vi "FT10_FPGA_7854R Set Relay Config.vi"(10 "Update Config Enum":T1(ring), 11 "Refnum in":refnum<k20>) -> (3 "Refnum out":refnum<k20>)   [LabVIEW 2024]
uses:
  <vilib>/Utility/error.llb/Error Cluster From Error Code.vi
  <vilib>/rvi/errors/niLvFpgaAdjustHostInterfaceError.vi
  <vilib>/rvi/interface/nirviReadWriteControl/nirviReadWriteControl.xnode
  NiFpgaLv.dll
  <vilib>/rvi/interface/Simulation/niFpgaSimulationCallBeginRW.vi
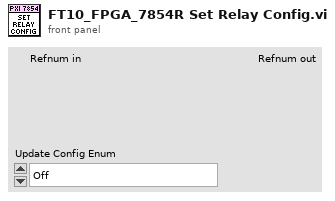
[diagram p1: front panel]
types:
  T1 = enum16{"Off", "Mono1 Relay Config", "Mono2 Relay Config", "Bipolar Relay Config", "Ligasure Relay Config", "Handswitch - Mono1 Cut", "Handswitch - Mono1 Coag", "Handswitch - Mono2 Cut", "Handswitch - Mono2 Coag", "Switch to Triverse Mode", "Switch to Mono2 - 2 button Mode", "Triverse Power 1", "Triverse Power 2", "Triverse Power 3", "Triverse Power 4", "Triverse Power 5", "Handswitch - Triverse Seal", "Handswitch - Triverse Cut", "Handswitch - Triverse Coag"}
  T2 = cluster{"Conn2/DIO_0_7 In":cluster{"Conn2/DIO_0_7 - 75kHz":bool, "Conn2/DIO_0_7 - uSec On":u16, "Conn2/DIO_0_7 In":bool[], "Conn2/DIO_0_7 - uSec Off":u16}, "Conn2/DIO_8_15 In":cluster{"Conn2/DIO_8_15 - 75kHz":bool, "Conn2/DIO_8_15 - uSec On":u16, "Conn2/DIO_8_15 In":bool[], "Conn2/DIO_8_15 - uSec Off":u16}, "Conn2/DIO_16_23 In":cluster{"Conn2/DIO_16_23 - 75kHz":bool, "Conn2/DIO_16_23 - uSec On":u16, "Conn2/DIO_16_23 In":bool[], "Conn2/DIO_16_23 - uSec Off":u16}, "Conn2/DIO_24_31 In":cluster{"Conn2/DIO_24_31 - 75kHz":bool, "Conn2/DIO_24_31 - uSec On":u16, "Conn2/DIO_24_31 In":bool[], "Conn2/DIO_24_31 - uSec Off":u16}, "Conn2/DIO_32_39 In":cluster{"Conn2/DIO_32_39 - 75kHz":bool, "Conn2/DIO_32_39 - uSec On":u16, "Conn2/DIO_32_39 In":bool[], "Conn2/DIO_32_39 - uSec Off":u16}}
  T3 = cluster{"Conn1/DIO_0_7 In":cluster{"Conn1/DIO_0_7 - 75kHz":bool, "Conn1/DIO_0_7 - uSec On":u16, "Conn1/DIO_0_7 In":bool[], "Conn1/DIO_0_7 - uSec Off":u16}, "Conn1/DIO_8_15 In":cluster{"Conn1/DIO_8_15 - 75kHz":bool, "Conn1/DIO_8_15 - uSec On":u16, "Conn1/DIO_8_15 In":bool[], "Conn1/DIO_8_15 - uSec Off":u16}, "Conn1/DIO_16_23 In":cluster{"Conn1/DIO_16_23 - 75kHz":bool, "Conn1/DIO_16_23 - uSec On":u16, "Conn1/DIO_16_23 In":bool[], "Conn1/DIO_16_23 - uSec Off":u16}, "Conn1/DIO_24_31 In":cluster{"Conn1/DIO_24_31 - 75kHz":bool, "Conn1/DIO_24_31 - uSec On":u16, "Conn1/DIO_24_31 In":bool[], "Conn1/DIO_24_31 - uSec Off":u16}, "Conn1/DIO_32_39 In":cluster{"Conn1/DIO_32_39 - 75kHz":bool, "Conn1/DIO_32_39 - uSec On":u16, "Conn1/DIO_32_39 In":bool[], "Conn1/DIO_32_39 - uSec Off":u16}}
  T4 = cluster{"Conn0/DIO_0_7 In":cluster{"Conn0/DIO_0_7 - 75kHz":bool, "Conn0/DIO_0_7 - uSec On":u16, "Conn0/DIO_0_7 In":bool[], "Conn0/DIO_0_7 - uSec Off":u16}, "Conn0/DIO_8_15 In":cluster{"Conn0/DIO_8_15 - 75kHz":bool, "Conn0/DIO_8_15 - uSec On":u16, "Conn0/DIO_8_15 In":bool[], "Conn0/DIO_8_15 - uSec Off":u16}}
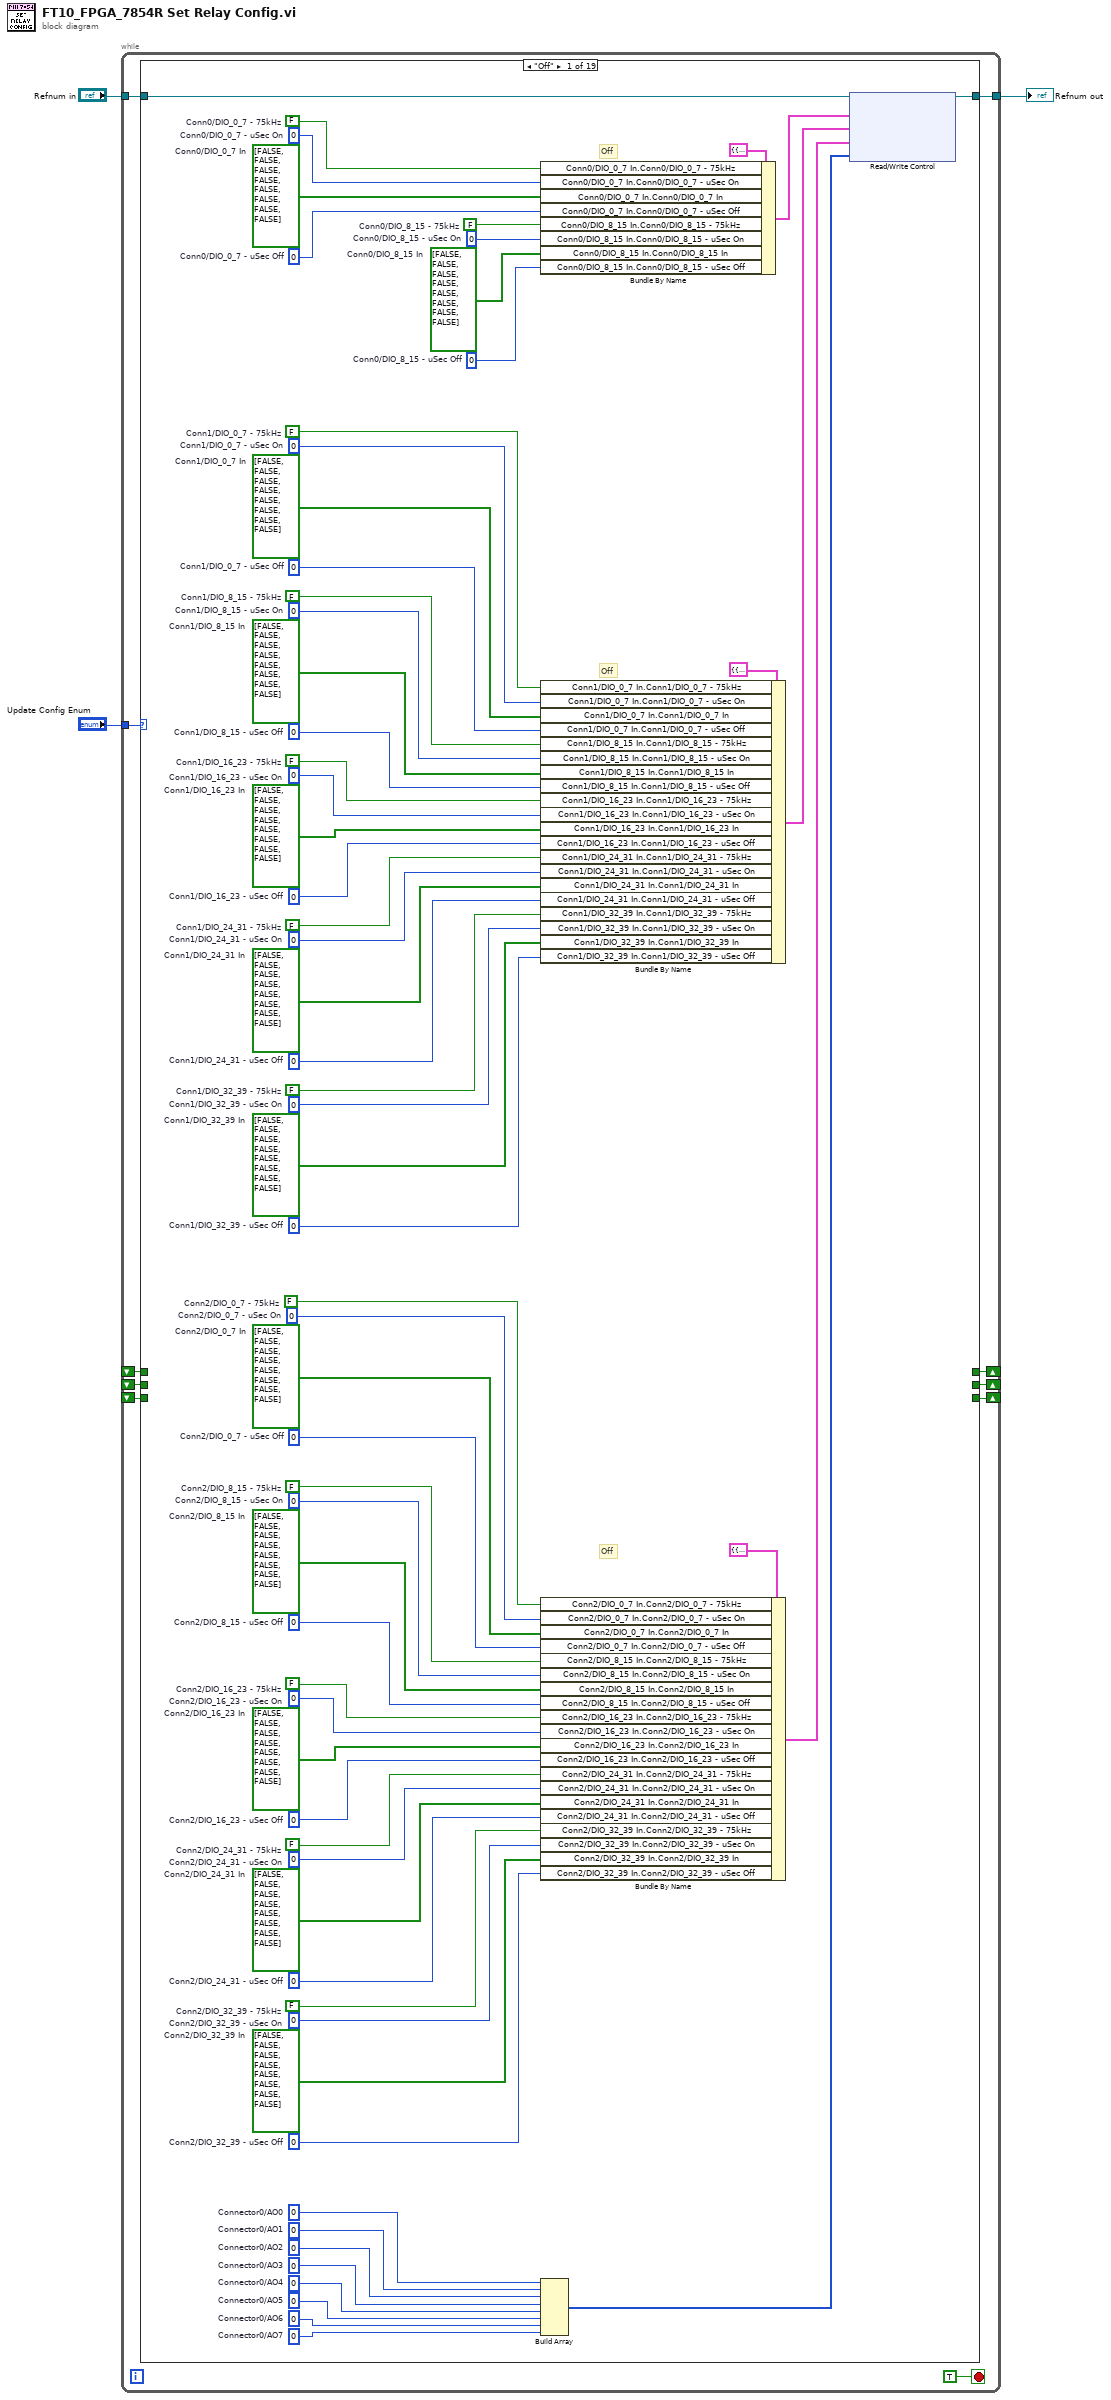
[diagram p0: block diagram]
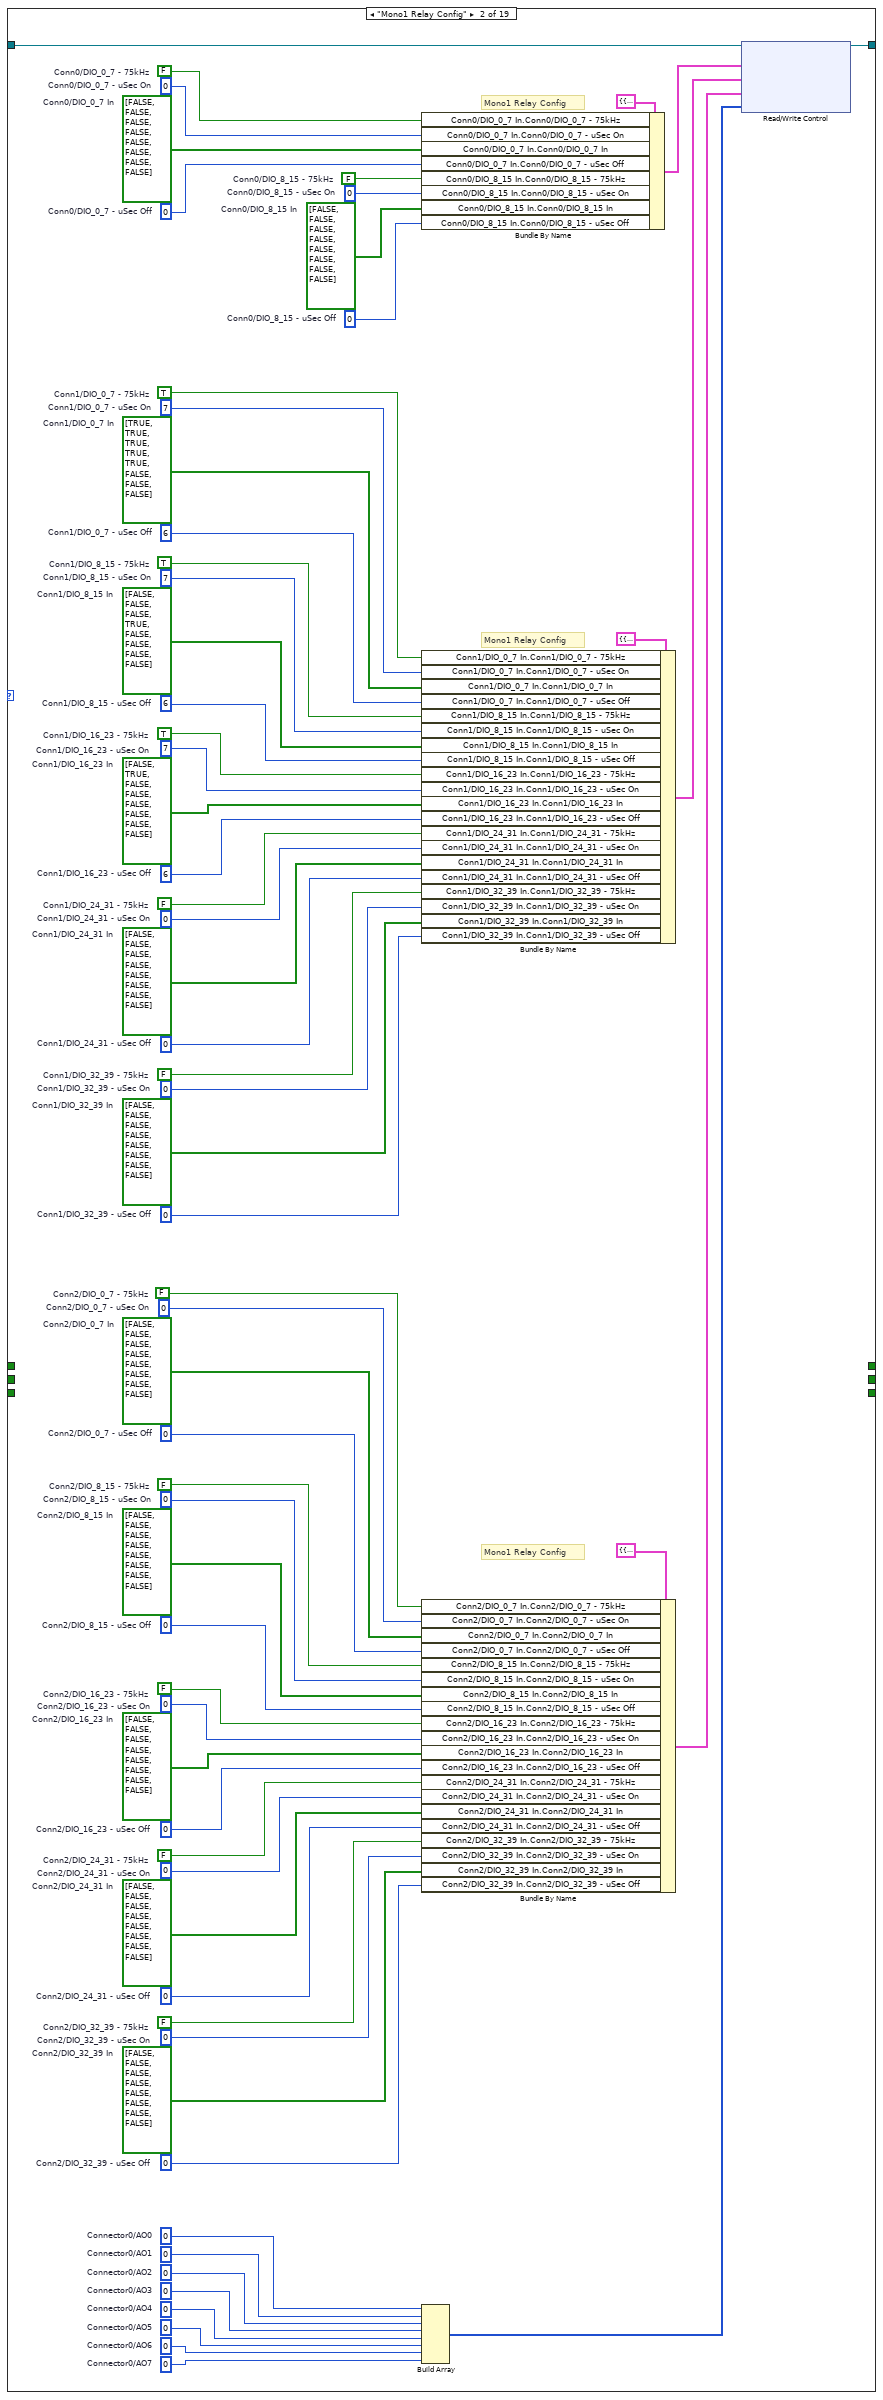
[diagram p2: hidden frame]
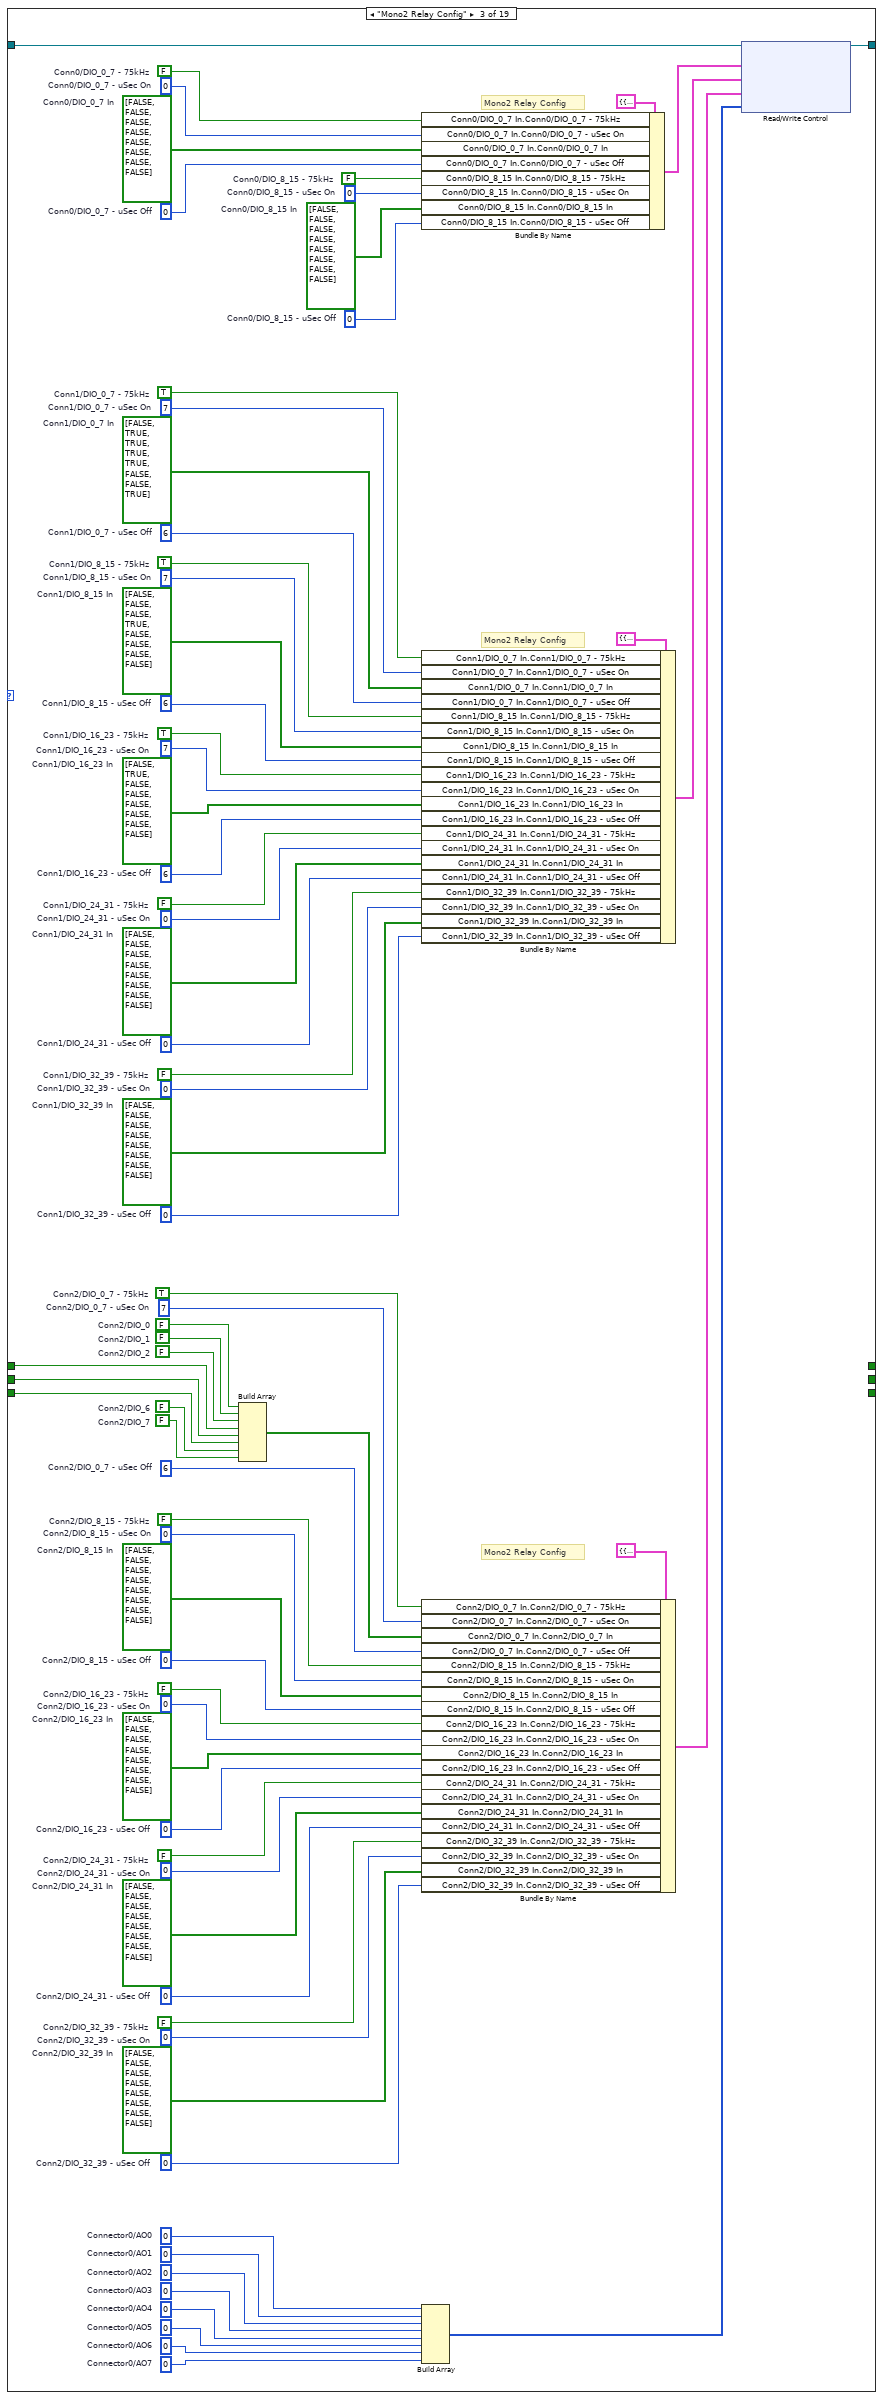
[diagram p3: hidden frame]
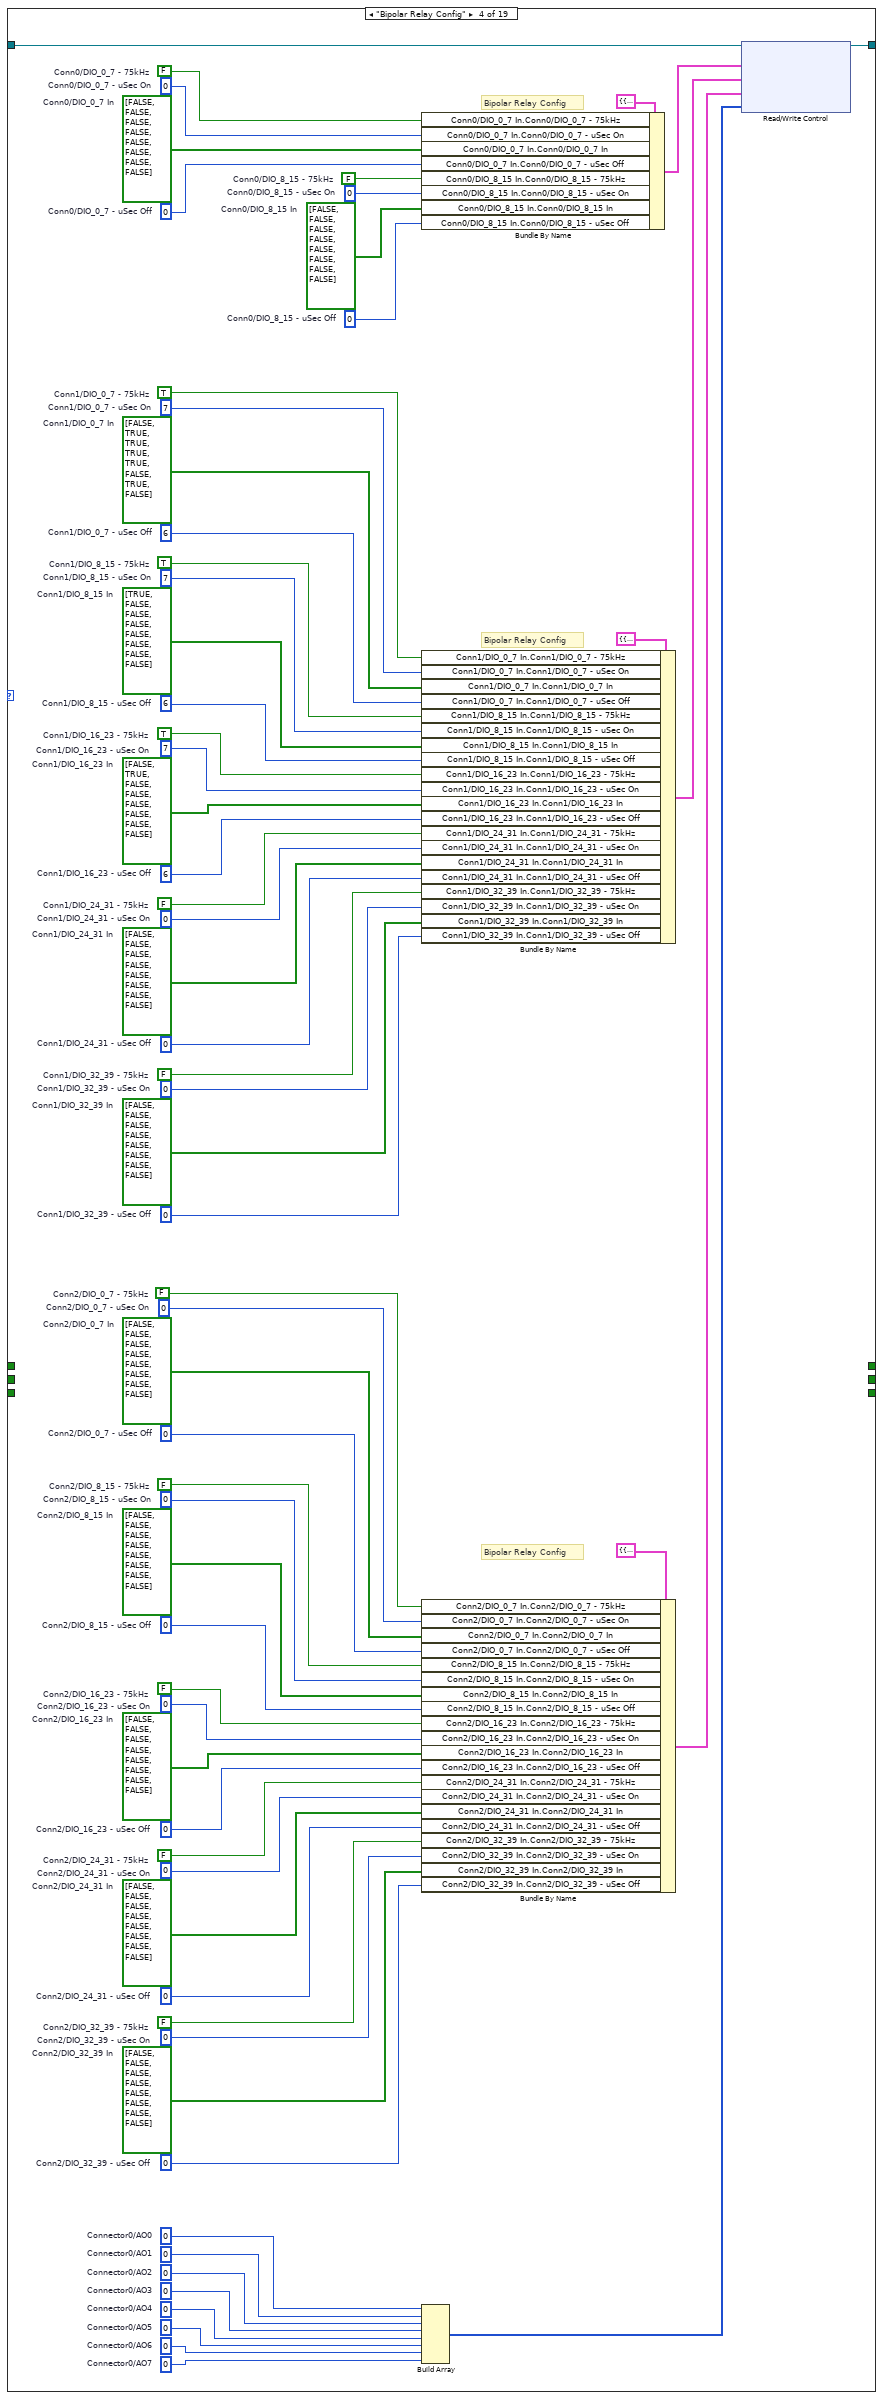
[diagram p4: hidden frame]
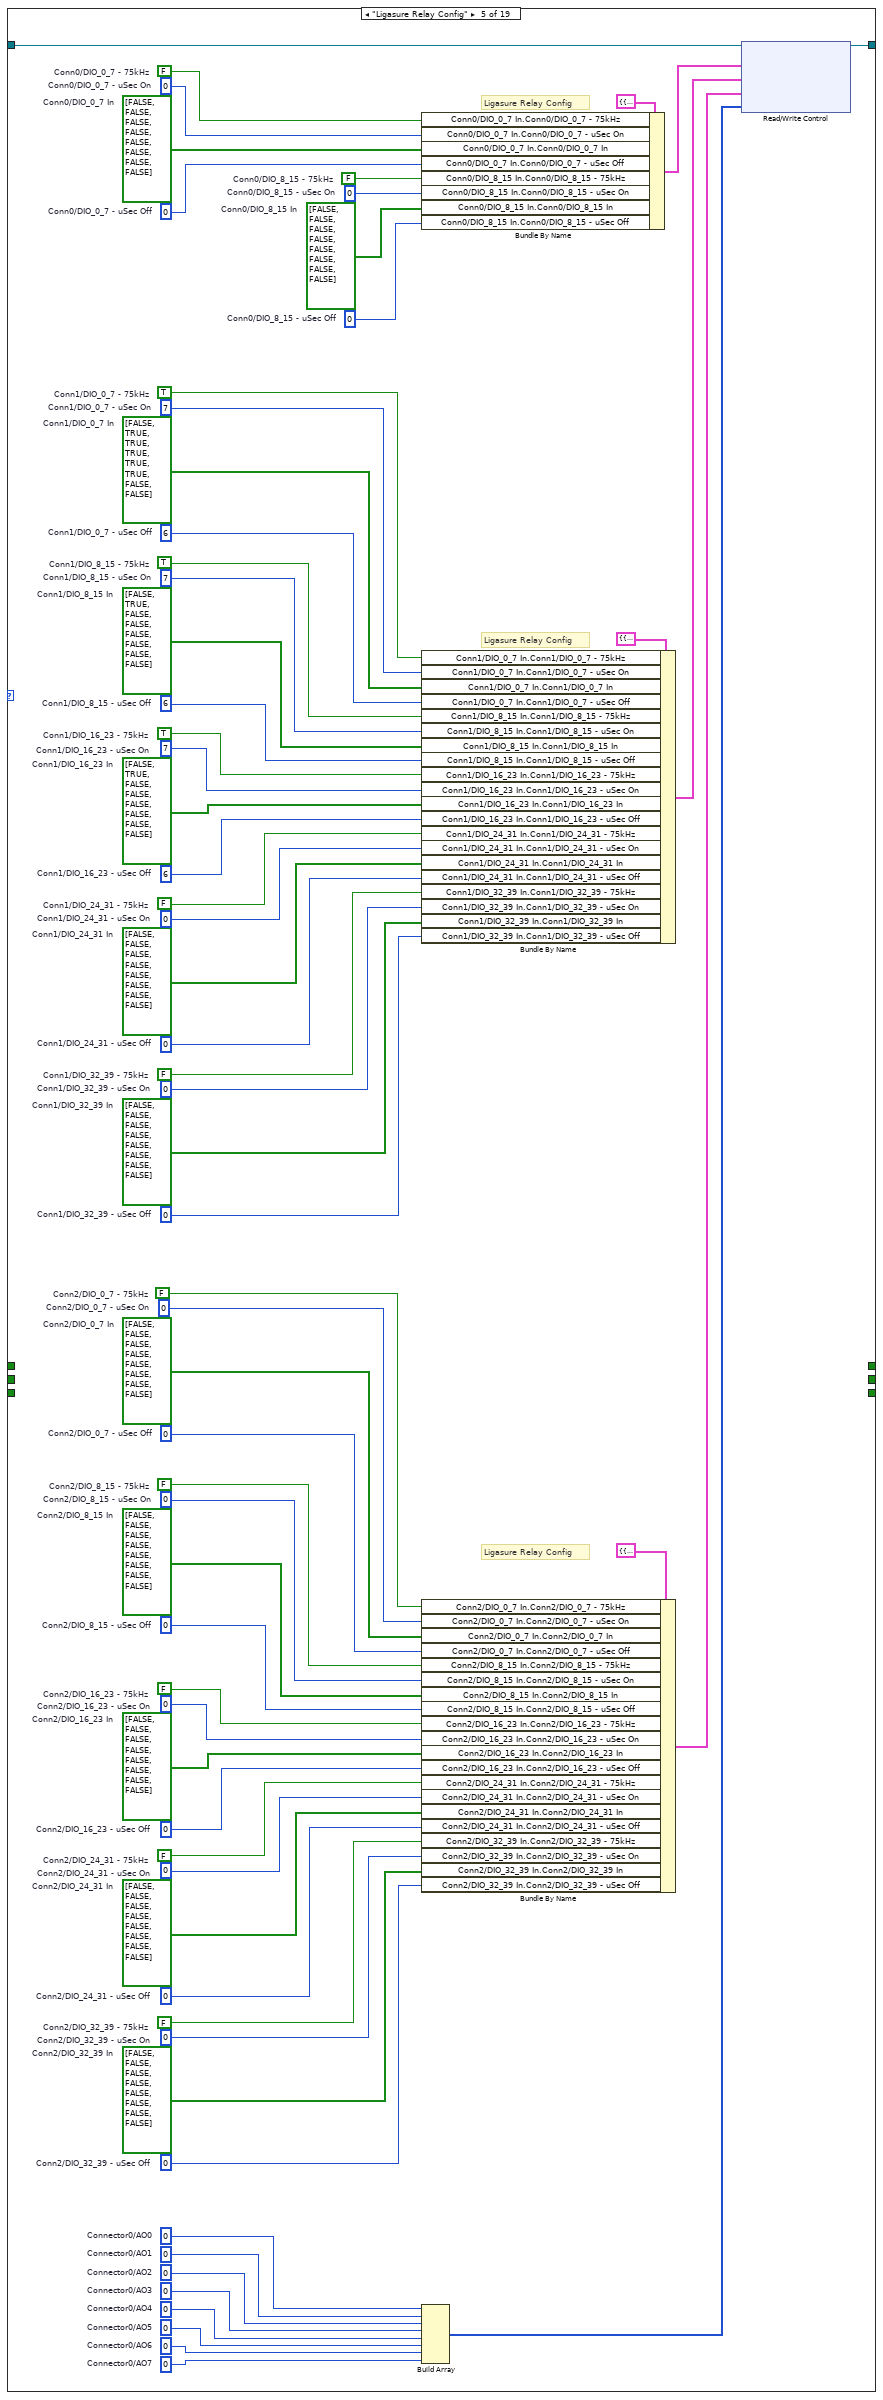
[diagram p5: hidden frame]
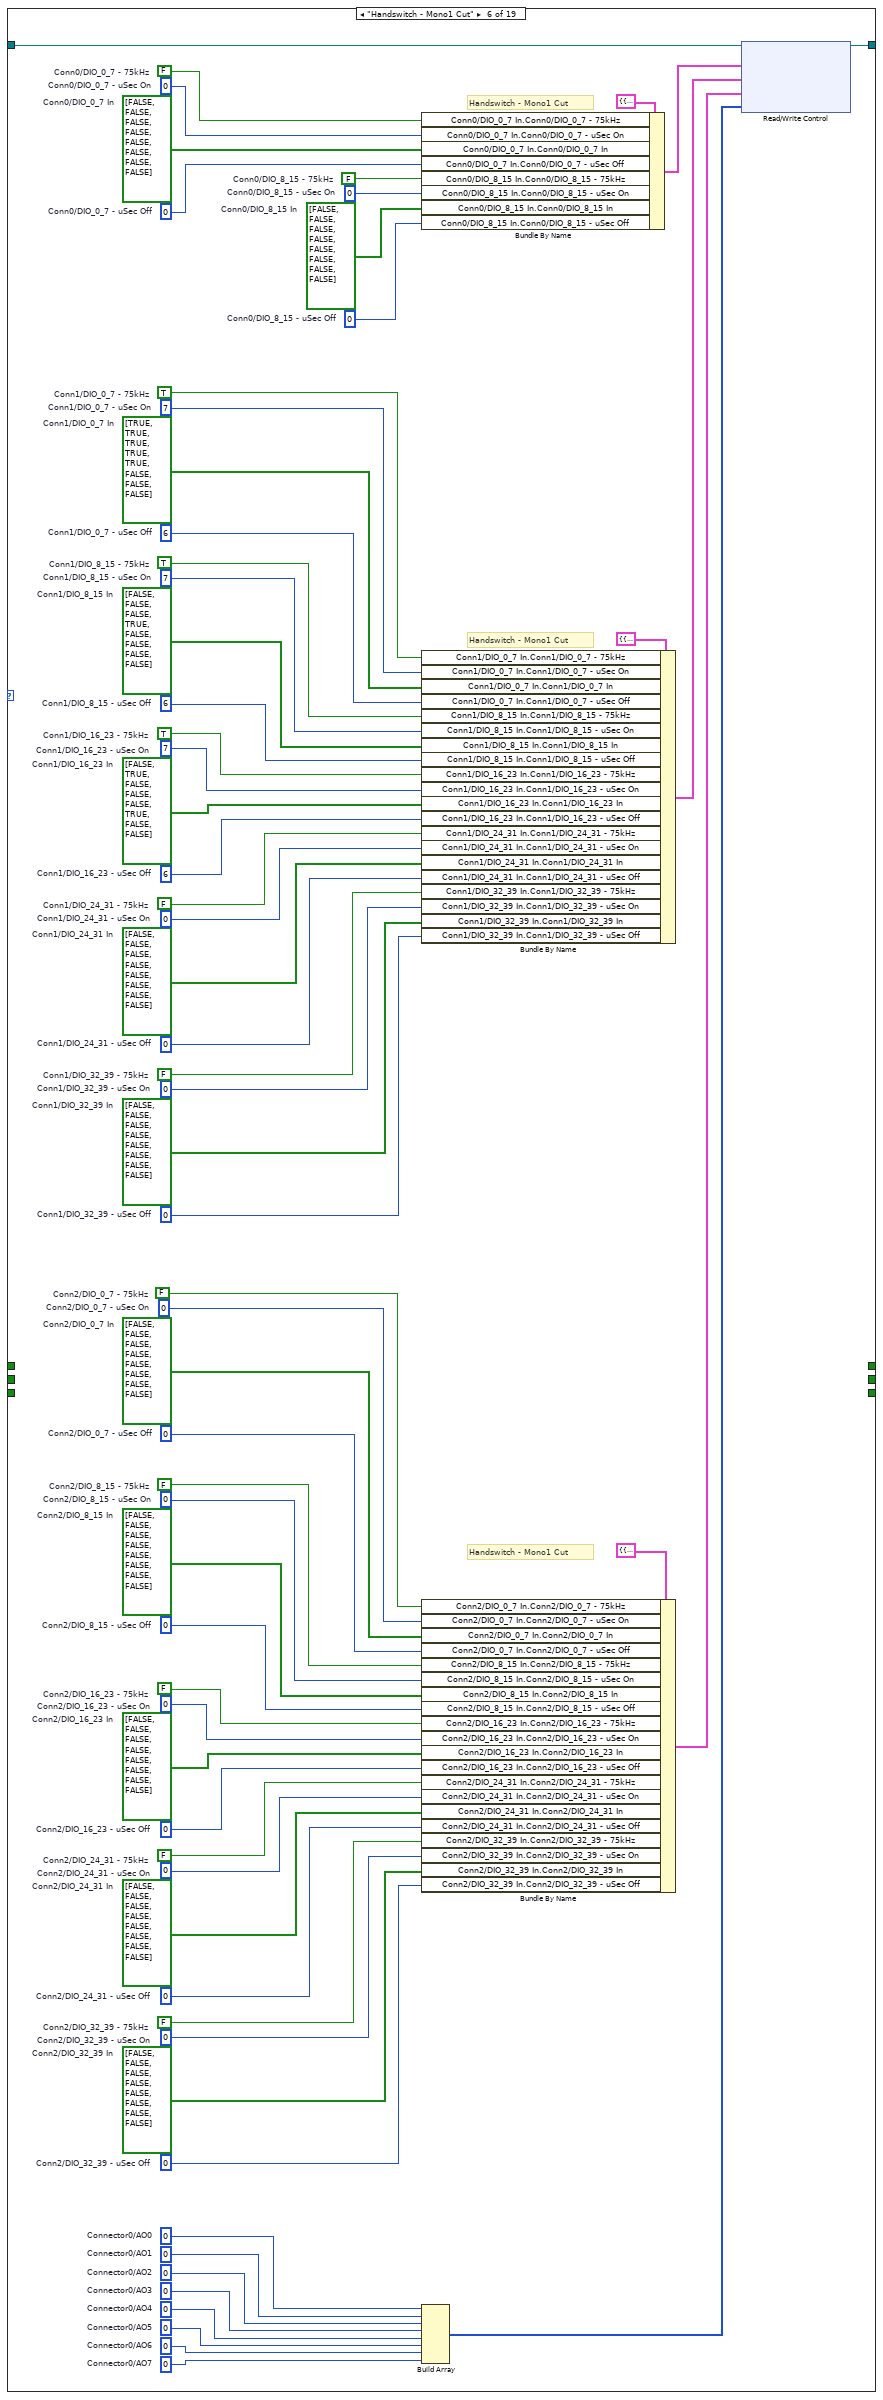
[diagram p6: hidden frame]
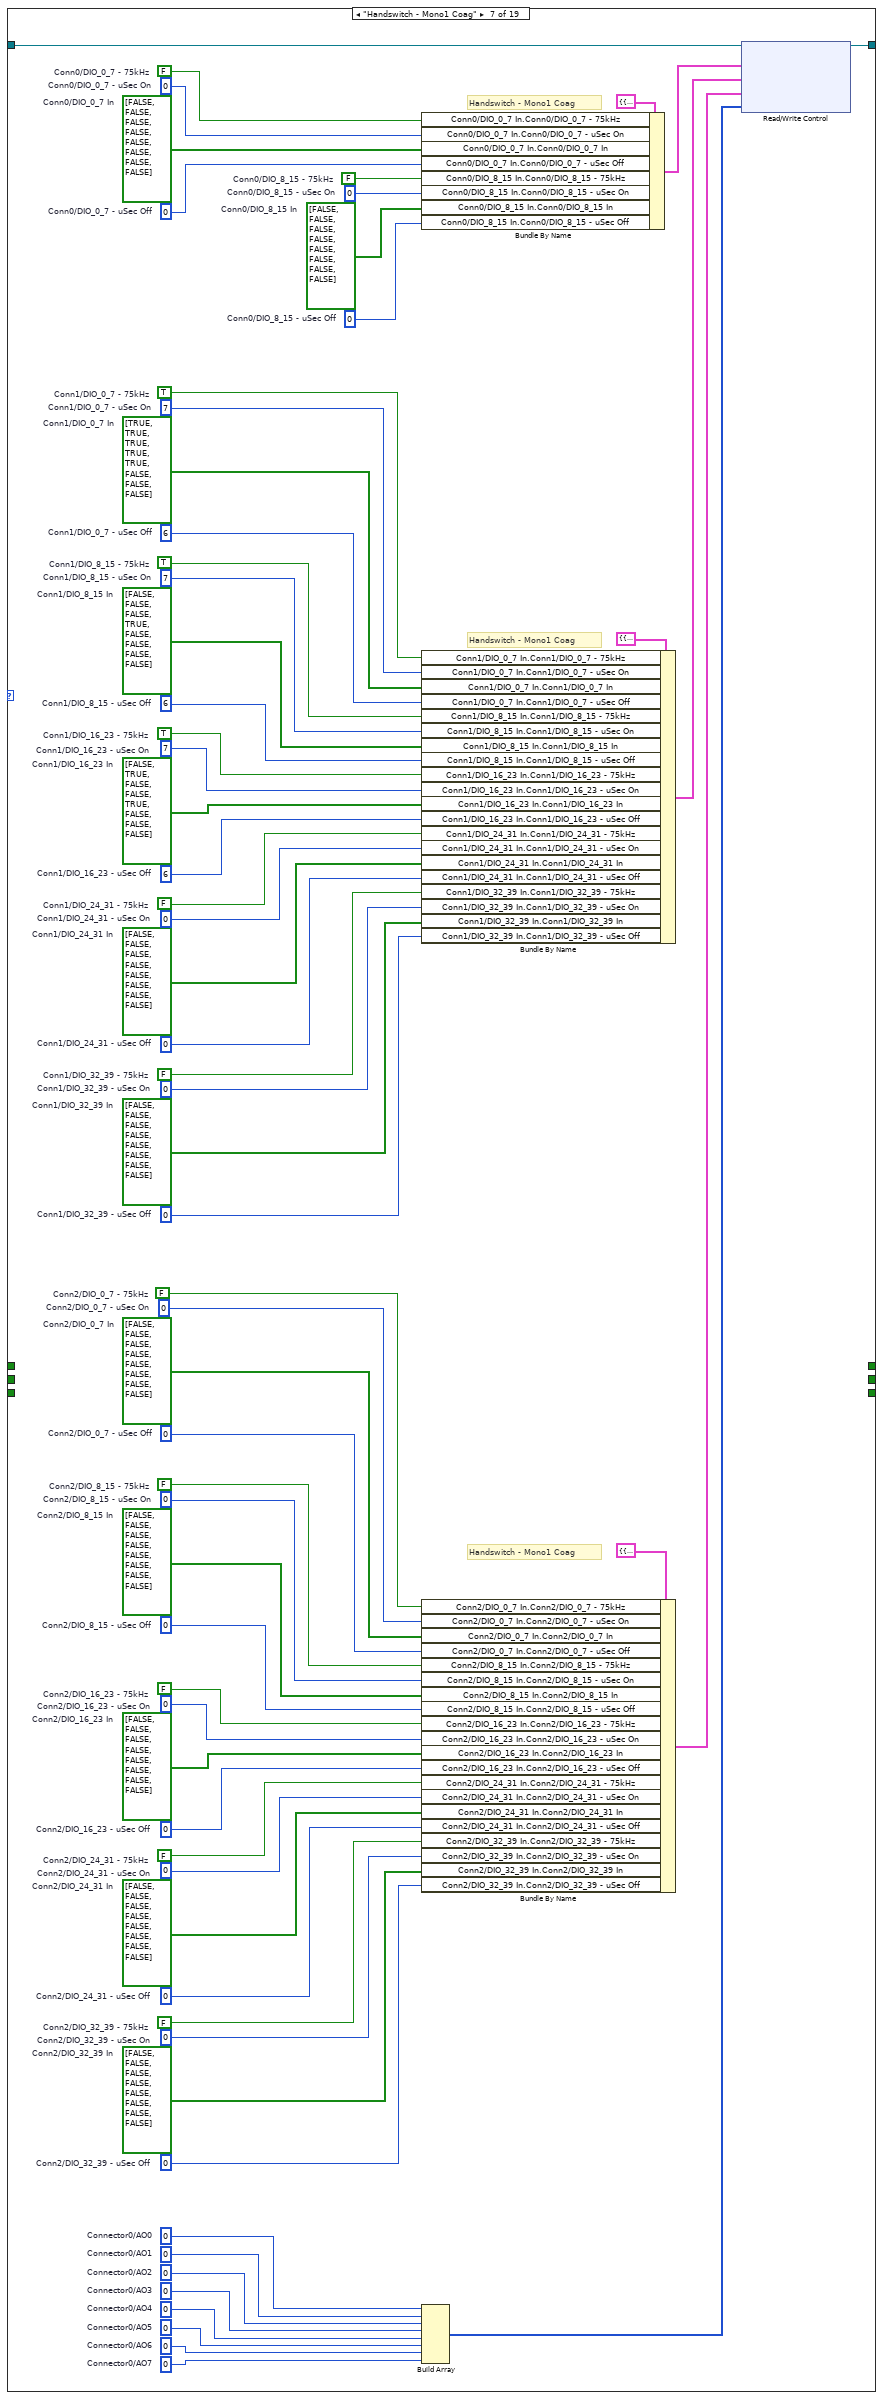
[diagram p7: hidden frame]
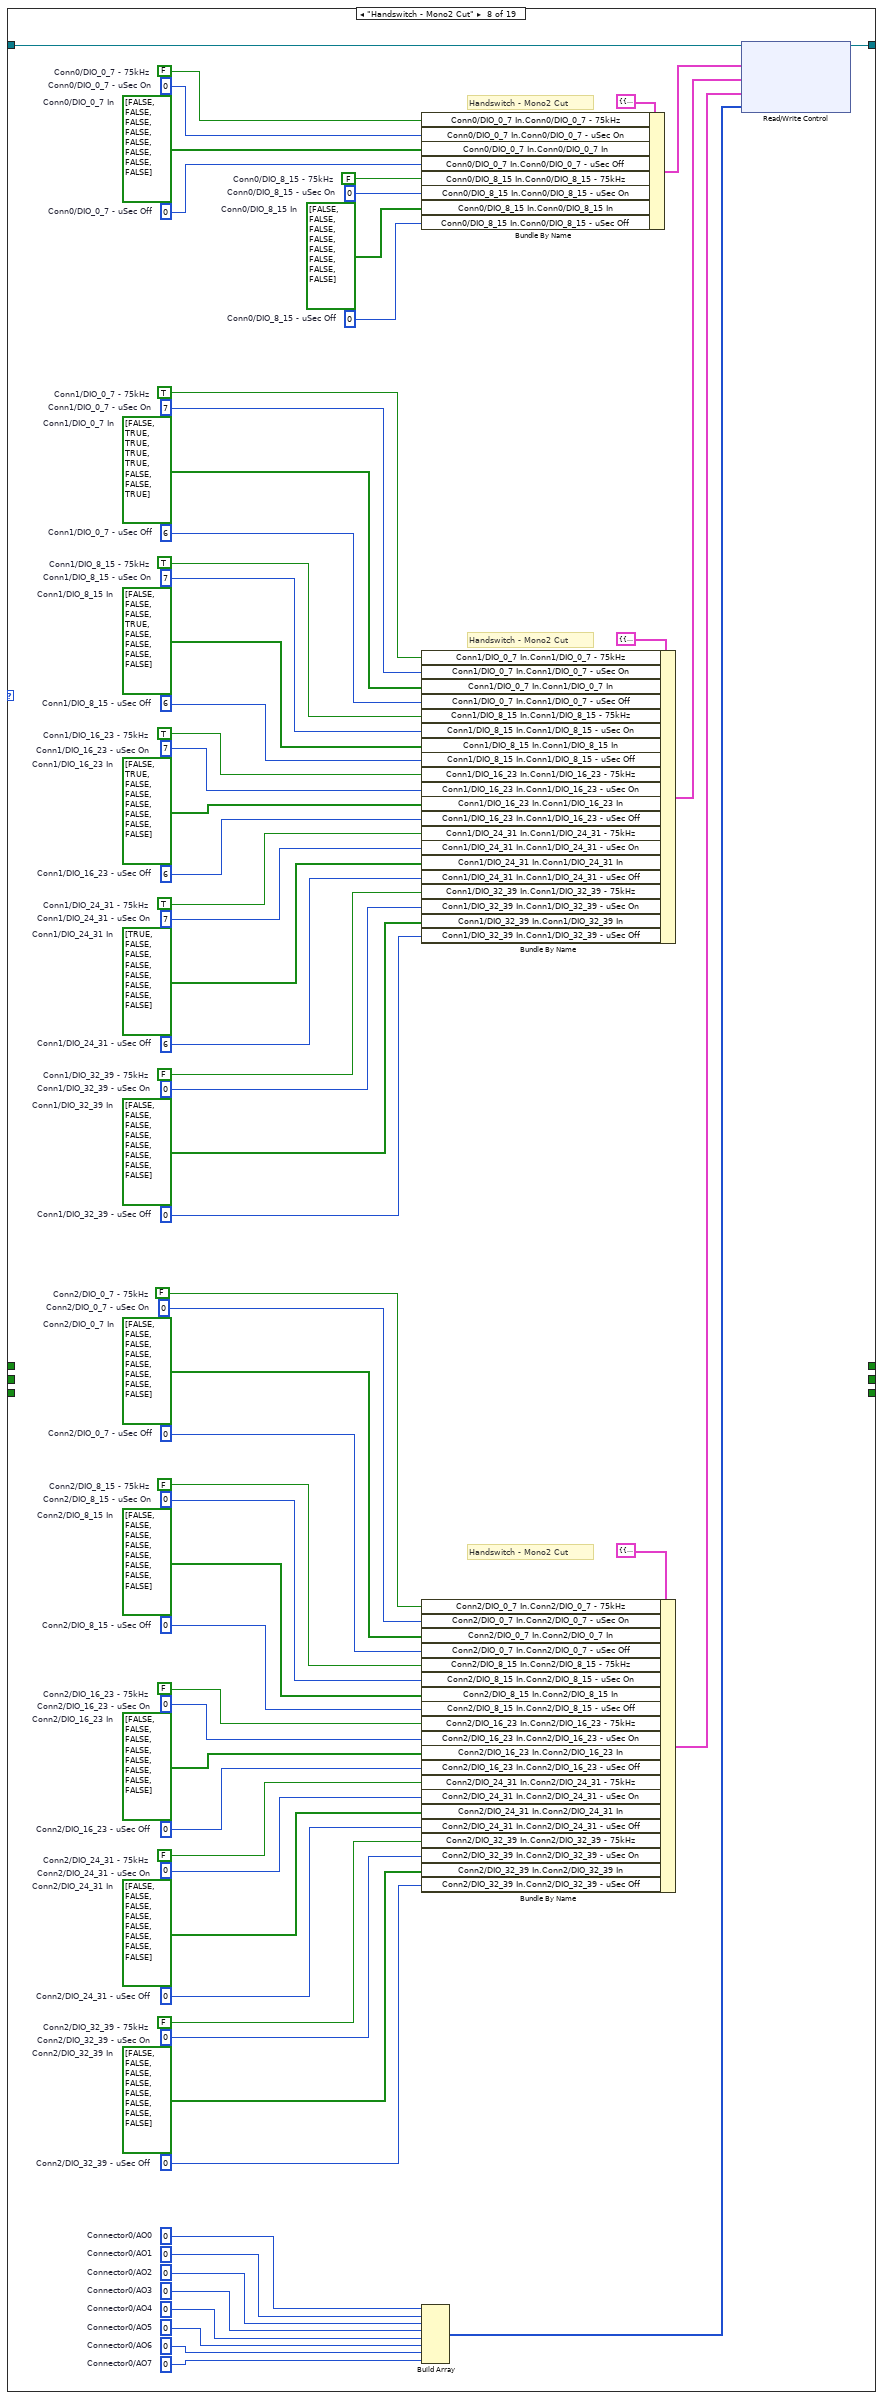
[diagram p8: hidden frame]
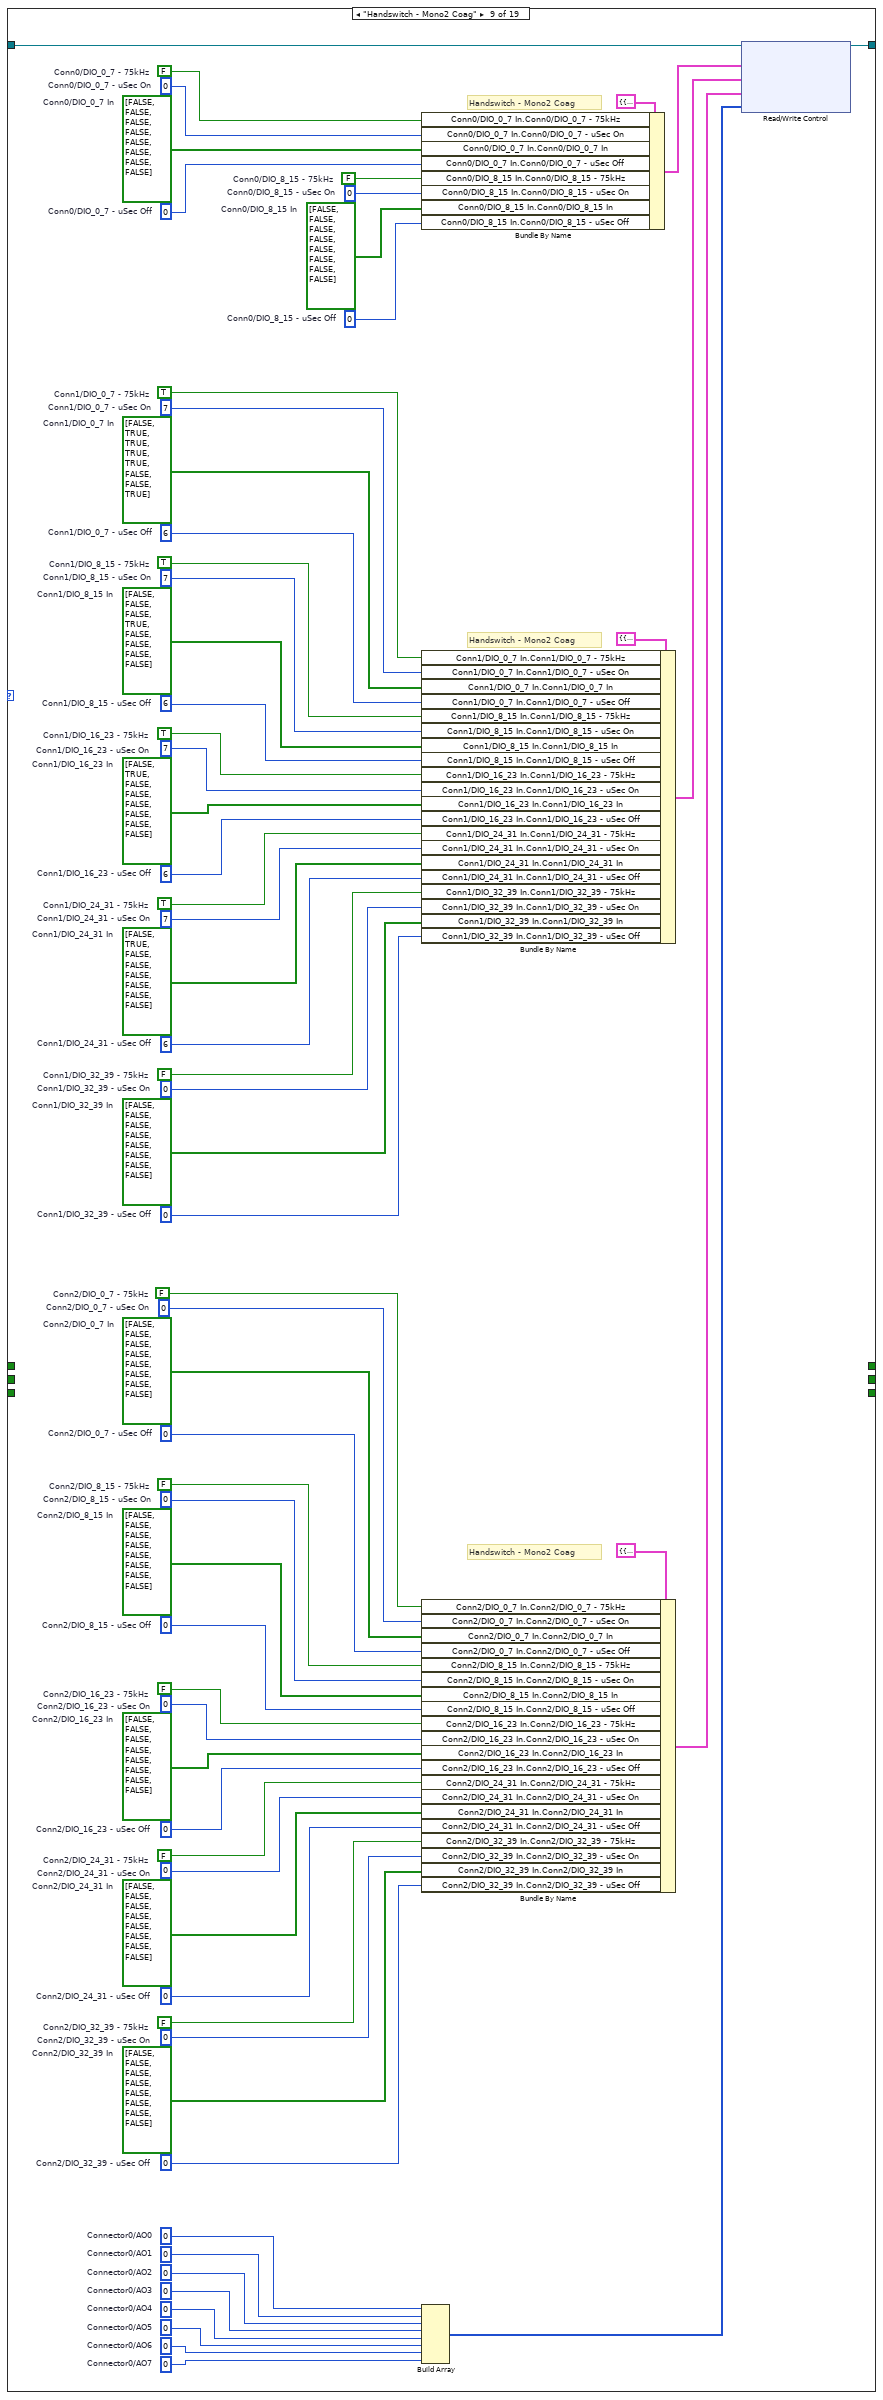
[diagram p9: hidden frame]
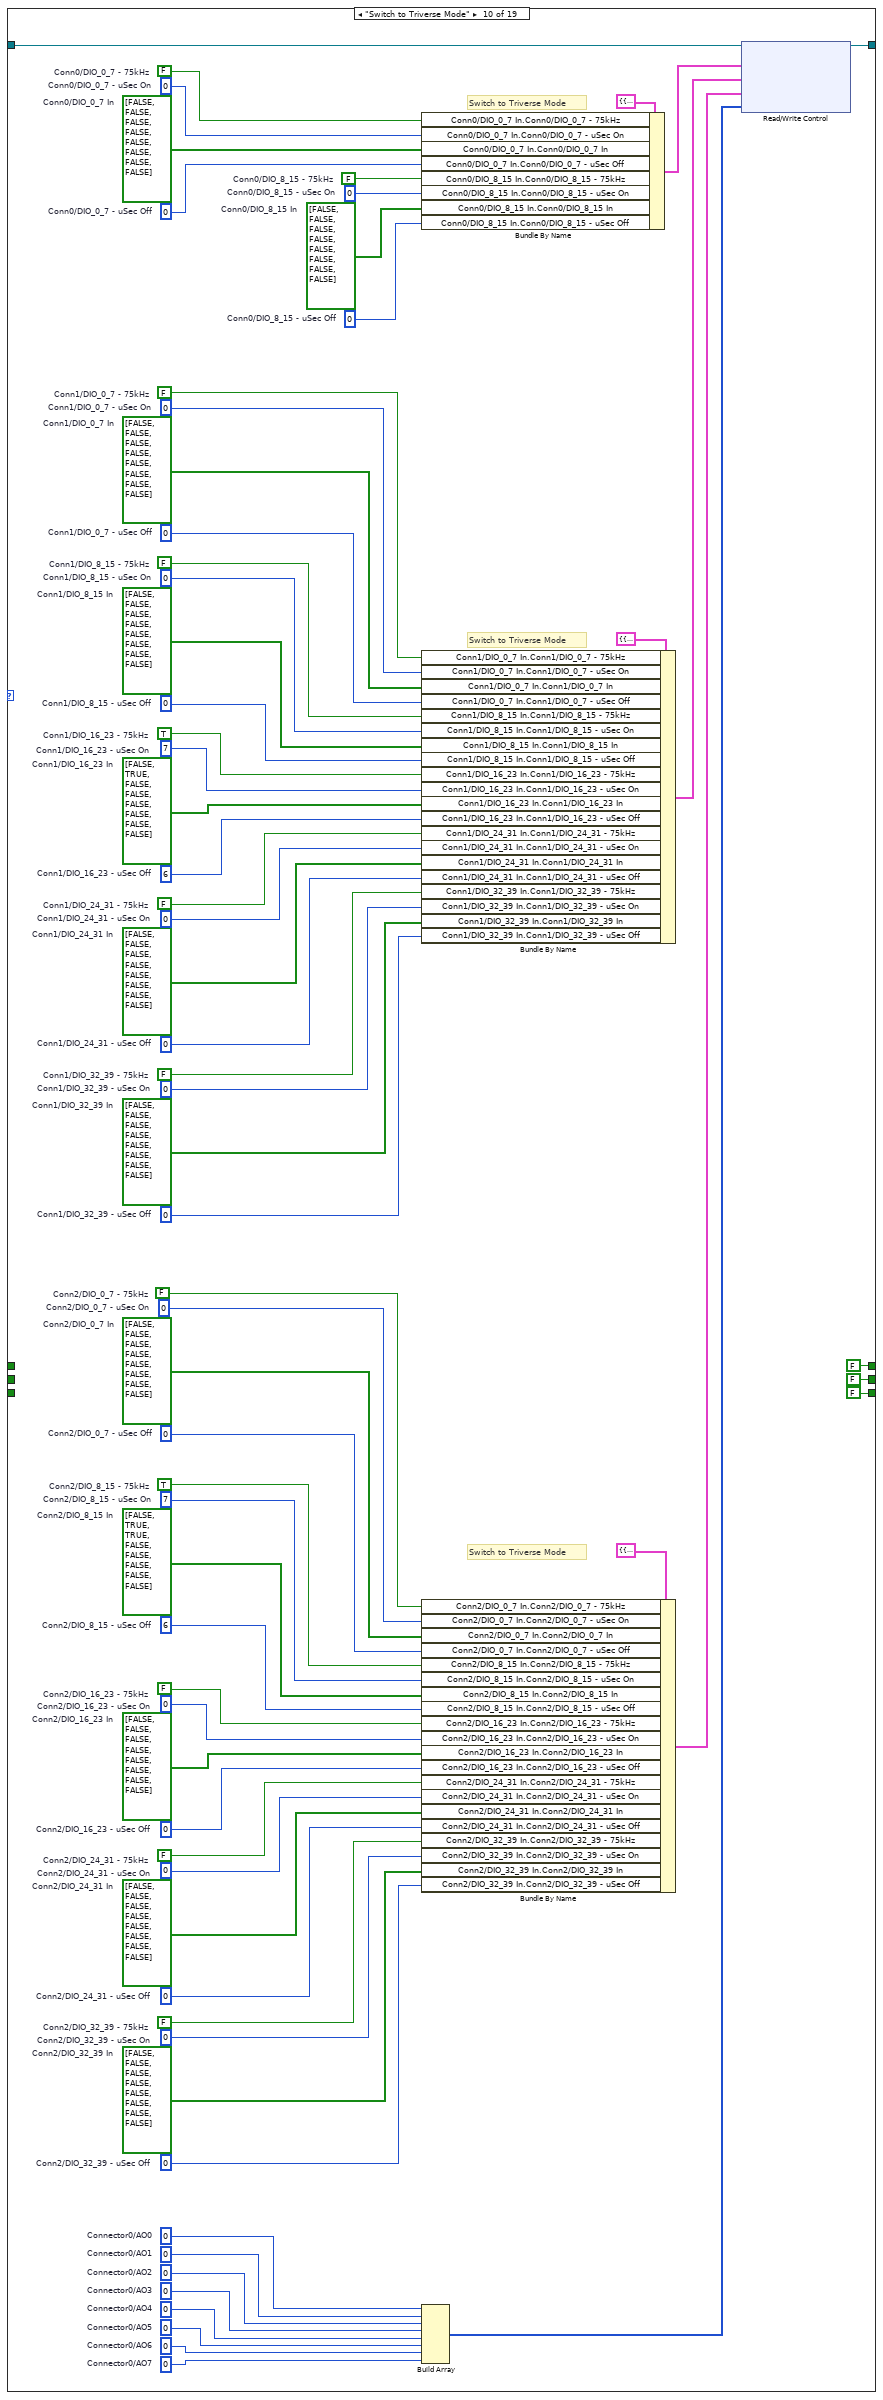
[diagram p10: hidden frame]
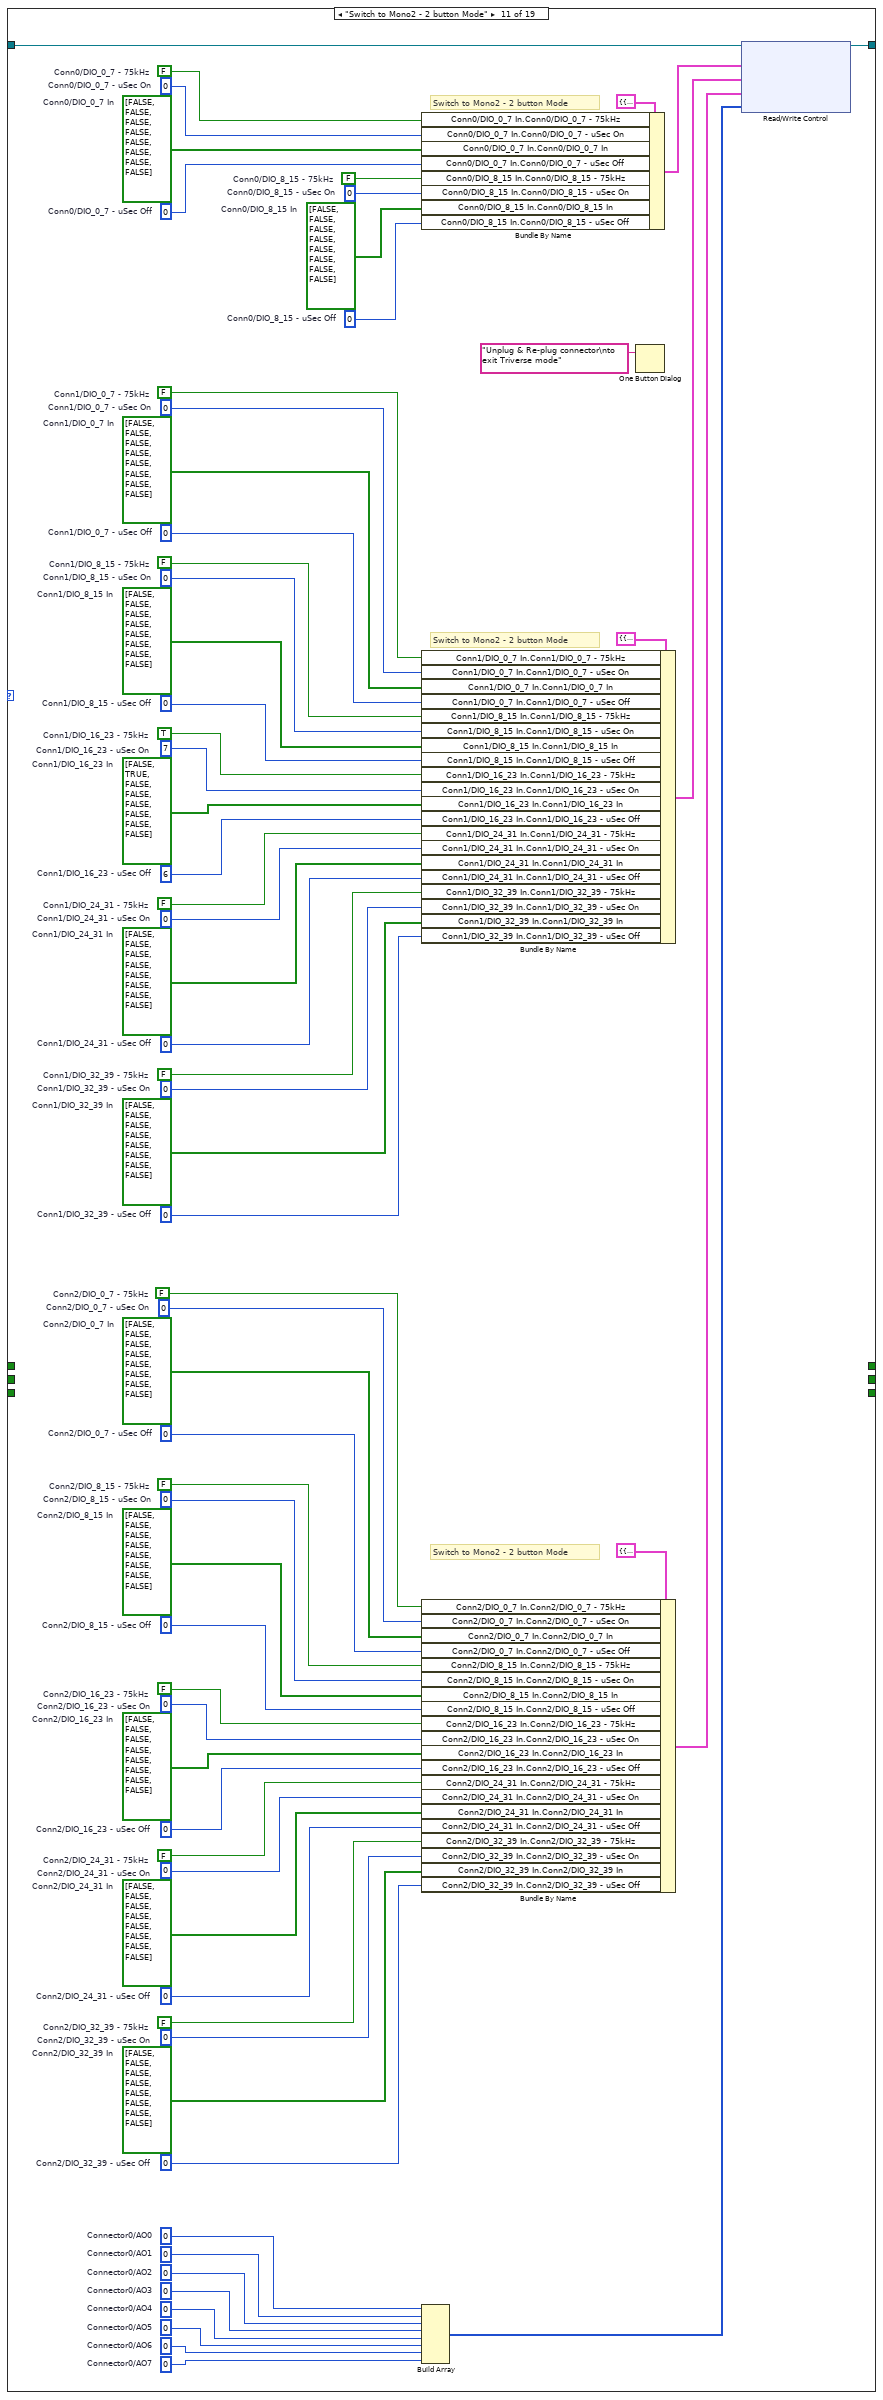
[diagram p11: hidden frame]
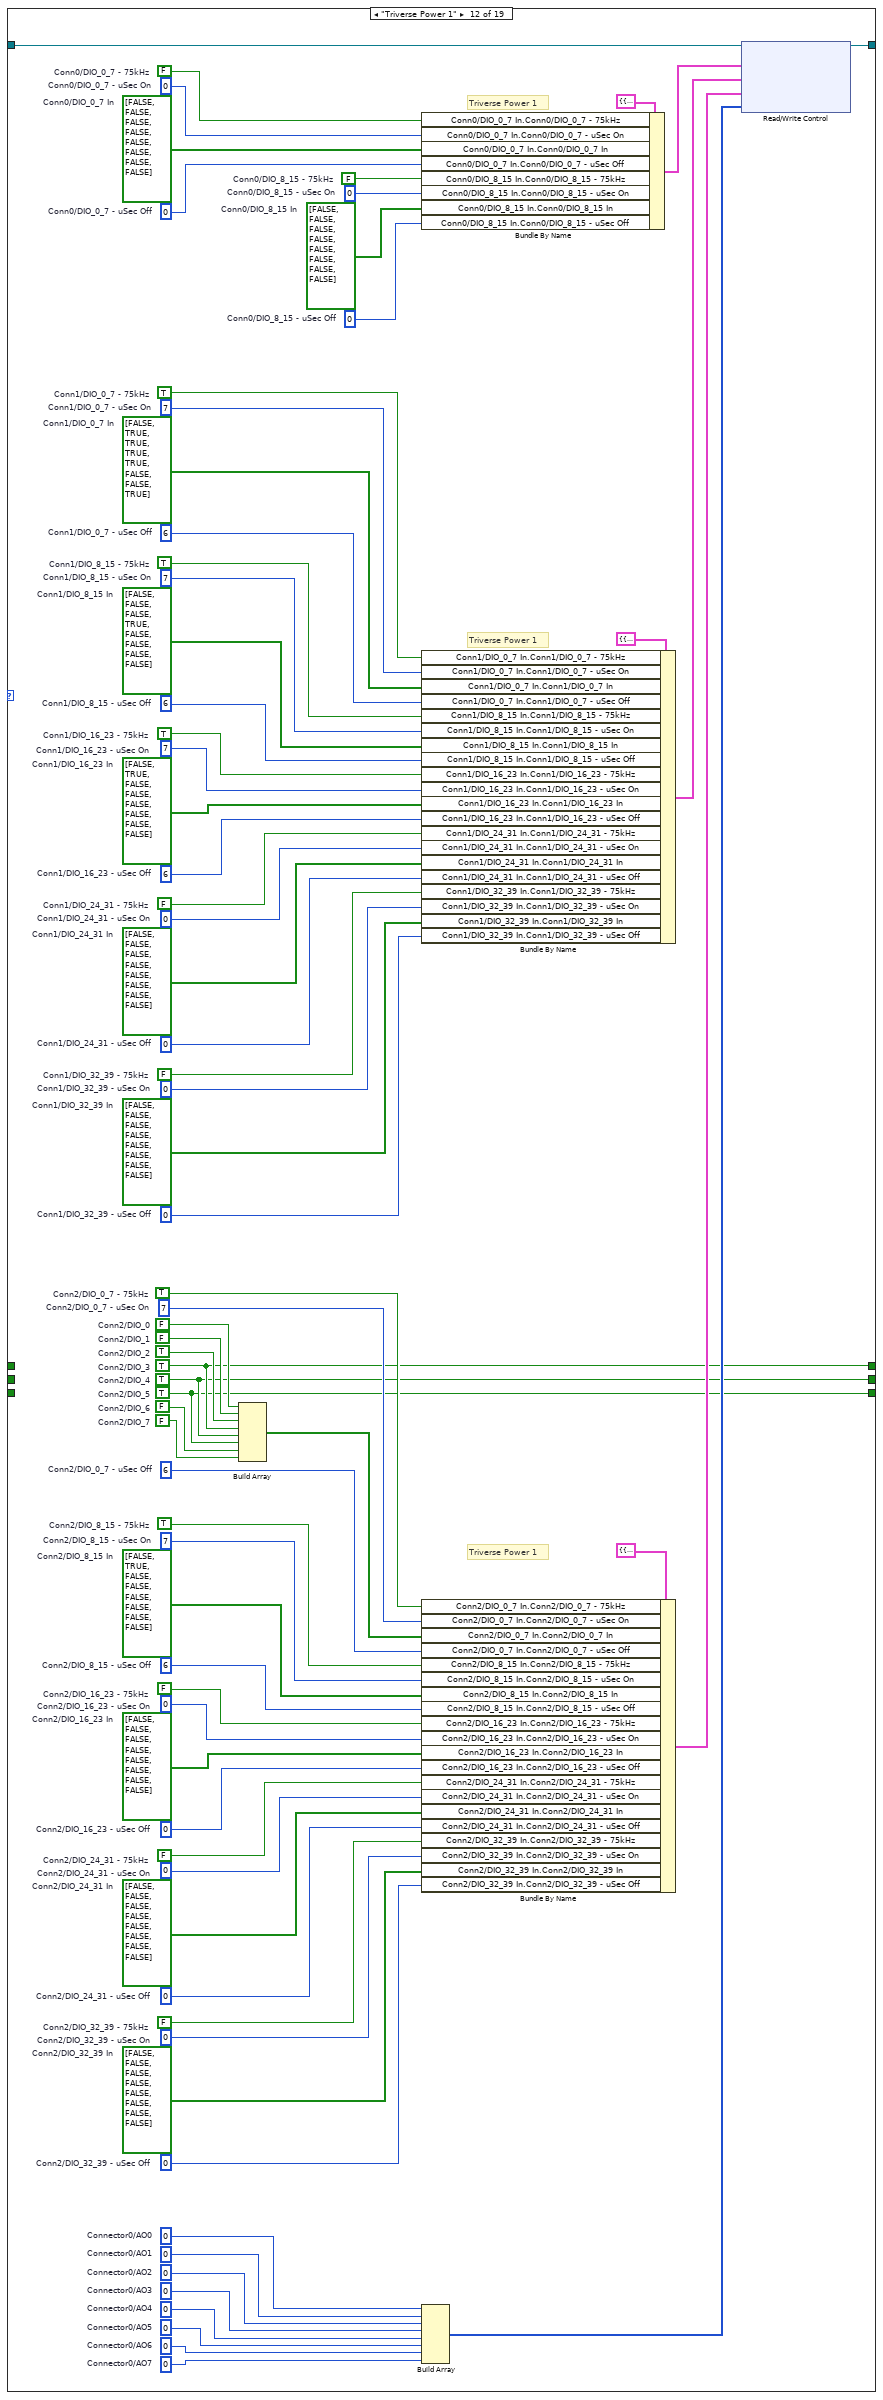
[diagram p12: hidden frame]
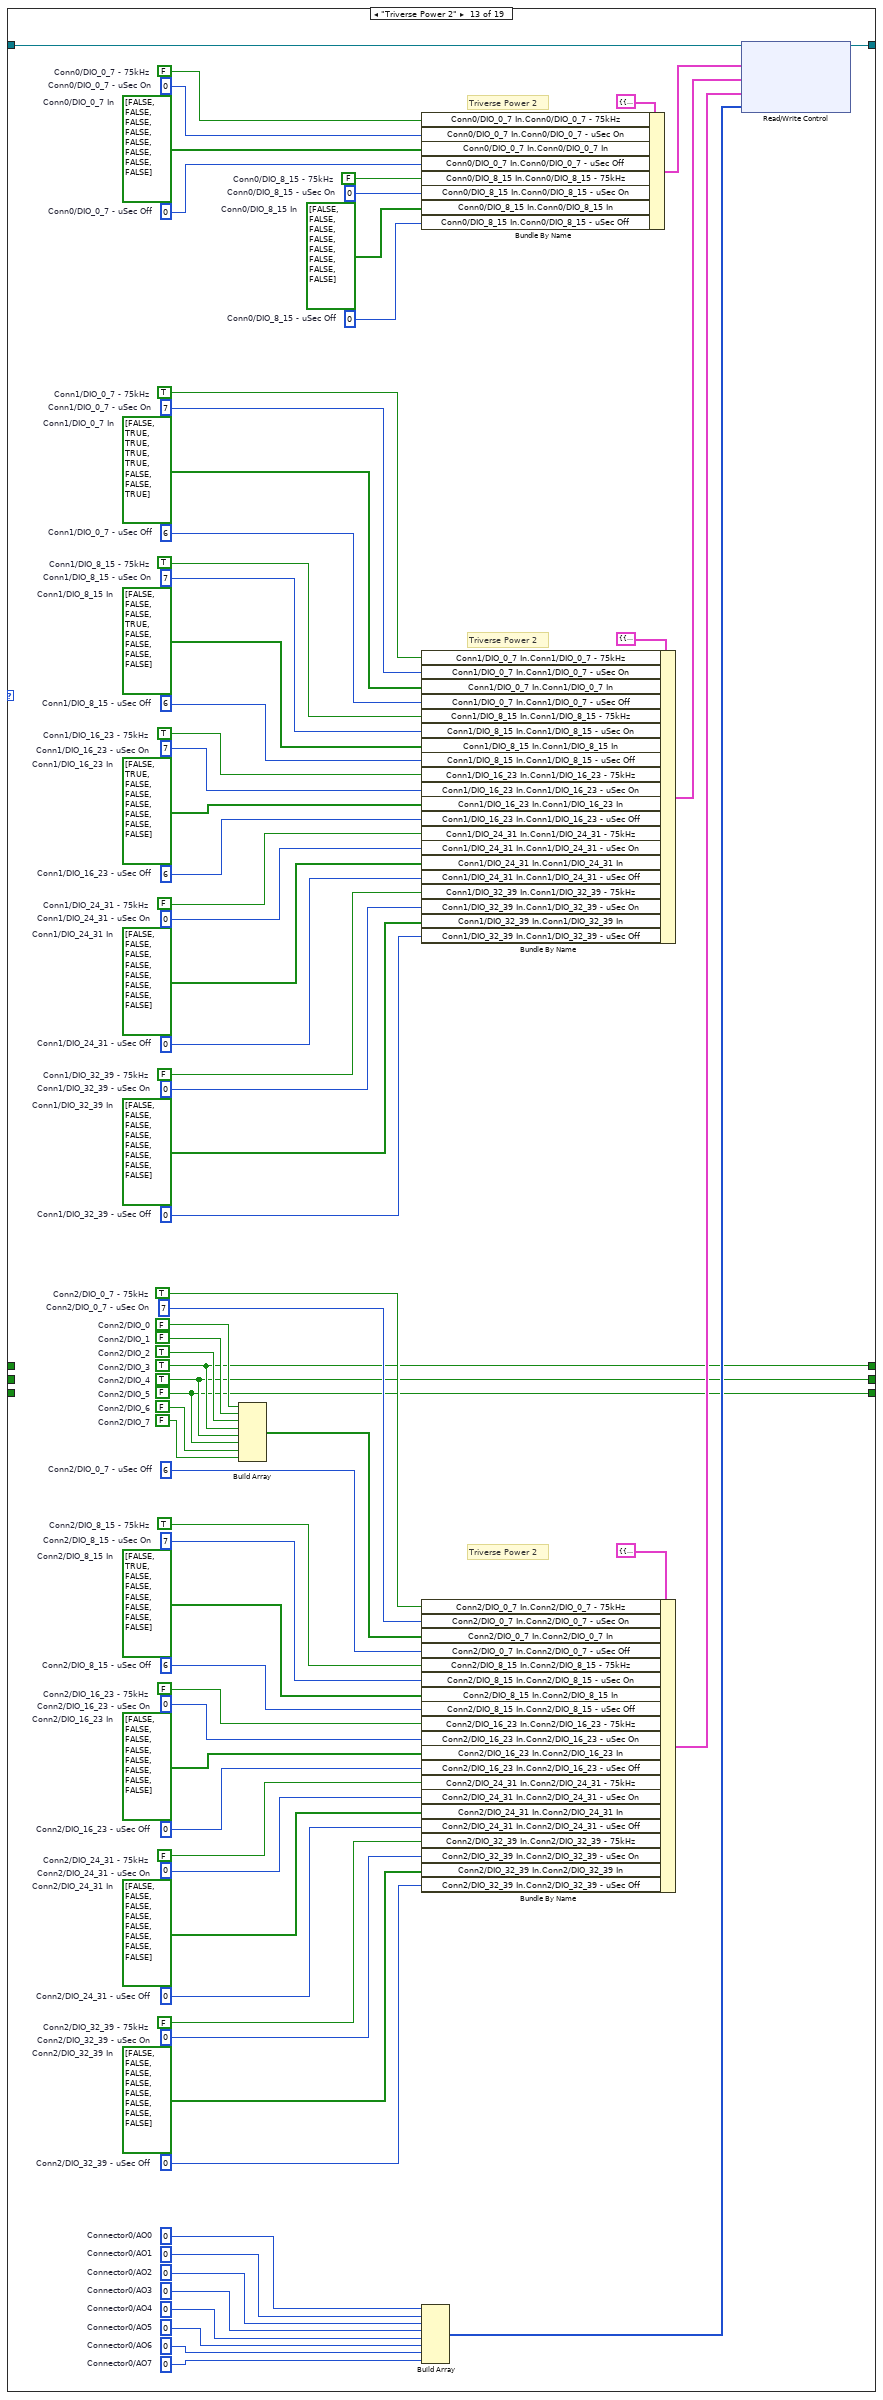
[diagram p13: hidden frame]
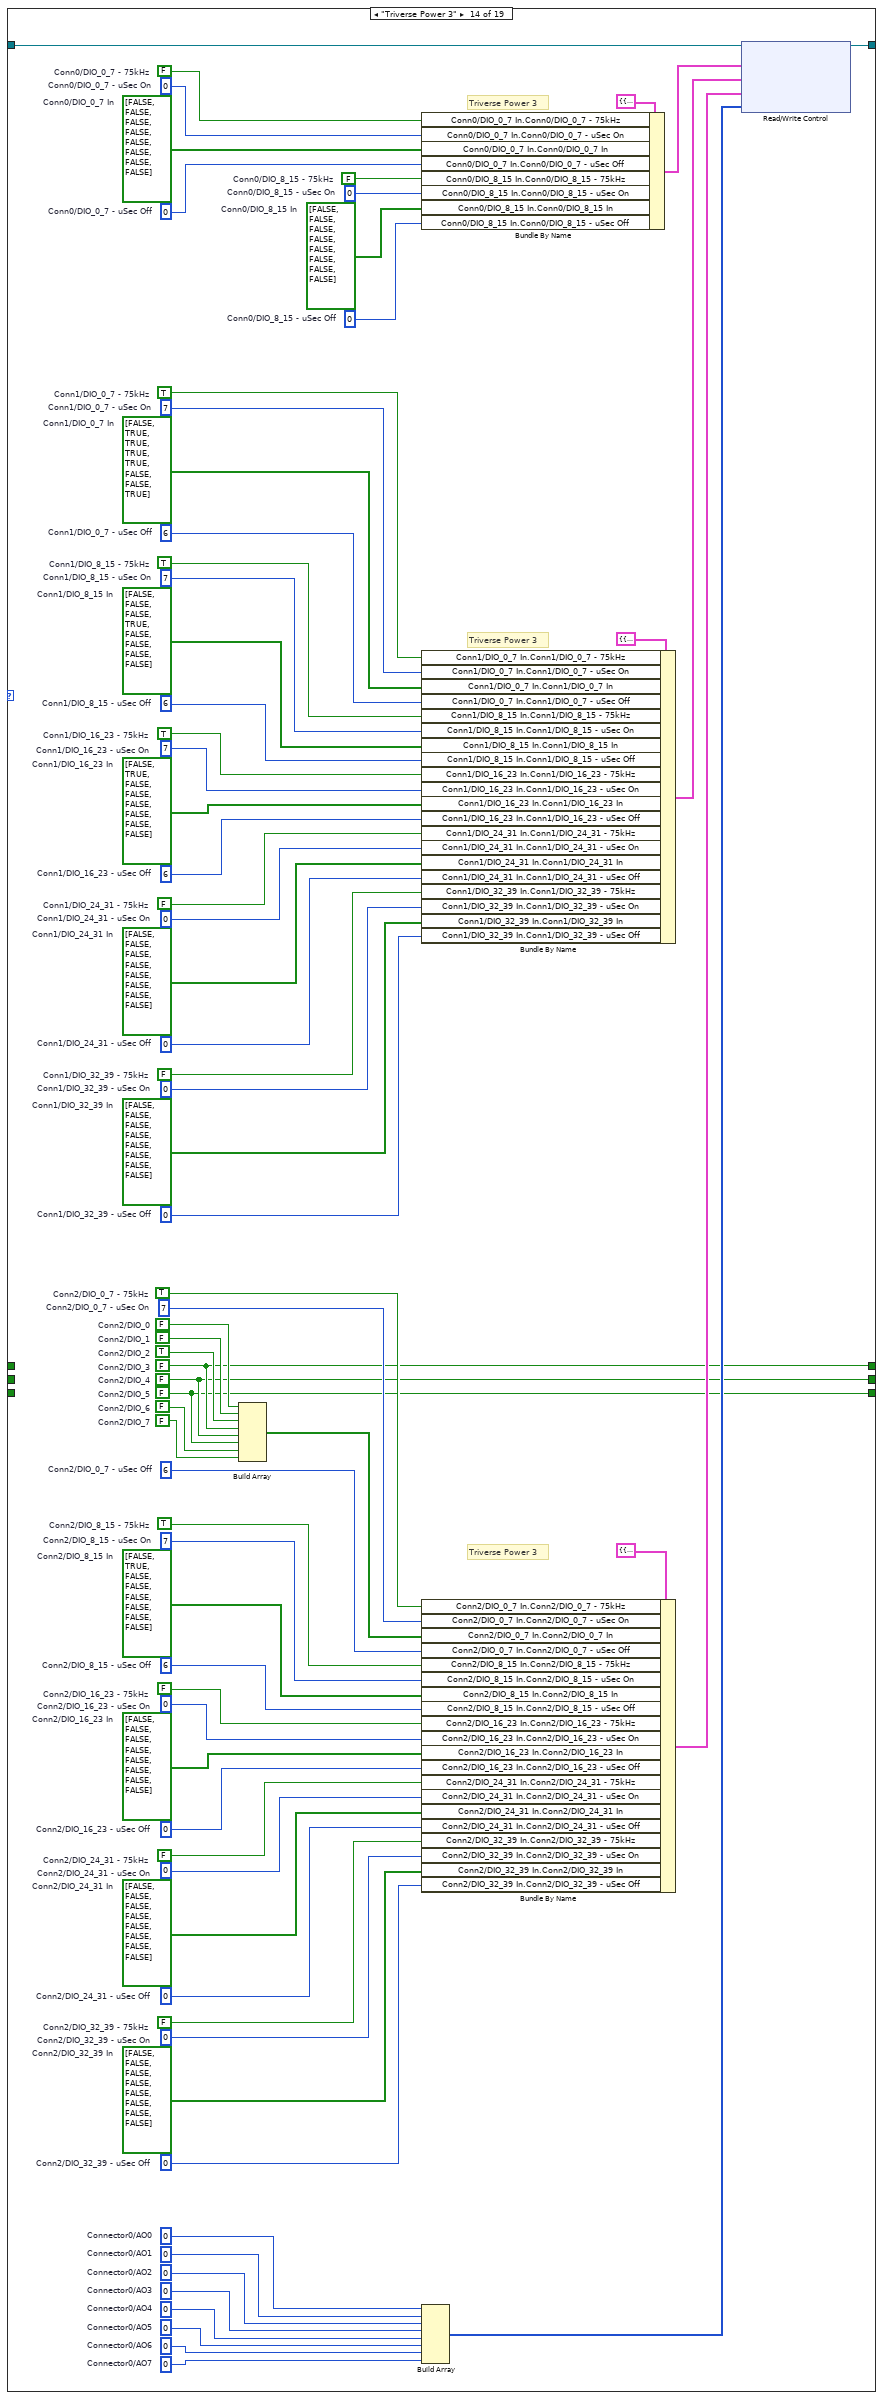
[diagram p14: hidden frame]
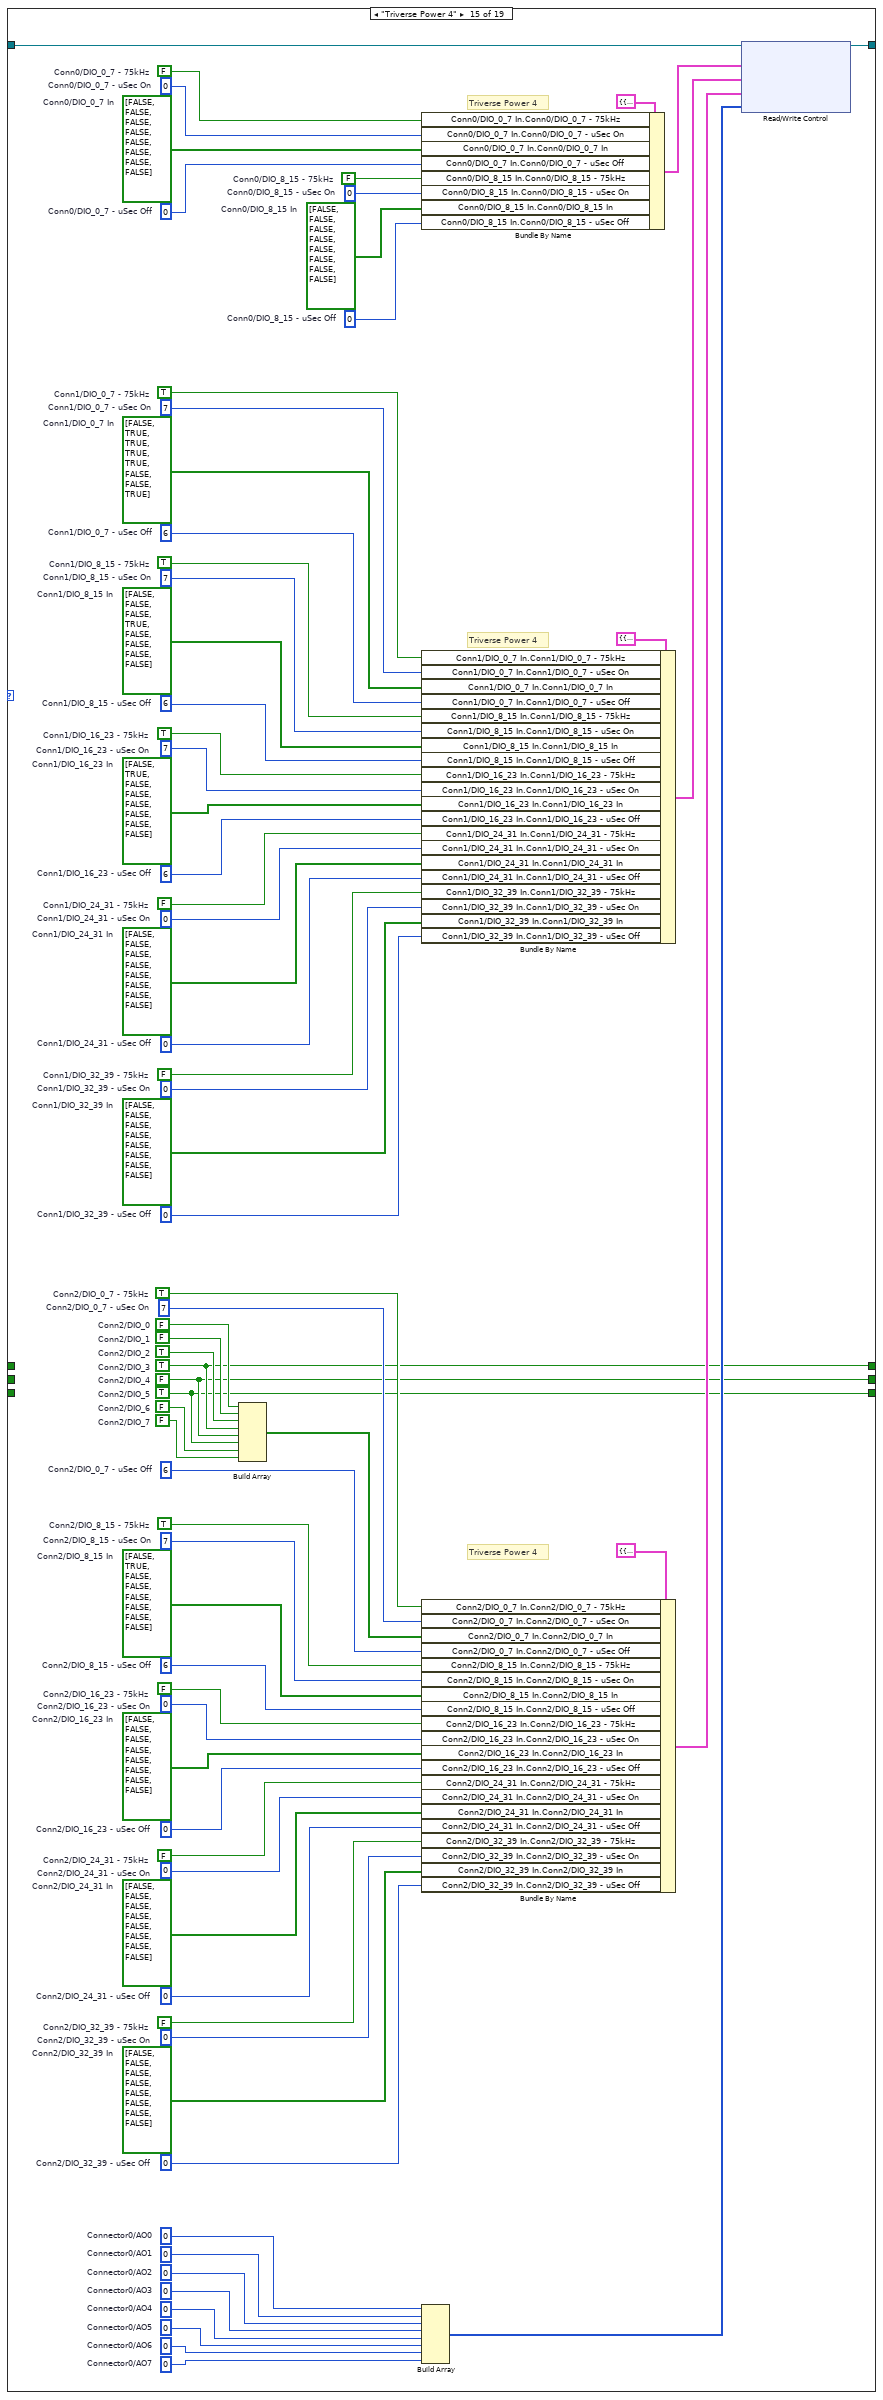
[diagram p15: hidden frame]
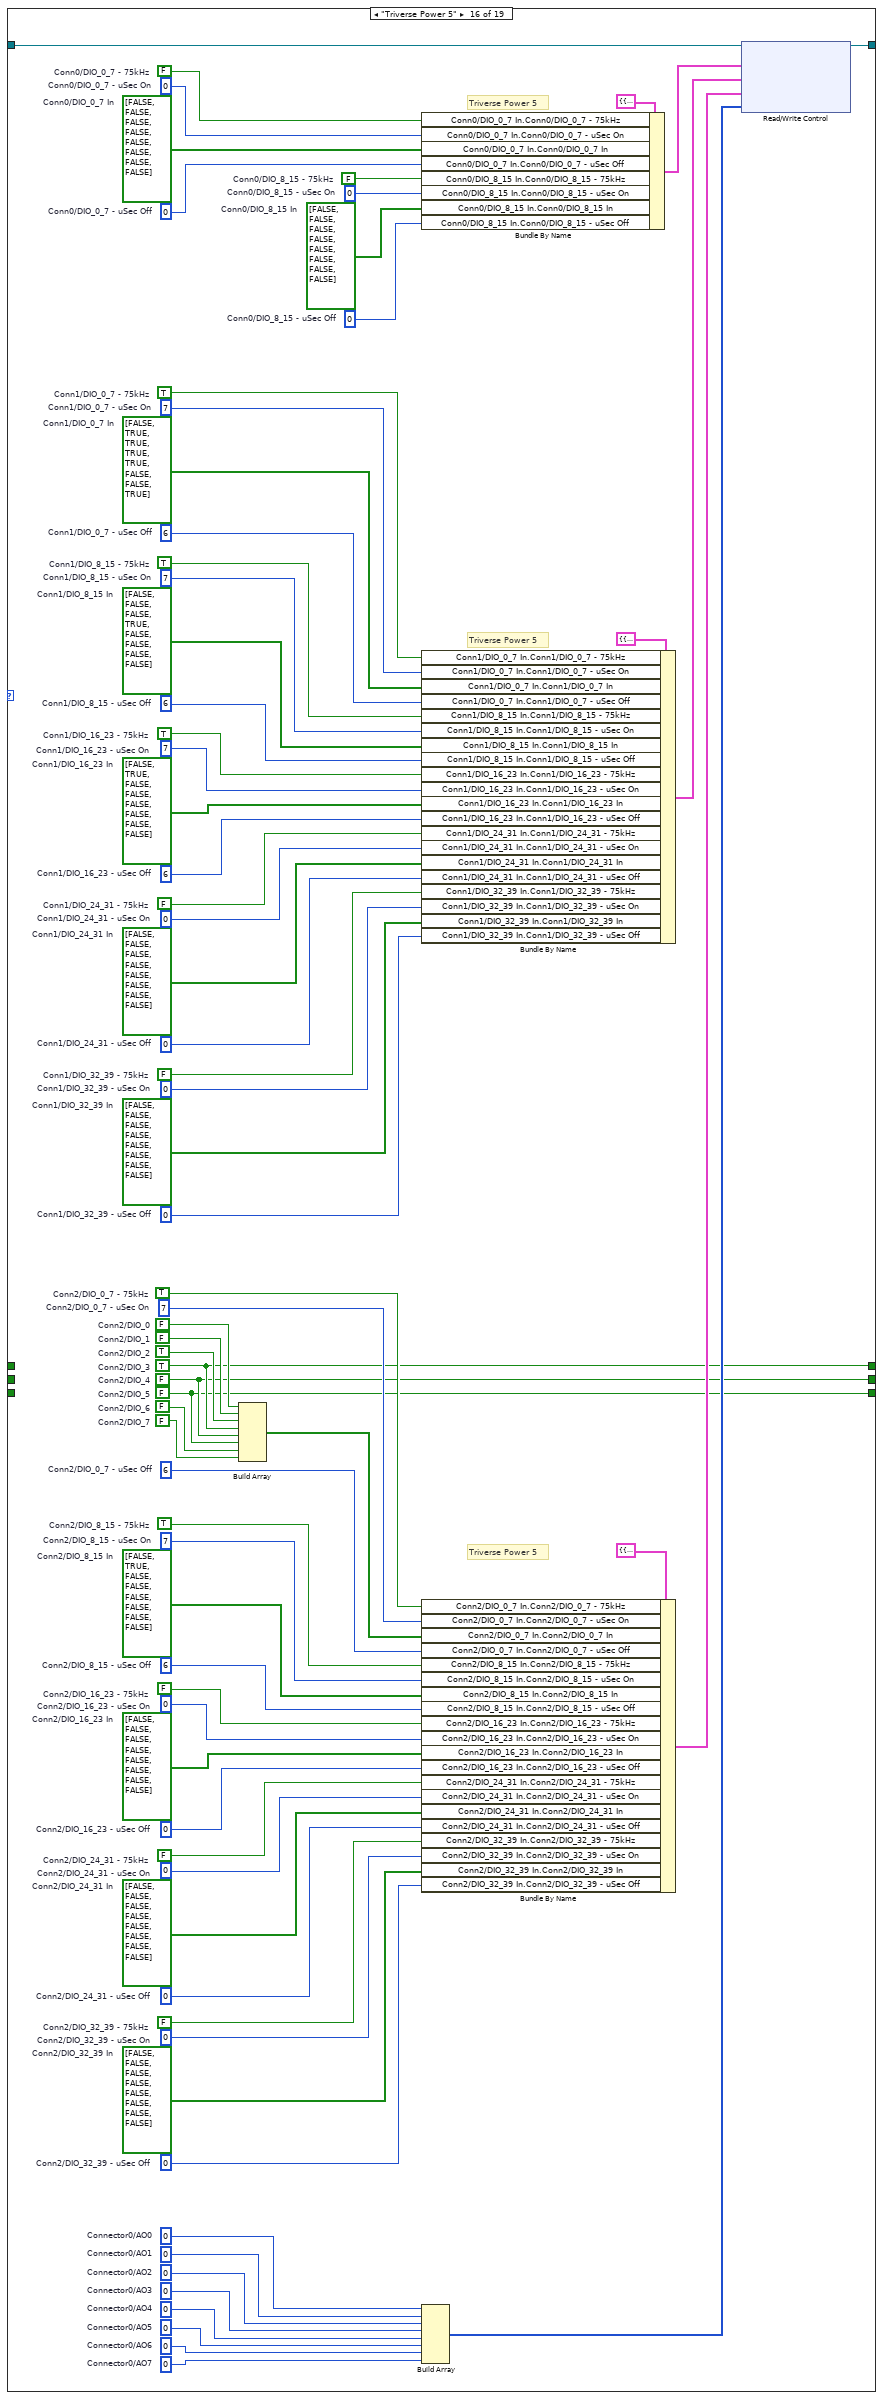
[diagram p16: hidden frame]
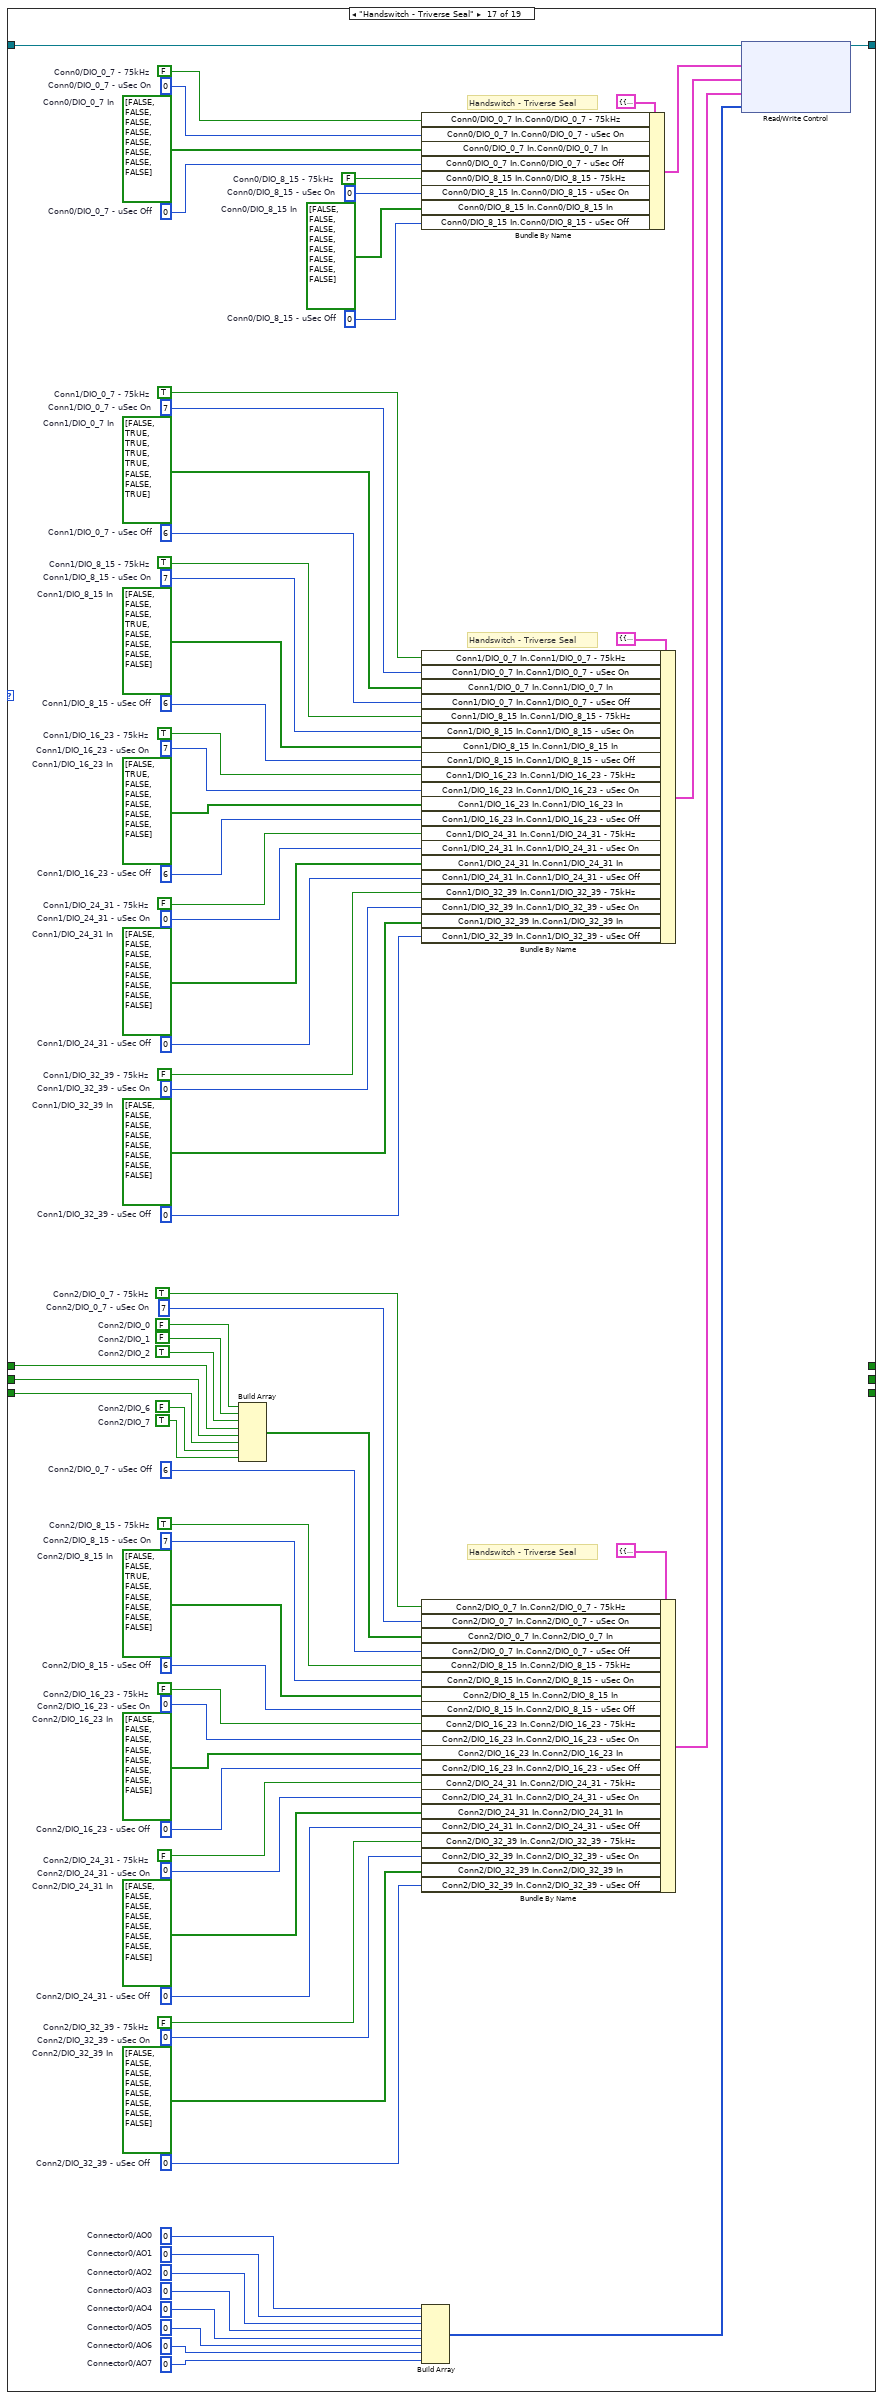
[diagram p17: hidden frame]
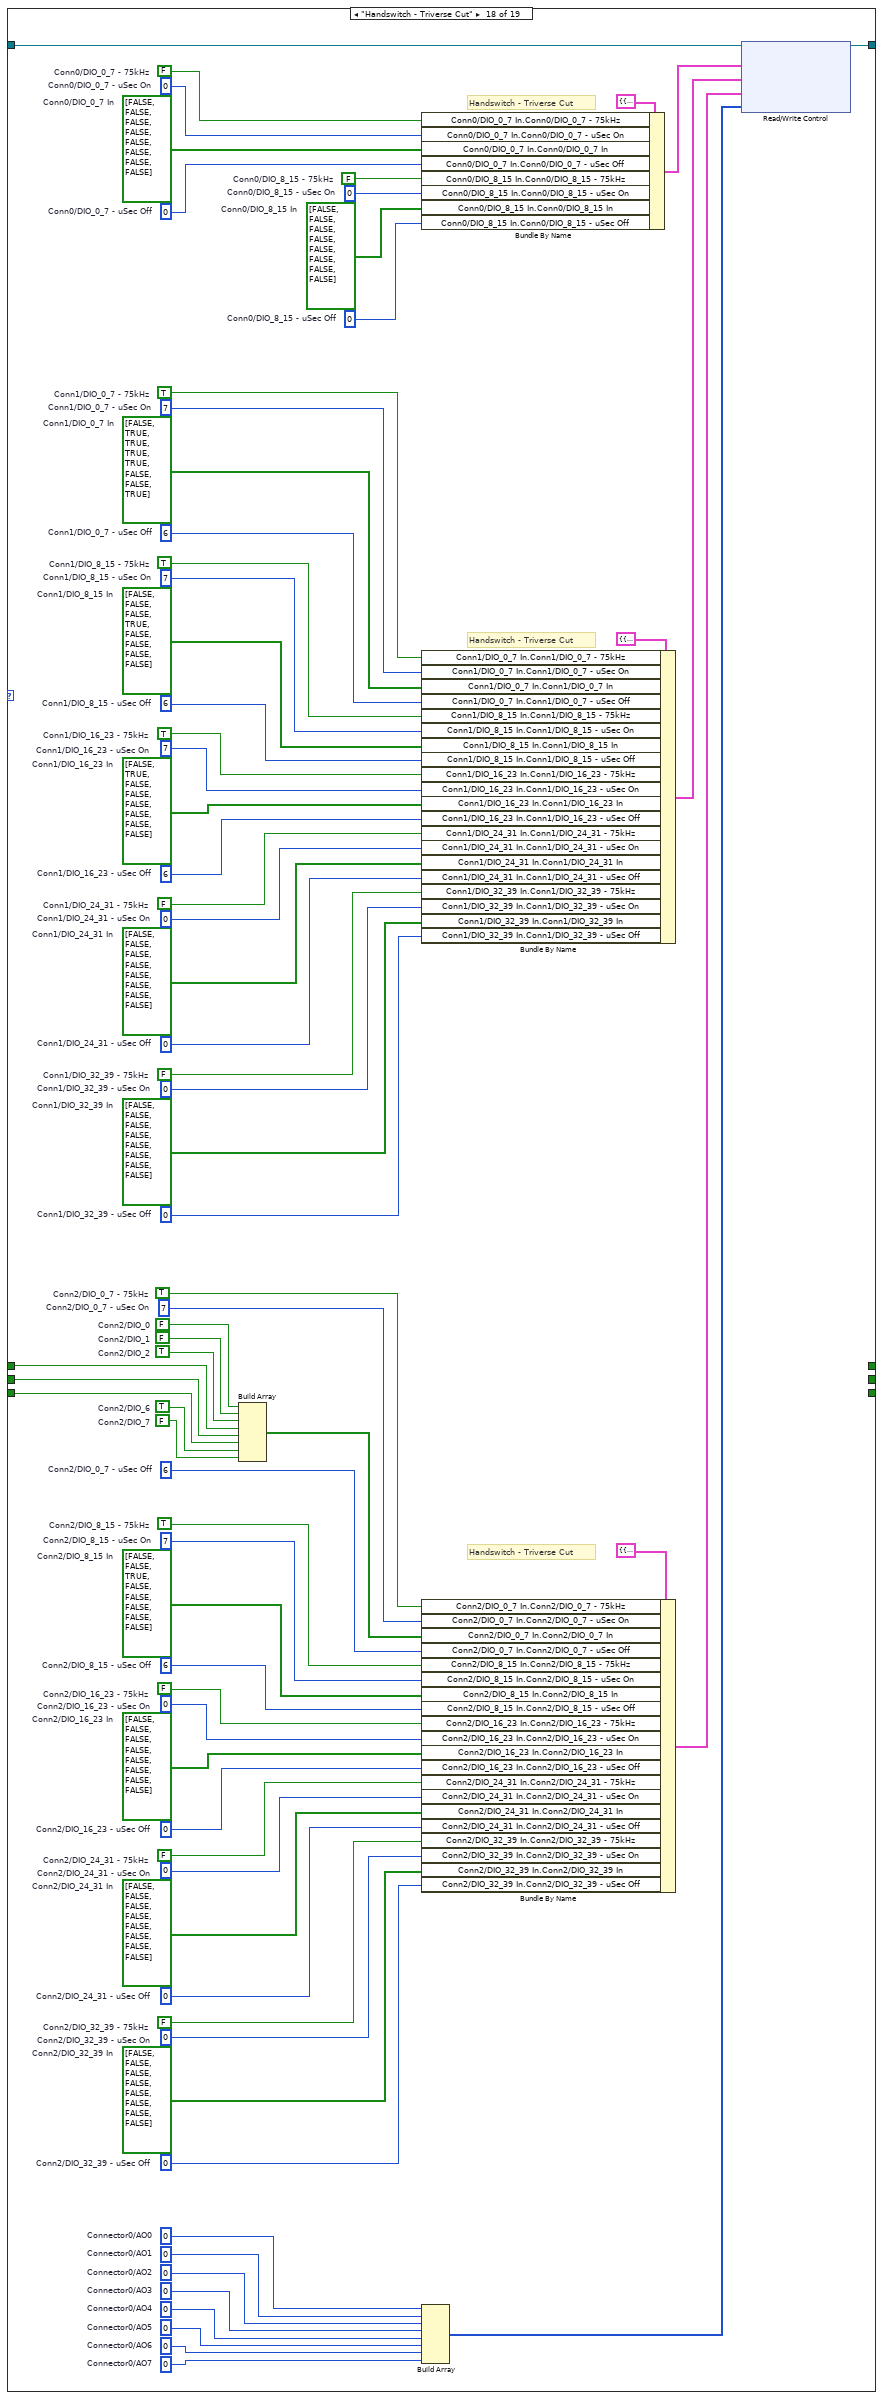
[diagram p18: hidden frame]
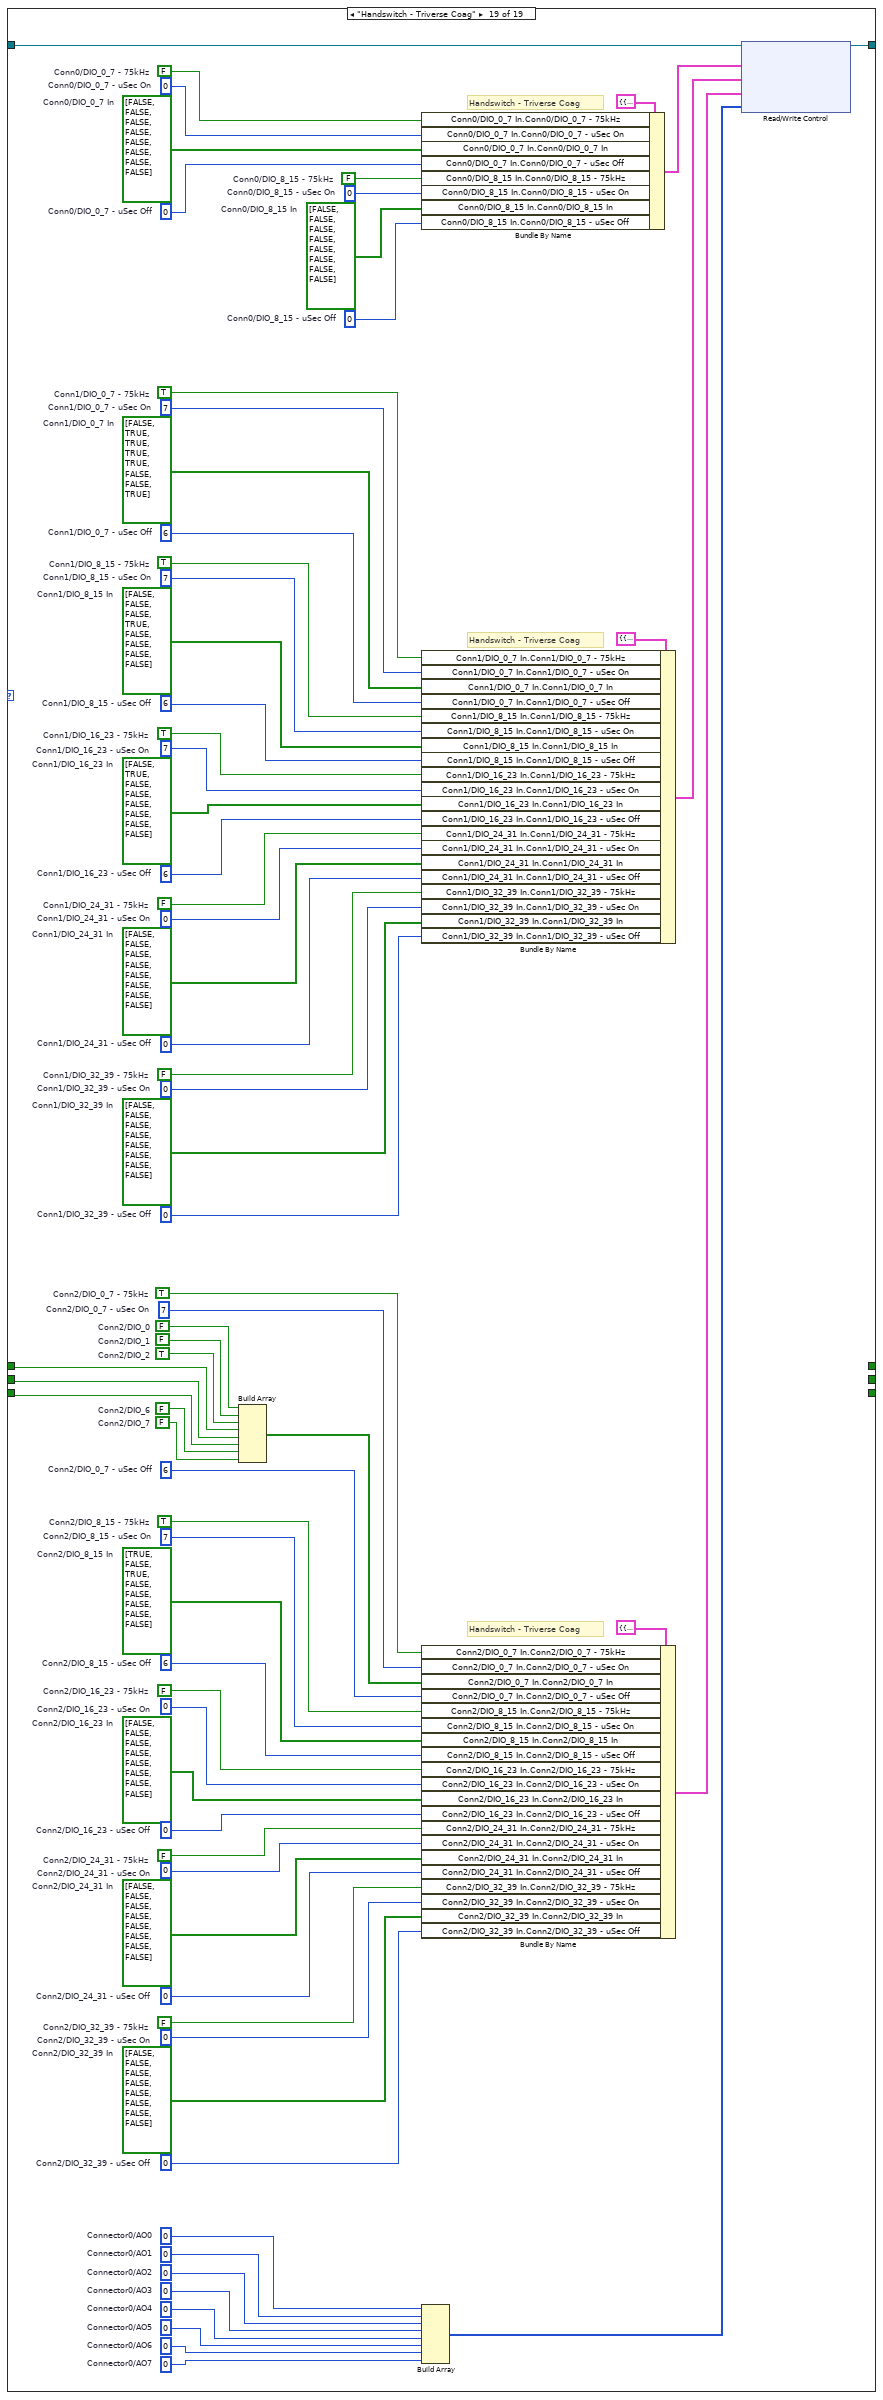
[diagram p19: hidden frame]
diagram:
  n1 = while {
    tunnel: "Update Config Enum" -> [w11]
    tunnel: "Refnum in" -> [w12]
    tunnel: [w13] -> w3
    shift-right: [w9] -> _
    shift-left: _ -> [w6]
    shift-right: [w8] -> _
    shift-left: _ -> [w5]
    shift-right: [w7] -> _
    shift-left: _ -> [w4]
    stop <- TRUE stop-if-true
    n2 = case shown="\"Off\"" w11 {
      tunnel: [w60 w126 w199 w263 w328 w393 w458 w523 w588 w656 w722 w796 w869 w942 w1015 w1088 w1161 w1234 w1307] -> w13
      tunnel: w12 -> [w59 w125 w198 w262 w327 w392 w457 w522 w587 w655 w721 w795 w868 w941 w1014 w1087 w1160 w1233 w1306]
      tunnel: [_ _ _ _ _ _ _ _ _ FALSE ("Conn2/DIO_3") _ w743 w816 w889 w962 w1035 _ _ _] -> w9
      tunnel: [_ _ _ _ _ _ _ _ _ FALSE ("Conn2/DIO_4") _ w742 w815 w888 w961 w1034 _ _ _] -> w8
      tunnel: [_ _ _ _ _ _ _ _ _ FALSE ("Conn2/DIO_5") _ w741 w814 w887 w960 w1033 _ _ _] -> w7
      tunnel: w6 -> [_ _ w146 _ _ _ _ _ _ _ _ _ _ _ _ _ w1108 w1181 w1254]
      tunnel: w5 -> [_ _ w145 _ _ _ _ _ _ _ _ _ _ _ _ _ w1107 w1180 w1253]
      tunnel: w4 -> [_ _ w144 _ _ _ _ _ _ _ _ _ _ _ _ _ w1106 w1179 w1252]
      frame "Off" {
        w15 = u16 0  # Conn2/DIO_32_39 - uSec Off
        w16 = bool[] [FALSE, FALSE, FALSE, FALSE, FALSE, FALSE, FALSE, FALSE]  # Conn2/DIO_32_39 In
        w17 = u16 0  # Conn2/DIO_32_39 - uSec On
        w18 = FALSE  # Conn2/DIO_32_39 - 75kHz
        w19 = u16 0  # Conn2/DIO_24_31 - uSec Off
        w20 = bool[] [FALSE, FALSE, FALSE, FALSE, FALSE, FALSE, FALSE, FALSE]  # Conn2/DIO_24_31 In
        w21 = u16 0  # Conn2/DIO_24_31 - uSec On
        w22 = FALSE  # Conn2/DIO_24_31 - 75kHz
        w23 = u16 0  # Conn2/DIO_16_23 - uSec Off
        w24 = bool[] [FALSE, FALSE, FALSE, FALSE, FALSE, FALSE, FALSE, FALSE]  # Conn2/DIO_16_23 In
        w25 = u16 0  # Conn2/DIO_16_23 - uSec On
        w26 = FALSE  # Conn2/DIO_16_23 - 75kHz
        w27 = u16 0  # Conn2/DIO_8_15 - uSec Off
        w28 = bool[] [FALSE, FALSE, FALSE, FALSE, FALSE, FALSE, FALSE, FALSE]  # Conn2/DIO_8_15 In
        w29 = u16 0  # Conn2/DIO_8_15 - uSec On
        w30 = FALSE  # Conn2/DIO_8_15 - 75kHz
        w31 = i16 0  # Connector0/AO7
        w32 = i16 0  # Connector0/AO6
        w33 = i16 0  # Connector0/AO5
        w34 = i16 0  # Connector0/AO4
        w35 = i16 0  # Connector0/AO3
        w36 = i16 0  # Connector0/AO2
        w37 = i16 0  # Connector0/AO1
        w38 = i16 0  # Connector0/AO0
        w39 = u16 0  # Conn1/DIO_32_39 - uSec Off
        w40 = bool[] [FALSE, FALSE, FALSE, FALSE, FALSE, FALSE, FALSE, FALSE]  # Conn1/DIO_32_39 In
        w41 = u16 0  # Conn1/DIO_32_39 - uSec On
        w42 = FALSE  # Conn1/DIO_32_39 - 75kHz
        w43 = u16 0  # Conn1/DIO_24_31 - uSec Off
        w44 = bool[] [FALSE, FALSE, FALSE, FALSE, FALSE, FALSE, FALSE, FALSE]  # Conn1/DIO_24_31 In
        w45 = u16 0  # Conn1/DIO_24_31 - uSec On
        w46 = FALSE  # Conn1/DIO_24_31 - 75kHz
        w47 = u16 0  # Conn1/DIO_16_23 - uSec Off
        w48 = bool[] [FALSE, FALSE, FALSE, FALSE, FALSE, FALSE, FALSE, FALSE]  # Conn1/DIO_16_23 In
        w49 = u16 0  # Conn1/DIO_16_23 - uSec On
        w50 = FALSE  # Conn1/DIO_16_23 - 75kHz
        w51 = u16 0  # Conn1/DIO_8_15 - uSec Off
        w52 = bool[] [FALSE, FALSE, FALSE, FALSE, FALSE, FALSE, FALSE, FALSE]  # Conn1/DIO_8_15 In
        w53 = u16 0  # Conn1/DIO_8_15 - uSec On
        w54 = FALSE  # Conn1/DIO_8_15 - 75kHz
        w55 = u16 0  # Conn0/DIO_8_15 - uSec Off
        w56 = bool[] [FALSE, FALSE, FALSE, FALSE, FALSE, FALSE, FALSE, FALSE]  # Conn0/DIO_8_15 In
        w57 = u16 0  # Conn0/DIO_8_15 - uSec On
        w58 = FALSE  # Conn0/DIO_8_15 - 75kHz
        w75 = u16 0  # Conn0/DIO_0_7 - uSec Off
        w74 = bool[] [FALSE, FALSE, FALSE, FALSE, FALSE, FALSE, FALSE, FALSE]  # Conn0/DIO_0_7 In
        w73 = u16 0  # Conn0/DIO_0_7 - uSec On
        w72 = FALSE  # Conn0/DIO_0_7 - 75kHz
        w71 = u16 0  # Conn1/DIO_0_7 - uSec Off
        w70 = bool[] [FALSE, FALSE, FALSE, FALSE, FALSE, FALSE, FALSE, FALSE]  # Conn1/DIO_0_7 In
        w69 = u16 0  # Conn1/DIO_0_7 - uSec On
        w68 = FALSE  # Conn1/DIO_0_7 - 75kHz
        w67 = u16 0  # Conn2/DIO_0_7 - uSec Off
        w66 = bool[] [FALSE, FALSE, FALSE, FALSE, FALSE, FALSE, FALSE, FALSE]  # Conn2/DIO_0_7 In
        w65 = u16 0  # Conn2/DIO_0_7 - uSec On
        w64 = FALSE  # Conn2/DIO_0_7 - 75kHz
        # "Off"
        # "Off"
        # "Off"
        n3 = Bundle By Name(cluster=T4 {"Conn0/DIO_0_7 In"={"Conn0/DIO_0_7 - 75kHz"=FALSE, "Conn0/DIO_0_7 - uSec On"=0, "Conn0/DIO_0_7 In"=[FALSE, FALSE, FALSE, FALSE, FALSE, FALSE, FALSE, FALSE], "Conn0/DIO_0_7 - uSec Off"=0}, "Conn0/DIO_8_15 In"={"Conn0/DIO_8_15 - 75kHz"=FALSE, "Conn0/DIO_8_15 - uSec On"=0, "Conn0/DIO_8_15 In"=[FALSE, FALSE, FALSE, FALSE, FALSE, FALSE, FALSE, FALSE], "Conn0/DIO_8_15 - uSec Off"=0}} ("Conn0 DIOs In"), "Conn0/DIO_0_7 In.Conn0/DIO_0_7 - 75kHz"=w72, "Conn0/DIO_0_7 In.Conn0/DIO_0_7 - uSec On"=w73, "Conn0/DIO_0_7 In.Conn0/DIO_0_7 In"=w74, "Conn0/DIO_0_7 In.Conn0/DIO_0_7 - uSec Off"=w75, "Conn0/DIO_8_15 In.Conn0/DIO_8_15 - 75kHz"=w58, "Conn0/DIO_8_15 In.Conn0/DIO_8_15 - uSec On"=w57, "Conn0/DIO_8_15 In.Conn0/DIO_8_15 In"=w56, "Conn0/DIO_8_15 In.Conn0/DIO_8_15 - uSec Off"=w55) -> (w62:T4)
        n4 = Bundle By Name(cluster=T3 {"Conn1/DIO_0_7 In"={"Conn1/DIO_0_7 - 75kHz"=FALSE, "Conn1/DIO_0_7 - uSec On"=0, "Conn1/DIO_0_7 In"=[FALSE, FALSE, FALSE, FALSE, FALSE, FALSE, FALSE, FALSE], "Conn1/DIO_0_7 - uSec Off"=0}, "Conn1/DIO_8_15 In"={"Conn1/DIO_8_15 - 75kHz"=FALSE, "Conn1/DIO_8_15 - uSec On"=0, "Conn1/DIO_8_15 In"=[FALSE, FALSE, FALSE, FALSE, FALSE, FALSE, FALSE, FALSE], "Conn1/DIO_8_15 - uSec Off"=0}, "Conn1/DIO_16_23 In"={"Conn1/DIO_16_23 - 75kHz"=FALSE, "Conn1/DIO_16_23 - uSec On"=0, "Conn1/DIO_16_23 In"=[FALSE, FALSE, FALSE, FALSE, FALSE, FALSE, FALSE, FALSE], "Conn1/DIO_16_23 - uSec Off"=0}, "Conn1/DIO_24_31 In"={"Conn1/DIO_24_31 - 75kHz"=FALSE, "Conn1/DIO_24_31 - uSec On"=0, "Conn1/DIO_24_31 In"=[FALSE, FALSE, FALSE, FALSE, FALSE, FALSE, FALSE, FALSE], "Conn1/DIO_24_31 - uSec Off"=0}, "Conn1/DIO_32_39 In"={"Conn1/DIO_32_39 - 75kHz"=FALSE, "Conn1/DIO_32_39 - uSec On"=0, "Conn1/DIO_32_39 In"=[FALSE, FALSE, FALSE, FALSE, FALSE, FALSE, FALSE, FALSE], "Conn1/DIO_32_39 - uSec Off"=0}} ("Conn1 DIOs In"), "Conn1/DIO_0_7 In.Conn1/DIO_0_7 - 75kHz"=w68, "Conn1/DIO_0_7 In.Conn1/DIO_0_7 - uSec On"=w69, "Conn1/DIO_0_7 In.Conn1/DIO_0_7 In"=w70, "Conn1/DIO_0_7 In.Conn1/DIO_0_7 - uSec Off"=w71, "Conn1/DIO_8_15 In.Conn1/DIO_8_15 - 75kHz"=w54, "Conn1/DIO_8_15 In.Conn1/DIO_8_15 - uSec On"=w53, "Conn1/DIO_8_15 In.Conn1/DIO_8_15 In"=w52, "Conn1/DIO_8_15 In.Conn1/DIO_8_15 - uSec Off"=w51, "Conn1/DIO_16_23 In.Conn1/DIO_16_23 - 75kHz"=w50, "Conn1/DIO_16_23 In.Conn1/DIO_16_23 - uSec On"=w49, "Conn1/DIO_16_23 In.Conn1/DIO_16_23 In"=w48, "Conn1/DIO_16_23 In.Conn1/DIO_16_23 - uSec Off"=w47, "Conn1/DIO_24_31 In.Conn1/DIO_24_31 - 75kHz"=w46, "Conn1/DIO_24_31 In.Conn1/DIO_24_31 - uSec On"=w45, "Conn1/DIO_24_31 In.Conn1/DIO_24_31 In"=w44, "Conn1/DIO_24_31 In.Conn1/DIO_24_31 - uSec Off"=w43, "Conn1/DIO_32_39 In.Conn1/DIO_32_39 - 75kHz"=w42, "Conn1/DIO_32_39 In.Conn1/DIO_32_39 - uSec On"=w41, "Conn1/DIO_32_39 In.Conn1/DIO_32_39 In"=w40, "Conn1/DIO_32_39 In.Conn1/DIO_32_39 - uSec Off"=w39) -> (w76:T3)
        n5 = Bundle By Name(cluster=T2 {"Conn2/DIO_0_7 In"={"Conn2/DIO_0_7 - 75kHz"=FALSE, "Conn2/DIO_0_7 - uSec On"=0, "Conn2/DIO_0_7 In"=[FALSE, FALSE, FALSE, FALSE, FALSE, FALSE, FALSE, FALSE], "Conn2/DIO_0_7 - uSec Off"=0}, "Conn2/DIO_8_15 In"={"Conn2/DIO_8_15 - 75kHz"=FALSE, "Conn2/DIO_8_15 - uSec On"=0, "Conn2/DIO_8_15 In"=[FALSE, FALSE, FALSE, FALSE, FALSE, FALSE, FALSE, FALSE], "Conn2/DIO_8_15 - uSec Off"=0}, "Conn2/DIO_16_23 In"={"Conn2/DIO_16_23 - 75kHz"=FALSE, "Conn2/DIO_16_23 - uSec On"=0, "Conn2/DIO_16_23 In"=[FALSE, FALSE, FALSE, FALSE, FALSE, FALSE, FALSE, FALSE], "Conn2/DIO_16_23 - uSec Off"=0}, "Conn2/DIO_24_31 In"={"Conn2/DIO_24_31 - 75kHz"=FALSE, "Conn2/DIO_24_31 - uSec On"=0, "Conn2/DIO_24_31 In"=[FALSE, FALSE, FALSE, FALSE, FALSE, FALSE, FALSE, FALSE], "Conn2/DIO_24_31 - uSec Off"=0}, "Conn2/DIO_32_39 In"={"Conn2/DIO_32_39 - 75kHz"=FALSE, "Conn2/DIO_32_39 - uSec On"=0, "Conn2/DIO_32_39 In"=[FALSE, FALSE, FALSE, FALSE, FALSE, FALSE, FALSE, FALSE], "Conn2/DIO_32_39 - uSec Off"=0}} ("Conn2 DIOs In"), "Conn2/DIO_0_7 In.Conn2/DIO_0_7 - 75kHz"=w64, "Conn2/DIO_0_7 In.Conn2/DIO_0_7 - uSec On"=w65, "Conn2/DIO_0_7 In.Conn2/DIO_0_7 In"=w66, "Conn2/DIO_0_7 In.Conn2/DIO_0_7 - uSec Off"=w67, "Conn2/DIO_8_15 In.Conn2/DIO_8_15 - 75kHz"=w30, "Conn2/DIO_8_15 In.Conn2/DIO_8_15 - uSec On"=w29, "Conn2/DIO_8_15 In.Conn2/DIO_8_15 In"=w28, "Conn2/DIO_8_15 In.Conn2/DIO_8_15 - uSec Off"=w27, "Conn2/DIO_16_23 In.Conn2/DIO_16_23 - 75kHz"=w26, "Conn2/DIO_16_23 In.Conn2/DIO_16_23 - uSec On"=w25, "Conn2/DIO_16_23 In.Conn2/DIO_16_23 In"=w24, "Conn2/DIO_16_23 In.Conn2/DIO_16_23 - uSec Off"=w23, "Conn2/DIO_24_31 In.Conn2/DIO_24_31 - 75kHz"=w22, "Conn2/DIO_24_31 In.Conn2/DIO_24_31 - uSec On"=w21, "Conn2/DIO_24_31 In.Conn2/DIO_24_31 In"=w20, "Conn2/DIO_24_31 In.Conn2/DIO_24_31 - uSec Off"=w19, "Conn2/DIO_32_39 In.Conn2/DIO_32_39 - 75kHz"=w18, "Conn2/DIO_32_39 In.Conn2/DIO_32_39 - uSec On"=w17, "Conn2/DIO_32_39 In.Conn2/DIO_32_39 In"=w16, "Conn2/DIO_32_39 In.Conn2/DIO_32_39 - uSec Off"=w15) -> (w77:T2)
        n6 = Build Array(w38, w37, w36, w35, w34, w33, w32, w31) -> (w78:i16[])
        n7 = xnode "Read/Write Control"("FPGA VI Reference In"=w59, "Conn0 DIOs In"=w62, "Conn1 DIOs In"=w76, "Conn2 DIOs In"=w77, "Connector0/AO0_7"=w78) -> ("FPGA VI Reference Out"=w60:refnum<k20>)  [unwired: 1 in, 1 out]
      }
      frame "Mono1 Relay Config" {
        w81 = u16 0  # Conn2/DIO_32_39 - uSec Off
        w82 = bool[] [FALSE, FALSE, FALSE, FALSE, FALSE, FALSE, FALSE, FALSE]  # Conn2/DIO_32_39 In
        w83 = u16 0  # Conn2/DIO_32_39 - uSec On
        w84 = FALSE  # Conn2/DIO_32_39 - 75kHz
        w85 = u16 0  # Conn2/DIO_24_31 - uSec Off
        w86 = bool[] [FALSE, FALSE, FALSE, FALSE, FALSE, FALSE, FALSE, FALSE]  # Conn2/DIO_24_31 In
        w87 = u16 0  # Conn2/DIO_24_31 - uSec On
        w88 = FALSE  # Conn2/DIO_24_31 - 75kHz
        w89 = u16 0  # Conn2/DIO_16_23 - uSec Off
        w90 = bool[] [FALSE, FALSE, FALSE, FALSE, FALSE, FALSE, FALSE, FALSE]  # Conn2/DIO_16_23 In
        w91 = u16 0  # Conn2/DIO_16_23 - uSec On
        w92 = FALSE  # Conn2/DIO_16_23 - 75kHz
        w93 = u16 0  # Conn2/DIO_8_15 - uSec Off
        w94 = bool[] [FALSE, FALSE, FALSE, FALSE, FALSE, FALSE, FALSE, FALSE]  # Conn2/DIO_8_15 In
        w95 = u16 0  # Conn2/DIO_8_15 - uSec On
        w96 = FALSE  # Conn2/DIO_8_15 - 75kHz
        w97 = i16 0  # Connector0/AO7
        w98 = i16 0  # Connector0/AO6
        w99 = i16 0  # Connector0/AO5
        w100 = i16 0  # Connector0/AO4
        w101 = i16 0  # Connector0/AO3
        w102 = i16 0  # Connector0/AO2
        w103 = i16 0  # Connector0/AO1
        w104 = i16 0  # Connector0/AO0
        w105 = u16 0  # Conn1/DIO_32_39 - uSec Off
        w106 = bool[] [FALSE, FALSE, FALSE, FALSE, FALSE, FALSE, FALSE, FALSE]  # Conn1/DIO_32_39 In
        w107 = u16 0  # Conn1/DIO_32_39 - uSec On
        w108 = FALSE  # Conn1/DIO_32_39 - 75kHz
        w109 = u16 0  # Conn1/DIO_24_31 - uSec Off
        w110 = bool[] [FALSE, FALSE, FALSE, FALSE, FALSE, FALSE, FALSE, FALSE]  # Conn1/DIO_24_31 In
        w111 = u16 0  # Conn1/DIO_24_31 - uSec On
        w112 = FALSE  # Conn1/DIO_24_31 - 75kHz
        w113 = u16 6  # Conn1/DIO_16_23 - uSec Off
        w114 = bool[] [FALSE, TRUE, FALSE, FALSE, FALSE, FALSE, FALSE, FALSE]  # Conn1/DIO_16_23 In
        w115 = u16 7  # Conn1/DIO_16_23 - uSec On
        w116 = TRUE  # Conn1/DIO_16_23 - 75kHz
        w117 = u16 6  # Conn1/DIO_8_15 - uSec Off
        w118 = bool[] [FALSE, FALSE, FALSE, TRUE, FALSE, FALSE, FALSE, FALSE]  # Conn1/DIO_8_15 In
        w119 = u16 7  # Conn1/DIO_8_15 - uSec On
        w120 = TRUE  # Conn1/DIO_8_15 - 75kHz
        w121 = u16 0  # Conn0/DIO_8_15 - uSec Off
        w122 = bool[] [FALSE, FALSE, FALSE, FALSE, FALSE, FALSE, FALSE, FALSE]  # Conn0/DIO_8_15 In
        w123 = u16 0  # Conn0/DIO_8_15 - uSec On
        w124 = FALSE  # Conn0/DIO_8_15 - 75kHz
        w141 = u16 0  # Conn0/DIO_0_7 - uSec Off
        w140 = bool[] [FALSE, FALSE, FALSE, FALSE, FALSE, FALSE, FALSE, FALSE]  # Conn0/DIO_0_7 In
        w139 = u16 0  # Conn0/DIO_0_7 - uSec On
        w138 = FALSE  # Conn0/DIO_0_7 - 75kHz
        w137 = u16 6  # Conn1/DIO_0_7 - uSec Off
        w136 = bool[] [TRUE, TRUE, TRUE, TRUE, TRUE, FALSE, FALSE, FALSE]  # Conn1/DIO_0_7 In
        w135 = u16 7  # Conn1/DIO_0_7 - uSec On
        w134 = TRUE  # Conn1/DIO_0_7 - 75kHz
        w133 = u16 0  # Conn2/DIO_0_7 - uSec Off
        w132 = bool[] [FALSE, FALSE, FALSE, FALSE, FALSE, FALSE, FALSE, FALSE]  # Conn2/DIO_0_7 In
        w131 = u16 0  # Conn2/DIO_0_7 - uSec On
        w130 = FALSE  # Conn2/DIO_0_7 - 75kHz
        # "Mono1 Relay Config"
        # "Mono1 Relay Config"
        # "Mono1 Relay Config"
        n8 = Bundle By Name(cluster=T4 {"Conn0/DIO_0_7 In"={"Conn0/DIO_0_7 - 75kHz"=FALSE, "Conn0/DIO_0_7 - uSec On"=0, "Conn0/DIO_0_7 In"=[FALSE, FALSE, FALSE, FALSE, FALSE, FALSE, FALSE, FALSE], "Conn0/DIO_0_7 - uSec Off"=0}, "Conn0/DIO_8_15 In"={"Conn0/DIO_8_15 - 75kHz"=FALSE, "Conn0/DIO_8_15 - uSec On"=0, "Conn0/DIO_8_15 In"=[FALSE, FALSE, FALSE, FALSE, FALSE, FALSE, FALSE, FALSE], "Conn0/DIO_8_15 - uSec Off"=0}} ("Conn0 DIOs In"), "Conn0/DIO_0_7 In.Conn0/DIO_0_7 - 75kHz"=w138, "Conn0/DIO_0_7 In.Conn0/DIO_0_7 - uSec On"=w139, "Conn0/DIO_0_7 In.Conn0/DIO_0_7 In"=w140, "Conn0/DIO_0_7 In.Conn0/DIO_0_7 - uSec Off"=w141, "Conn0/DIO_8_15 In.Conn0/DIO_8_15 - 75kHz"=w124, "Conn0/DIO_8_15 In.Conn0/DIO_8_15 - uSec On"=w123, "Conn0/DIO_8_15 In.Conn0/DIO_8_15 In"=w122, "Conn0/DIO_8_15 In.Conn0/DIO_8_15 - uSec Off"=w121) -> (w128:T4)
        n9 = Bundle By Name(cluster=T3 {"Conn1/DIO_0_7 In"={"Conn1/DIO_0_7 - 75kHz"=FALSE, "Conn1/DIO_0_7 - uSec On"=0, "Conn1/DIO_0_7 In"=[FALSE, FALSE, FALSE, FALSE, FALSE, FALSE, FALSE, FALSE], "Conn1/DIO_0_7 - uSec Off"=0}, "Conn1/DIO_8_15 In"={"Conn1/DIO_8_15 - 75kHz"=FALSE, "Conn1/DIO_8_15 - uSec On"=0, "Conn1/DIO_8_15 In"=[FALSE, FALSE, FALSE, FALSE, FALSE, FALSE, FALSE, FALSE], "Conn1/DIO_8_15 - uSec Off"=0}, "Conn1/DIO_16_23 In"={"Conn1/DIO_16_23 - 75kHz"=FALSE, "Conn1/DIO_16_23 - uSec On"=0, "Conn1/DIO_16_23 In"=[FALSE, FALSE, FALSE, FALSE, FALSE, FALSE, FALSE, FALSE], "Conn1/DIO_16_23 - uSec Off"=0}, "Conn1/DIO_24_31 In"={"Conn1/DIO_24_31 - 75kHz"=FALSE, "Conn1/DIO_24_31 - uSec On"=0, "Conn1/DIO_24_31 In"=[FALSE, FALSE, FALSE, FALSE, FALSE, FALSE, FALSE, FALSE], "Conn1/DIO_24_31 - uSec Off"=0}, "Conn1/DIO_32_39 In"={"Conn1/DIO_32_39 - 75kHz"=FALSE, "Conn1/DIO_32_39 - uSec On"=0, "Conn1/DIO_32_39 In"=[FALSE, FALSE, FALSE, FALSE, FALSE, FALSE, FALSE, FALSE], "Conn1/DIO_32_39 - uSec Off"=0}} ("Conn1 DIOs In"), "Conn1/DIO_0_7 In.Conn1/DIO_0_7 - 75kHz"=w134, "Conn1/DIO_0_7 In.Conn1/DIO_0_7 - uSec On"=w135, "Conn1/DIO_0_7 In.Conn1/DIO_0_7 In"=w136, "Conn1/DIO_0_7 In.Conn1/DIO_0_7 - uSec Off"=w137, "Conn1/DIO_8_15 In.Conn1/DIO_8_15 - 75kHz"=w120, "Conn1/DIO_8_15 In.Conn1/DIO_8_15 - uSec On"=w119, "Conn1/DIO_8_15 In.Conn1/DIO_8_15 In"=w118, "Conn1/DIO_8_15 In.Conn1/DIO_8_15 - uSec Off"=w117, "Conn1/DIO_16_23 In.Conn1/DIO_16_23 - 75kHz"=w116, "Conn1/DIO_16_23 In.Conn1/DIO_16_23 - uSec On"=w115, "Conn1/DIO_16_23 In.Conn1/DIO_16_23 In"=w114, "Conn1/DIO_16_23 In.Conn1/DIO_16_23 - uSec Off"=w113, "Conn1/DIO_24_31 In.Conn1/DIO_24_31 - 75kHz"=w112, "Conn1/DIO_24_31 In.Conn1/DIO_24_31 - uSec On"=w111, "Conn1/DIO_24_31 In.Conn1/DIO_24_31 In"=w110, "Conn1/DIO_24_31 In.Conn1/DIO_24_31 - uSec Off"=w109, "Conn1/DIO_32_39 In.Conn1/DIO_32_39 - 75kHz"=w108, "Conn1/DIO_32_39 In.Conn1/DIO_32_39 - uSec On"=w107, "Conn1/DIO_32_39 In.Conn1/DIO_32_39 In"=w106, "Conn1/DIO_32_39 In.Conn1/DIO_32_39 - uSec Off"=w105) -> (w142:T3)
        n10 = Bundle By Name(cluster=T2 {"Conn2/DIO_0_7 In"={"Conn2/DIO_0_7 - 75kHz"=FALSE, "Conn2/DIO_0_7 - uSec On"=0, "Conn2/DIO_0_7 In"=[FALSE, FALSE, FALSE, FALSE, FALSE, FALSE, FALSE, FALSE], "Conn2/DIO_0_7 - uSec Off"=0}, "Conn2/DIO_8_15 In"={"Conn2/DIO_8_15 - 75kHz"=FALSE, "Conn2/DIO_8_15 - uSec On"=0, "Conn2/DIO_8_15 In"=[FALSE, FALSE, FALSE, FALSE, FALSE, FALSE, FALSE, FALSE], "Conn2/DIO_8_15 - uSec Off"=0}, "Conn2/DIO_16_23 In"={"Conn2/DIO_16_23 - 75kHz"=FALSE, "Conn2/DIO_16_23 - uSec On"=0, "Conn2/DIO_16_23 In"=[FALSE, FALSE, FALSE, FALSE, FALSE, FALSE, FALSE, FALSE], "Conn2/DIO_16_23 - uSec Off"=0}, "Conn2/DIO_24_31 In"={"Conn2/DIO_24_31 - 75kHz"=FALSE, "Conn2/DIO_24_31 - uSec On"=0, "Conn2/DIO_24_31 In"=[FALSE, FALSE, FALSE, FALSE, FALSE, FALSE, FALSE, FALSE], "Conn2/DIO_24_31 - uSec Off"=0}, "Conn2/DIO_32_39 In"={"Conn2/DIO_32_39 - 75kHz"=FALSE, "Conn2/DIO_32_39 - uSec On"=0, "Conn2/DIO_32_39 In"=[FALSE, FALSE, FALSE, FALSE, FALSE, FALSE, FALSE, FALSE], "Conn2/DIO_32_39 - uSec Off"=0}} ("Conn2 DIOs In"), "Conn2/DIO_0_7 In.Conn2/DIO_0_7 - 75kHz"=w130, "Conn2/DIO_0_7 In.Conn2/DIO_0_7 - uSec On"=w131, "Conn2/DIO_0_7 In.Conn2/DIO_0_7 In"=w132, "Conn2/DIO_0_7 In.Conn2/DIO_0_7 - uSec Off"=w133, "Conn2/DIO_8_15 In.Conn2/DIO_8_15 - 75kHz"=w96, "Conn2/DIO_8_15 In.Conn2/DIO_8_15 - uSec On"=w95, "Conn2/DIO_8_15 In.Conn2/DIO_8_15 In"=w94, "Conn2/DIO_8_15 In.Conn2/DIO_8_15 - uSec Off"=w93, "Conn2/DIO_16_23 In.Conn2/DIO_16_23 - 75kHz"=w92, "Conn2/DIO_16_23 In.Conn2/DIO_16_23 - uSec On"=w91, "Conn2/DIO_16_23 In.Conn2/DIO_16_23 In"=w90, "Conn2/DIO_16_23 In.Conn2/DIO_16_23 - uSec Off"=w89, "Conn2/DIO_24_31 In.Conn2/DIO_24_31 - 75kHz"=w88, "Conn2/DIO_24_31 In.Conn2/DIO_24_31 - uSec On"=w87, "Conn2/DIO_24_31 In.Conn2/DIO_24_31 In"=w86, "Conn2/DIO_24_31 In.Conn2/DIO_24_31 - uSec Off"=w85, "Conn2/DIO_32_39 In.Conn2/DIO_32_39 - 75kHz"=w84, "Conn2/DIO_32_39 In.Conn2/DIO_32_39 - uSec On"=w83, "Conn2/DIO_32_39 In.Conn2/DIO_32_39 In"=w82, "Conn2/DIO_32_39 In.Conn2/DIO_32_39 - uSec Off"=w81) -> (w80:T2)
        n11 = Build Array(w104, w103, w102, w101, w100, w99, w98, w97) -> (w143:i16[])
        n12 = xnode "Read/Write Control"("FPGA VI Reference In"=w125, "Conn0 DIOs In"=w128, "Conn1 DIOs In"=w142, "Conn2 DIOs In"=w80, "Connector0/AO0_7"=w143) -> ("FPGA VI Reference Out"=w126:refnum<k20>)  [unwired: 1 in, 1 out]
      }
      frame "Mono2 Relay Config" {
        w152 = FALSE  # Conn2/DIO_7
        w151 = FALSE  # Conn2/DIO_6
        w150 = FALSE  # Conn2/DIO_2
        w149 = FALSE  # Conn2/DIO_1
        w148 = FALSE  # Conn2/DIO_0
        w154 = u16 0  # Conn2/DIO_32_39 - uSec Off
        w155 = bool[] [FALSE, FALSE, FALSE, FALSE, FALSE, FALSE, FALSE, FALSE]  # Conn2/DIO_32_39 In
        w156 = u16 0  # Conn2/DIO_32_39 - uSec On
        w157 = FALSE  # Conn2/DIO_32_39 - 75kHz
        w158 = u16 0  # Conn2/DIO_24_31 - uSec Off
        w159 = bool[] [FALSE, FALSE, FALSE, FALSE, FALSE, FALSE, FALSE, FALSE]  # Conn2/DIO_24_31 In
        w160 = u16 0  # Conn2/DIO_24_31 - uSec On
        w161 = FALSE  # Conn2/DIO_24_31 - 75kHz
        w162 = u16 0  # Conn2/DIO_16_23 - uSec Off
        w163 = bool[] [FALSE, FALSE, FALSE, FALSE, FALSE, FALSE, FALSE, FALSE]  # Conn2/DIO_16_23 In
        w164 = u16 0  # Conn2/DIO_16_23 - uSec On
        w165 = FALSE  # Conn2/DIO_16_23 - 75kHz
        w166 = u16 0  # Conn2/DIO_8_15 - uSec Off
        w167 = bool[] [FALSE, FALSE, FALSE, FALSE, FALSE, FALSE, FALSE, FALSE]  # Conn2/DIO_8_15 In
        w168 = u16 0  # Conn2/DIO_8_15 - uSec On
        w169 = FALSE  # Conn2/DIO_8_15 - 75kHz
        w170 = i16 0  # Connector0/AO7
        w171 = i16 0  # Connector0/AO6
        w172 = i16 0  # Connector0/AO5
        w173 = i16 0  # Connector0/AO4
        w174 = i16 0  # Connector0/AO3
        w175 = i16 0  # Connector0/AO2
        w176 = i16 0  # Connector0/AO1
        w177 = i16 0  # Connector0/AO0
        w178 = u16 0  # Conn1/DIO_32_39 - uSec Off
        w179 = bool[] [FALSE, FALSE, FALSE, FALSE, FALSE, FALSE, FALSE, FALSE]  # Conn1/DIO_32_39 In
        w180 = u16 0  # Conn1/DIO_32_39 - uSec On
        w181 = FALSE  # Conn1/DIO_32_39 - 75kHz
        w182 = u16 0  # Conn1/DIO_24_31 - uSec Off
        w183 = bool[] [FALSE, FALSE, FALSE, FALSE, FALSE, FALSE, FALSE, FALSE]  # Conn1/DIO_24_31 In
        w184 = u16 0  # Conn1/DIO_24_31 - uSec On
        w185 = FALSE  # Conn1/DIO_24_31 - 75kHz
        w186 = u16 6  # Conn1/DIO_16_23 - uSec Off
        w187 = bool[] [FALSE, TRUE, FALSE, FALSE, FALSE, FALSE, FALSE, FALSE]  # Conn1/DIO_16_23 In
        w188 = u16 7  # Conn1/DIO_16_23 - uSec On
        w189 = TRUE  # Conn1/DIO_16_23 - 75kHz
        w190 = u16 6  # Conn1/DIO_8_15 - uSec Off
        w191 = bool[] [FALSE, FALSE, FALSE, TRUE, FALSE, FALSE, FALSE, FALSE]  # Conn1/DIO_8_15 In
        w192 = u16 7  # Conn1/DIO_8_15 - uSec On
        w193 = TRUE  # Conn1/DIO_8_15 - 75kHz
        w194 = u16 0  # Conn0/DIO_8_15 - uSec Off
        w195 = bool[] [FALSE, FALSE, FALSE, FALSE, FALSE, FALSE, FALSE, FALSE]  # Conn0/DIO_8_15 In
        w196 = u16 0  # Conn0/DIO_8_15 - uSec On
        w197 = FALSE  # Conn0/DIO_8_15 - 75kHz
        w213 = u16 0  # Conn0/DIO_0_7 - uSec Off
        w212 = bool[] [FALSE, FALSE, FALSE, FALSE, FALSE, FALSE, FALSE, FALSE]  # Conn0/DIO_0_7 In
        w211 = u16 0  # Conn0/DIO_0_7 - uSec On
        w210 = FALSE  # Conn0/DIO_0_7 - 75kHz
        w209 = u16 6  # Conn1/DIO_0_7 - uSec Off
        w208 = bool[] [FALSE, TRUE, TRUE, TRUE, TRUE, FALSE, FALSE, TRUE]  # Conn1/DIO_0_7 In
        w207 = u16 7  # Conn1/DIO_0_7 - uSec On
        w206 = TRUE  # Conn1/DIO_0_7 - 75kHz
        w205 = u16 6  # Conn2/DIO_0_7 - uSec Off
        w204 = u16 7  # Conn2/DIO_0_7 - uSec On
        w203 = TRUE  # Conn2/DIO_0_7 - 75kHz
        # "Mono2 Relay Config"
        # "Mono2 Relay Config"
        # "Mono2 Relay Config"
        n13 = Build Array(w148, w149, w150, w146, w145, w144, w151, w152) -> (w147:bool[])
        n14 = Bundle By Name(cluster=T4 {"Conn0/DIO_0_7 In"={"Conn0/DIO_0_7 - 75kHz"=FALSE, "Conn0/DIO_0_7 - uSec On"=0, "Conn0/DIO_0_7 In"=[FALSE, FALSE, FALSE, FALSE, FALSE, FALSE, FALSE, FALSE], "Conn0/DIO_0_7 - uSec Off"=0}, "Conn0/DIO_8_15 In"={"Conn0/DIO_8_15 - 75kHz"=FALSE, "Conn0/DIO_8_15 - uSec On"=0, "Conn0/DIO_8_15 In"=[FALSE, FALSE, FALSE, FALSE, FALSE, FALSE, FALSE, FALSE], "Conn0/DIO_8_15 - uSec Off"=0}} ("Conn0 DIOs In"), "Conn0/DIO_0_7 In.Conn0/DIO_0_7 - 75kHz"=w210, "Conn0/DIO_0_7 In.Conn0/DIO_0_7 - uSec On"=w211, "Conn0/DIO_0_7 In.Conn0/DIO_0_7 In"=w212, "Conn0/DIO_0_7 In.Conn0/DIO_0_7 - uSec Off"=w213, "Conn0/DIO_8_15 In.Conn0/DIO_8_15 - 75kHz"=w197, "Conn0/DIO_8_15 In.Conn0/DIO_8_15 - uSec On"=w196, "Conn0/DIO_8_15 In.Conn0/DIO_8_15 In"=w195, "Conn0/DIO_8_15 In.Conn0/DIO_8_15 - uSec Off"=w194) -> (w201:T4)
        n15 = Bundle By Name(cluster=T3 {"Conn1/DIO_0_7 In"={"Conn1/DIO_0_7 - 75kHz"=FALSE, "Conn1/DIO_0_7 - uSec On"=0, "Conn1/DIO_0_7 In"=[FALSE, FALSE, FALSE, FALSE, FALSE, FALSE, FALSE, FALSE], "Conn1/DIO_0_7 - uSec Off"=0}, "Conn1/DIO_8_15 In"={"Conn1/DIO_8_15 - 75kHz"=FALSE, "Conn1/DIO_8_15 - uSec On"=0, "Conn1/DIO_8_15 In"=[FALSE, FALSE, FALSE, FALSE, FALSE, FALSE, FALSE, FALSE], "Conn1/DIO_8_15 - uSec Off"=0}, "Conn1/DIO_16_23 In"={"Conn1/DIO_16_23 - 75kHz"=FALSE, "Conn1/DIO_16_23 - uSec On"=0, "Conn1/DIO_16_23 In"=[FALSE, FALSE, FALSE, FALSE, FALSE, FALSE, FALSE, FALSE], "Conn1/DIO_16_23 - uSec Off"=0}, "Conn1/DIO_24_31 In"={"Conn1/DIO_24_31 - 75kHz"=FALSE, "Conn1/DIO_24_31 - uSec On"=0, "Conn1/DIO_24_31 In"=[FALSE, FALSE, FALSE, FALSE, FALSE, FALSE, FALSE, FALSE], "Conn1/DIO_24_31 - uSec Off"=0}, "Conn1/DIO_32_39 In"={"Conn1/DIO_32_39 - 75kHz"=FALSE, "Conn1/DIO_32_39 - uSec On"=0, "Conn1/DIO_32_39 In"=[FALSE, FALSE, FALSE, FALSE, FALSE, FALSE, FALSE, FALSE], "Conn1/DIO_32_39 - uSec Off"=0}} ("Conn1 DIOs In"), "Conn1/DIO_0_7 In.Conn1/DIO_0_7 - 75kHz"=w206, "Conn1/DIO_0_7 In.Conn1/DIO_0_7 - uSec On"=w207, "Conn1/DIO_0_7 In.Conn1/DIO_0_7 In"=w208, "Conn1/DIO_0_7 In.Conn1/DIO_0_7 - uSec Off"=w209, "Conn1/DIO_8_15 In.Conn1/DIO_8_15 - 75kHz"=w193, "Conn1/DIO_8_15 In.Conn1/DIO_8_15 - uSec On"=w192, "Conn1/DIO_8_15 In.Conn1/DIO_8_15 In"=w191, "Conn1/DIO_8_15 In.Conn1/DIO_8_15 - uSec Off"=w190, "Conn1/DIO_16_23 In.Conn1/DIO_16_23 - 75kHz"=w189, "Conn1/DIO_16_23 In.Conn1/DIO_16_23 - uSec On"=w188, "Conn1/DIO_16_23 In.Conn1/DIO_16_23 In"=w187, "Conn1/DIO_16_23 In.Conn1/DIO_16_23 - uSec Off"=w186, "Conn1/DIO_24_31 In.Conn1/DIO_24_31 - 75kHz"=w185, "Conn1/DIO_24_31 In.Conn1/DIO_24_31 - uSec On"=w184, "Conn1/DIO_24_31 In.Conn1/DIO_24_31 In"=w183, "Conn1/DIO_24_31 In.Conn1/DIO_24_31 - uSec Off"=w182, "Conn1/DIO_32_39 In.Conn1/DIO_32_39 - 75kHz"=w181, "Conn1/DIO_32_39 In.Conn1/DIO_32_39 - uSec On"=w180, "Conn1/DIO_32_39 In.Conn1/DIO_32_39 In"=w179, "Conn1/DIO_32_39 In.Conn1/DIO_32_39 - uSec Off"=w178) -> (w214:T3)
        n16 = Bundle By Name(cluster=T2 {"Conn2/DIO_0_7 In"={"Conn2/DIO_0_7 - 75kHz"=FALSE, "Conn2/DIO_0_7 - uSec On"=0, "Conn2/DIO_0_7 In"=[FALSE, FALSE, FALSE, FALSE, FALSE, FALSE, FALSE, FALSE], "Conn2/DIO_0_7 - uSec Off"=0}, "Conn2/DIO_8_15 In"={"Conn2/DIO_8_15 - 75kHz"=FALSE, "Conn2/DIO_8_15 - uSec On"=0, "Conn2/DIO_8_15 In"=[FALSE, FALSE, FALSE, FALSE, FALSE, FALSE, FALSE, FALSE], "Conn2/DIO_8_15 - uSec Off"=0}, "Conn2/DIO_16_23 In"={"Conn2/DIO_16_23 - 75kHz"=FALSE, "Conn2/DIO_16_23 - uSec On"=0, "Conn2/DIO_16_23 In"=[FALSE, FALSE, FALSE, FALSE, FALSE, FALSE, FALSE, FALSE], "Conn2/DIO_16_23 - uSec Off"=0}, "Conn2/DIO_24_31 In"={"Conn2/DIO_24_31 - 75kHz"=FALSE, "Conn2/DIO_24_31 - uSec On"=0, "Conn2/DIO_24_31 In"=[FALSE, FALSE, FALSE, FALSE, FALSE, FALSE, FALSE, FALSE], "Conn2/DIO_24_31 - uSec Off"=0}, "Conn2/DIO_32_39 In"={"Conn2/DIO_32_39 - 75kHz"=FALSE, "Conn2/DIO_32_39 - uSec On"=0, "Conn2/DIO_32_39 In"=[FALSE, FALSE, FALSE, FALSE, FALSE, FALSE, FALSE, FALSE], "Conn2/DIO_32_39 - uSec Off"=0}} ("Conn2 DIOs In"), "Conn2/DIO_0_7 In.Conn2/DIO_0_7 - 75kHz"=w203, "Conn2/DIO_0_7 In.Conn2/DIO_0_7 - uSec On"=w204, "Conn2/DIO_0_7 In.Conn2/DIO_0_7 In"=w147, "Conn2/DIO_0_7 In.Conn2/DIO_0_7 - uSec Off"=w205, "Conn2/DIO_8_15 In.Conn2/DIO_8_15 - 75kHz"=w169, "Conn2/DIO_8_15 In.Conn2/DIO_8_15 - uSec On"=w168, "Conn2/DIO_8_15 In.Conn2/DIO_8_15 In"=w167, "Conn2/DIO_8_15 In.Conn2/DIO_8_15 - uSec Off"=w166, "Conn2/DIO_16_23 In.Conn2/DIO_16_23 - 75kHz"=w165, "Conn2/DIO_16_23 In.Conn2/DIO_16_23 - uSec On"=w164, "Conn2/DIO_16_23 In.Conn2/DIO_16_23 In"=w163, "Conn2/DIO_16_23 In.Conn2/DIO_16_23 - uSec Off"=w162, "Conn2/DIO_24_31 In.Conn2/DIO_24_31 - 75kHz"=w161, "Conn2/DIO_24_31 In.Conn2/DIO_24_31 - uSec On"=w160, "Conn2/DIO_24_31 In.Conn2/DIO_24_31 In"=w159, "Conn2/DIO_24_31 In.Conn2/DIO_24_31 - uSec Off"=w158, "Conn2/DIO_32_39 In.Conn2/DIO_32_39 - 75kHz"=w157, "Conn2/DIO_32_39 In.Conn2/DIO_32_39 - uSec On"=w156, "Conn2/DIO_32_39 In.Conn2/DIO_32_39 In"=w155, "Conn2/DIO_32_39 In.Conn2/DIO_32_39 - uSec Off"=w154) -> (w215:T2)
        n17 = Build Array(w177, w176, w175, w174, w173, w172, w171, w170) -> (w216:i16[])
        n18 = xnode "Read/Write Control"("FPGA VI Reference In"=w198, "Conn0 DIOs In"=w201, "Conn1 DIOs In"=w214, "Conn2 DIOs In"=w215, "Connector0/AO0_7"=w216) -> ("FPGA VI Reference Out"=w199:refnum<k20>)  [unwired: 1 in, 1 out]
      }
      frame "Bipolar Relay Config" {
        w218 = u16 0  # Conn2/DIO_32_39 - uSec Off
        w219 = bool[] [FALSE, FALSE, FALSE, FALSE, FALSE, FALSE, FALSE, FALSE]  # Conn2/DIO_32_39 In
        w220 = u16 0  # Conn2/DIO_32_39 - uSec On
        w221 = FALSE  # Conn2/DIO_32_39 - 75kHz
        w222 = u16 0  # Conn2/DIO_24_31 - uSec Off
        w223 = bool[] [FALSE, FALSE, FALSE, FALSE, FALSE, FALSE, FALSE, FALSE]  # Conn2/DIO_24_31 In
        w224 = u16 0  # Conn2/DIO_24_31 - uSec On
        w225 = FALSE  # Conn2/DIO_24_31 - 75kHz
        w226 = u16 0  # Conn2/DIO_16_23 - uSec Off
        w227 = bool[] [FALSE, FALSE, FALSE, FALSE, FALSE, FALSE, FALSE, FALSE]  # Conn2/DIO_16_23 In
        w228 = u16 0  # Conn2/DIO_16_23 - uSec On
        w229 = FALSE  # Conn2/DIO_16_23 - 75kHz
        w230 = u16 0  # Conn2/DIO_8_15 - uSec Off
        w231 = bool[] [FALSE, FALSE, FALSE, FALSE, FALSE, FALSE, FALSE, FALSE]  # Conn2/DIO_8_15 In
        w232 = u16 0  # Conn2/DIO_8_15 - uSec On
        w233 = FALSE  # Conn2/DIO_8_15 - 75kHz
        w234 = i16 0  # Connector0/AO7
        w235 = i16 0  # Connector0/AO6
        w236 = i16 0  # Connector0/AO5
        w237 = i16 0  # Connector0/AO4
        w238 = i16 0  # Connector0/AO3
        w239 = i16 0  # Connector0/AO2
        w240 = i16 0  # Connector0/AO1
        w241 = i16 0  # Connector0/AO0
        w242 = u16 0  # Conn1/DIO_32_39 - uSec Off
        w243 = bool[] [FALSE, FALSE, FALSE, FALSE, FALSE, FALSE, FALSE, FALSE]  # Conn1/DIO_32_39 In
        w244 = u16 0  # Conn1/DIO_32_39 - uSec On
        w245 = FALSE  # Conn1/DIO_32_39 - 75kHz
        w246 = u16 0  # Conn1/DIO_24_31 - uSec Off
        w247 = bool[] [FALSE, FALSE, FALSE, FALSE, FALSE, FALSE, FALSE, FALSE]  # Conn1/DIO_24_31 In
        w248 = u16 0  # Conn1/DIO_24_31 - uSec On
        w249 = FALSE  # Conn1/DIO_24_31 - 75kHz
        w250 = u16 6  # Conn1/DIO_16_23 - uSec Off
        w251 = bool[] [FALSE, TRUE, FALSE, FALSE, FALSE, FALSE, FALSE, FALSE]  # Conn1/DIO_16_23 In
        w252 = u16 7  # Conn1/DIO_16_23 - uSec On
        w253 = TRUE  # Conn1/DIO_16_23 - 75kHz
        w254 = u16 6  # Conn1/DIO_8_15 - uSec Off
        w255 = bool[] [TRUE, FALSE, FALSE, FALSE, FALSE, FALSE, FALSE, FALSE]  # Conn1/DIO_8_15 In
        w256 = u16 7  # Conn1/DIO_8_15 - uSec On
        w257 = TRUE  # Conn1/DIO_8_15 - 75kHz
        w258 = u16 0  # Conn0/DIO_8_15 - uSec Off
        w259 = bool[] [FALSE, FALSE, FALSE, FALSE, FALSE, FALSE, FALSE, FALSE]  # Conn0/DIO_8_15 In
        w260 = u16 0  # Conn0/DIO_8_15 - uSec On
        w261 = FALSE  # Conn0/DIO_8_15 - 75kHz
        w278 = u16 0  # Conn0/DIO_0_7 - uSec Off
        w277 = bool[] [FALSE, FALSE, FALSE, FALSE, FALSE, FALSE, FALSE, FALSE]  # Conn0/DIO_0_7 In
        w276 = u16 0  # Conn0/DIO_0_7 - uSec On
        w275 = FALSE  # Conn0/DIO_0_7 - 75kHz
        w274 = u16 6  # Conn1/DIO_0_7 - uSec Off
        w273 = bool[] [FALSE, TRUE, TRUE, TRUE, TRUE, FALSE, TRUE, FALSE]  # Conn1/DIO_0_7 In
        w272 = u16 7  # Conn1/DIO_0_7 - uSec On
        w271 = TRUE  # Conn1/DIO_0_7 - 75kHz
        w270 = u16 0  # Conn2/DIO_0_7 - uSec Off
        w269 = bool[] [FALSE, FALSE, FALSE, FALSE, FALSE, FALSE, FALSE, FALSE]  # Conn2/DIO_0_7 In
        w268 = u16 0  # Conn2/DIO_0_7 - uSec On
        w267 = FALSE  # Conn2/DIO_0_7 - 75kHz
        # "Bipolar Relay Config"
        # "Bipolar Relay Config"
        # "Bipolar Relay Config"
        n19 = Bundle By Name(cluster=T4 {"Conn0/DIO_0_7 In"={"Conn0/DIO_0_7 - 75kHz"=FALSE, "Conn0/DIO_0_7 - uSec On"=0, "Conn0/DIO_0_7 In"=[FALSE, FALSE, FALSE, FALSE, FALSE, FALSE, FALSE, FALSE], "Conn0/DIO_0_7 - uSec Off"=0}, "Conn0/DIO_8_15 In"={"Conn0/DIO_8_15 - 75kHz"=FALSE, "Conn0/DIO_8_15 - uSec On"=0, "Conn0/DIO_8_15 In"=[FALSE, FALSE, FALSE, FALSE, FALSE, FALSE, FALSE, FALSE], "Conn0/DIO_8_15 - uSec Off"=0}} ("Conn0 DIOs In"), "Conn0/DIO_0_7 In.Conn0/DIO_0_7 - 75kHz"=w275, "Conn0/DIO_0_7 In.Conn0/DIO_0_7 - uSec On"=w276, "Conn0/DIO_0_7 In.Conn0/DIO_0_7 In"=w277, "Conn0/DIO_0_7 In.Conn0/DIO_0_7 - uSec Off"=w278, "Conn0/DIO_8_15 In.Conn0/DIO_8_15 - 75kHz"=w261, "Conn0/DIO_8_15 In.Conn0/DIO_8_15 - uSec On"=w260, "Conn0/DIO_8_15 In.Conn0/DIO_8_15 In"=w259, "Conn0/DIO_8_15 In.Conn0/DIO_8_15 - uSec Off"=w258) -> (w265:T4)
        n20 = Bundle By Name(cluster=T3 {"Conn1/DIO_0_7 In"={"Conn1/DIO_0_7 - 75kHz"=FALSE, "Conn1/DIO_0_7 - uSec On"=0, "Conn1/DIO_0_7 In"=[FALSE, FALSE, FALSE, FALSE, FALSE, FALSE, FALSE, FALSE], "Conn1/DIO_0_7 - uSec Off"=0}, "Conn1/DIO_8_15 In"={"Conn1/DIO_8_15 - 75kHz"=FALSE, "Conn1/DIO_8_15 - uSec On"=0, "Conn1/DIO_8_15 In"=[FALSE, FALSE, FALSE, FALSE, FALSE, FALSE, FALSE, FALSE], "Conn1/DIO_8_15 - uSec Off"=0}, "Conn1/DIO_16_23 In"={"Conn1/DIO_16_23 - 75kHz"=FALSE, "Conn1/DIO_16_23 - uSec On"=0, "Conn1/DIO_16_23 In"=[FALSE, FALSE, FALSE, FALSE, FALSE, FALSE, FALSE, FALSE], "Conn1/DIO_16_23 - uSec Off"=0}, "Conn1/DIO_24_31 In"={"Conn1/DIO_24_31 - 75kHz"=FALSE, "Conn1/DIO_24_31 - uSec On"=0, "Conn1/DIO_24_31 In"=[FALSE, FALSE, FALSE, FALSE, FALSE, FALSE, FALSE, FALSE], "Conn1/DIO_24_31 - uSec Off"=0}, "Conn1/DIO_32_39 In"={"Conn1/DIO_32_39 - 75kHz"=FALSE, "Conn1/DIO_32_39 - uSec On"=0, "Conn1/DIO_32_39 In"=[FALSE, FALSE, FALSE, FALSE, FALSE, FALSE, FALSE, FALSE], "Conn1/DIO_32_39 - uSec Off"=0}} ("Conn1 DIOs In"), "Conn1/DIO_0_7 In.Conn1/DIO_0_7 - 75kHz"=w271, "Conn1/DIO_0_7 In.Conn1/DIO_0_7 - uSec On"=w272, "Conn1/DIO_0_7 In.Conn1/DIO_0_7 In"=w273, "Conn1/DIO_0_7 In.Conn1/DIO_0_7 - uSec Off"=w274, "Conn1/DIO_8_15 In.Conn1/DIO_8_15 - 75kHz"=w257, "Conn1/DIO_8_15 In.Conn1/DIO_8_15 - uSec On"=w256, "Conn1/DIO_8_15 In.Conn1/DIO_8_15 In"=w255, "Conn1/DIO_8_15 In.Conn1/DIO_8_15 - uSec Off"=w254, "Conn1/DIO_16_23 In.Conn1/DIO_16_23 - 75kHz"=w253, "Conn1/DIO_16_23 In.Conn1/DIO_16_23 - uSec On"=w252, "Conn1/DIO_16_23 In.Conn1/DIO_16_23 In"=w251, "Conn1/DIO_16_23 In.Conn1/DIO_16_23 - uSec Off"=w250, "Conn1/DIO_24_31 In.Conn1/DIO_24_31 - 75kHz"=w249, "Conn1/DIO_24_31 In.Conn1/DIO_24_31 - uSec On"=w248, "Conn1/DIO_24_31 In.Conn1/DIO_24_31 In"=w247, "Conn1/DIO_24_31 In.Conn1/DIO_24_31 - uSec Off"=w246, "Conn1/DIO_32_39 In.Conn1/DIO_32_39 - 75kHz"=w245, "Conn1/DIO_32_39 In.Conn1/DIO_32_39 - uSec On"=w244, "Conn1/DIO_32_39 In.Conn1/DIO_32_39 In"=w243, "Conn1/DIO_32_39 In.Conn1/DIO_32_39 - uSec Off"=w242) -> (w279:T3)
        n21 = Bundle By Name(cluster=T2 {"Conn2/DIO_0_7 In"={"Conn2/DIO_0_7 - 75kHz"=FALSE, "Conn2/DIO_0_7 - uSec On"=0, "Conn2/DIO_0_7 In"=[FALSE, FALSE, FALSE, FALSE, FALSE, FALSE, FALSE, FALSE], "Conn2/DIO_0_7 - uSec Off"=0}, "Conn2/DIO_8_15 In"={"Conn2/DIO_8_15 - 75kHz"=FALSE, "Conn2/DIO_8_15 - uSec On"=0, "Conn2/DIO_8_15 In"=[FALSE, FALSE, FALSE, FALSE, FALSE, FALSE, FALSE, FALSE], "Conn2/DIO_8_15 - uSec Off"=0}, "Conn2/DIO_16_23 In"={"Conn2/DIO_16_23 - 75kHz"=FALSE, "Conn2/DIO_16_23 - uSec On"=0, "Conn2/DIO_16_23 In"=[FALSE, FALSE, FALSE, FALSE, FALSE, FALSE, FALSE, FALSE], "Conn2/DIO_16_23 - uSec Off"=0}, "Conn2/DIO_24_31 In"={"Conn2/DIO_24_31 - 75kHz"=FALSE, "Conn2/DIO_24_31 - uSec On"=0, "Conn2/DIO_24_31 In"=[FALSE, FALSE, FALSE, FALSE, FALSE, FALSE, FALSE, FALSE], "Conn2/DIO_24_31 - uSec Off"=0}, "Conn2/DIO_32_39 In"={"Conn2/DIO_32_39 - 75kHz"=FALSE, "Conn2/DIO_32_39 - uSec On"=0, "Conn2/DIO_32_39 In"=[FALSE, FALSE, FALSE, FALSE, FALSE, FALSE, FALSE, FALSE], "Conn2/DIO_32_39 - uSec Off"=0}} ("Conn2 DIOs In"), "Conn2/DIO_0_7 In.Conn2/DIO_0_7 - 75kHz"=w267, "Conn2/DIO_0_7 In.Conn2/DIO_0_7 - uSec On"=w268, "Conn2/DIO_0_7 In.Conn2/DIO_0_7 In"=w269, "Conn2/DIO_0_7 In.Conn2/DIO_0_7 - uSec Off"=w270, "Conn2/DIO_8_15 In.Conn2/DIO_8_15 - 75kHz"=w233, "Conn2/DIO_8_15 In.Conn2/DIO_8_15 - uSec On"=w232, "Conn2/DIO_8_15 In.Conn2/DIO_8_15 In"=w231, "Conn2/DIO_8_15 In.Conn2/DIO_8_15 - uSec Off"=w230, "Conn2/DIO_16_23 In.Conn2/DIO_16_23 - 75kHz"=w229, "Conn2/DIO_16_23 In.Conn2/DIO_16_23 - uSec On"=w228, "Conn2/DIO_16_23 In.Conn2/DIO_16_23 In"=w227, "Conn2/DIO_16_23 In.Conn2/DIO_16_23 - uSec Off"=w226, "Conn2/DIO_24_31 In.Conn2/DIO_24_31 - 75kHz"=w225, "Conn2/DIO_24_31 In.Conn2/DIO_24_31 - uSec On"=w224, "Conn2/DIO_24_31 In.Conn2/DIO_24_31 In"=w223, "Conn2/DIO_24_31 In.Conn2/DIO_24_31 - uSec Off"=w222, "Conn2/DIO_32_39 In.Conn2/DIO_32_39 - 75kHz"=w221, "Conn2/DIO_32_39 In.Conn2/DIO_32_39 - uSec On"=w220, "Conn2/DIO_32_39 In.Conn2/DIO_32_39 In"=w219, "Conn2/DIO_32_39 In.Conn2/DIO_32_39 - uSec Off"=w218) -> (w280:T2)
        n22 = Build Array(w241, w240, w239, w238, w237, w236, w235, w234) -> (w281:i16[])
        n23 = xnode "Read/Write Control"("FPGA VI Reference In"=w262, "Conn0 DIOs In"=w265, "Conn1 DIOs In"=w279, "Conn2 DIOs In"=w280, "Connector0/AO0_7"=w281) -> ("FPGA VI Reference Out"=w263:refnum<k20>)  [unwired: 1 in, 1 out]
      }
      frame "Ligasure Relay Config" {
        w283 = u16 0  # Conn2/DIO_32_39 - uSec Off
        w284 = bool[] [FALSE, FALSE, FALSE, FALSE, FALSE, FALSE, FALSE, FALSE]  # Conn2/DIO_32_39 In
        w285 = u16 0  # Conn2/DIO_32_39 - uSec On
        w286 = FALSE  # Conn2/DIO_32_39 - 75kHz
        w287 = u16 0  # Conn2/DIO_24_31 - uSec Off
        w288 = bool[] [FALSE, FALSE, FALSE, FALSE, FALSE, FALSE, FALSE, FALSE]  # Conn2/DIO_24_31 In
        w289 = u16 0  # Conn2/DIO_24_31 - uSec On
        w290 = FALSE  # Conn2/DIO_24_31 - 75kHz
        w291 = u16 0  # Conn2/DIO_16_23 - uSec Off
        w292 = bool[] [FALSE, FALSE, FALSE, FALSE, FALSE, FALSE, FALSE, FALSE]  # Conn2/DIO_16_23 In
        w293 = u16 0  # Conn2/DIO_16_23 - uSec On
        w294 = FALSE  # Conn2/DIO_16_23 - 75kHz
        w295 = u16 0  # Conn2/DIO_8_15 - uSec Off
        w296 = bool[] [FALSE, FALSE, FALSE, FALSE, FALSE, FALSE, FALSE, FALSE]  # Conn2/DIO_8_15 In
        w297 = u16 0  # Conn2/DIO_8_15 - uSec On
        w298 = FALSE  # Conn2/DIO_8_15 - 75kHz
        w299 = i16 0  # Connector0/AO7
        w300 = i16 0  # Connector0/AO6
        w301 = i16 0  # Connector0/AO5
        w302 = i16 0  # Connector0/AO4
        w303 = i16 0  # Connector0/AO3
        w304 = i16 0  # Connector0/AO2
        w305 = i16 0  # Connector0/AO1
        w306 = i16 0  # Connector0/AO0
        w307 = u16 0  # Conn1/DIO_32_39 - uSec Off
        w308 = bool[] [FALSE, FALSE, FALSE, FALSE, FALSE, FALSE, FALSE, FALSE]  # Conn1/DIO_32_39 In
        w309 = u16 0  # Conn1/DIO_32_39 - uSec On
        w310 = FALSE  # Conn1/DIO_32_39 - 75kHz
        w311 = u16 0  # Conn1/DIO_24_31 - uSec Off
        w312 = bool[] [FALSE, FALSE, FALSE, FALSE, FALSE, FALSE, FALSE, FALSE]  # Conn1/DIO_24_31 In
        w313 = u16 0  # Conn1/DIO_24_31 - uSec On
        w314 = FALSE  # Conn1/DIO_24_31 - 75kHz
        w315 = u16 6  # Conn1/DIO_16_23 - uSec Off
        w316 = bool[] [FALSE, TRUE, FALSE, FALSE, FALSE, FALSE, FALSE, FALSE]  # Conn1/DIO_16_23 In
        w317 = u16 7  # Conn1/DIO_16_23 - uSec On
        w318 = TRUE  # Conn1/DIO_16_23 - 75kHz
        w319 = u16 6  # Conn1/DIO_8_15 - uSec Off
        w320 = bool[] [FALSE, TRUE, FALSE, FALSE, FALSE, FALSE, FALSE, FALSE]  # Conn1/DIO_8_15 In
        w321 = u16 7  # Conn1/DIO_8_15 - uSec On
        w322 = TRUE  # Conn1/DIO_8_15 - 75kHz
        w323 = u16 0  # Conn0/DIO_8_15 - uSec Off
        w324 = bool[] [FALSE, FALSE, FALSE, FALSE, FALSE, FALSE, FALSE, FALSE]  # Conn0/DIO_8_15 In
        w325 = u16 0  # Conn0/DIO_8_15 - uSec On
        w326 = FALSE  # Conn0/DIO_8_15 - 75kHz
        w343 = u16 0  # Conn0/DIO_0_7 - uSec Off
        w342 = bool[] [FALSE, FALSE, FALSE, FALSE, FALSE, FALSE, FALSE, FALSE]  # Conn0/DIO_0_7 In
        w341 = u16 0  # Conn0/DIO_0_7 - uSec On
        w340 = FALSE  # Conn0/DIO_0_7 - 75kHz
        w339 = u16 6  # Conn1/DIO_0_7 - uSec Off
        w338 = bool[] [FALSE, TRUE, TRUE, TRUE, TRUE, TRUE, FALSE, FALSE]  # Conn1/DIO_0_7 In
        w337 = u16 7  # Conn1/DIO_0_7 - uSec On
        w336 = TRUE  # Conn1/DIO_0_7 - 75kHz
        w335 = u16 0  # Conn2/DIO_0_7 - uSec Off
        w334 = bool[] [FALSE, FALSE, FALSE, FALSE, FALSE, FALSE, FALSE, FALSE]  # Conn2/DIO_0_7 In
        w333 = u16 0  # Conn2/DIO_0_7 - uSec On
        w332 = FALSE  # Conn2/DIO_0_7 - 75kHz
        # "Ligasure Relay Config"
        # "Ligasure Relay Config"
        # "Ligasure Relay Config"
        n24 = Bundle By Name(cluster=T4 {"Conn0/DIO_0_7 In"={"Conn0/DIO_0_7 - 75kHz"=FALSE, "Conn0/DIO_0_7 - uSec On"=0, "Conn0/DIO_0_7 In"=[FALSE, FALSE, FALSE, FALSE, FALSE, FALSE, FALSE, FALSE], "Conn0/DIO_0_7 - uSec Off"=0}, "Conn0/DIO_8_15 In"={"Conn0/DIO_8_15 - 75kHz"=FALSE, "Conn0/DIO_8_15 - uSec On"=0, "Conn0/DIO_8_15 In"=[FALSE, FALSE, FALSE, FALSE, FALSE, FALSE, FALSE, FALSE], "Conn0/DIO_8_15 - uSec Off"=0}} ("Conn0 DIOs In"), "Conn0/DIO_0_7 In.Conn0/DIO_0_7 - 75kHz"=w340, "Conn0/DIO_0_7 In.Conn0/DIO_0_7 - uSec On"=w341, "Conn0/DIO_0_7 In.Conn0/DIO_0_7 In"=w342, "Conn0/DIO_0_7 In.Conn0/DIO_0_7 - uSec Off"=w343, "Conn0/DIO_8_15 In.Conn0/DIO_8_15 - 75kHz"=w326, "Conn0/DIO_8_15 In.Conn0/DIO_8_15 - uSec On"=w325, "Conn0/DIO_8_15 In.Conn0/DIO_8_15 In"=w324, "Conn0/DIO_8_15 In.Conn0/DIO_8_15 - uSec Off"=w323) -> (w330:T4)
        n25 = Bundle By Name(cluster=T3 {"Conn1/DIO_0_7 In"={"Conn1/DIO_0_7 - 75kHz"=FALSE, "Conn1/DIO_0_7 - uSec On"=0, "Conn1/DIO_0_7 In"=[FALSE, FALSE, FALSE, FALSE, FALSE, FALSE, FALSE, FALSE], "Conn1/DIO_0_7 - uSec Off"=0}, "Conn1/DIO_8_15 In"={"Conn1/DIO_8_15 - 75kHz"=FALSE, "Conn1/DIO_8_15 - uSec On"=0, "Conn1/DIO_8_15 In"=[FALSE, FALSE, FALSE, FALSE, FALSE, FALSE, FALSE, FALSE], "Conn1/DIO_8_15 - uSec Off"=0}, "Conn1/DIO_16_23 In"={"Conn1/DIO_16_23 - 75kHz"=FALSE, "Conn1/DIO_16_23 - uSec On"=0, "Conn1/DIO_16_23 In"=[FALSE, FALSE, FALSE, FALSE, FALSE, FALSE, FALSE, FALSE], "Conn1/DIO_16_23 - uSec Off"=0}, "Conn1/DIO_24_31 In"={"Conn1/DIO_24_31 - 75kHz"=FALSE, "Conn1/DIO_24_31 - uSec On"=0, "Conn1/DIO_24_31 In"=[FALSE, FALSE, FALSE, FALSE, FALSE, FALSE, FALSE, FALSE], "Conn1/DIO_24_31 - uSec Off"=0}, "Conn1/DIO_32_39 In"={"Conn1/DIO_32_39 - 75kHz"=FALSE, "Conn1/DIO_32_39 - uSec On"=0, "Conn1/DIO_32_39 In"=[FALSE, FALSE, FALSE, FALSE, FALSE, FALSE, FALSE, FALSE], "Conn1/DIO_32_39 - uSec Off"=0}} ("Conn1 DIOs In"), "Conn1/DIO_0_7 In.Conn1/DIO_0_7 - 75kHz"=w336, "Conn1/DIO_0_7 In.Conn1/DIO_0_7 - uSec On"=w337, "Conn1/DIO_0_7 In.Conn1/DIO_0_7 In"=w338, "Conn1/DIO_0_7 In.Conn1/DIO_0_7 - uSec Off"=w339, "Conn1/DIO_8_15 In.Conn1/DIO_8_15 - 75kHz"=w322, "Conn1/DIO_8_15 In.Conn1/DIO_8_15 - uSec On"=w321, "Conn1/DIO_8_15 In.Conn1/DIO_8_15 In"=w320, "Conn1/DIO_8_15 In.Conn1/DIO_8_15 - uSec Off"=w319, "Conn1/DIO_16_23 In.Conn1/DIO_16_23 - 75kHz"=w318, "Conn1/DIO_16_23 In.Conn1/DIO_16_23 - uSec On"=w317, "Conn1/DIO_16_23 In.Conn1/DIO_16_23 In"=w316, "Conn1/DIO_16_23 In.Conn1/DIO_16_23 - uSec Off"=w315, "Conn1/DIO_24_31 In.Conn1/DIO_24_31 - 75kHz"=w314, "Conn1/DIO_24_31 In.Conn1/DIO_24_31 - uSec On"=w313, "Conn1/DIO_24_31 In.Conn1/DIO_24_31 In"=w312, "Conn1/DIO_24_31 In.Conn1/DIO_24_31 - uSec Off"=w311, "Conn1/DIO_32_39 In.Conn1/DIO_32_39 - 75kHz"=w310, "Conn1/DIO_32_39 In.Conn1/DIO_32_39 - uSec On"=w309, "Conn1/DIO_32_39 In.Conn1/DIO_32_39 In"=w308, "Conn1/DIO_32_39 In.Conn1/DIO_32_39 - uSec Off"=w307) -> (w344:T3)
        n26 = Bundle By Name(cluster=T2 {"Conn2/DIO_0_7 In"={"Conn2/DIO_0_7 - 75kHz"=FALSE, "Conn2/DIO_0_7 - uSec On"=0, "Conn2/DIO_0_7 In"=[FALSE, FALSE, FALSE, FALSE, FALSE, FALSE, FALSE, FALSE], "Conn2/DIO_0_7 - uSec Off"=0}, "Conn2/DIO_8_15 In"={"Conn2/DIO_8_15 - 75kHz"=FALSE, "Conn2/DIO_8_15 - uSec On"=0, "Conn2/DIO_8_15 In"=[FALSE, FALSE, FALSE, FALSE, FALSE, FALSE, FALSE, FALSE], "Conn2/DIO_8_15 - uSec Off"=0}, "Conn2/DIO_16_23 In"={"Conn2/DIO_16_23 - 75kHz"=FALSE, "Conn2/DIO_16_23 - uSec On"=0, "Conn2/DIO_16_23 In"=[FALSE, FALSE, FALSE, FALSE, FALSE, FALSE, FALSE, FALSE], "Conn2/DIO_16_23 - uSec Off"=0}, "Conn2/DIO_24_31 In"={"Conn2/DIO_24_31 - 75kHz"=FALSE, "Conn2/DIO_24_31 - uSec On"=0, "Conn2/DIO_24_31 In"=[FALSE, FALSE, FALSE, FALSE, FALSE, FALSE, FALSE, FALSE], "Conn2/DIO_24_31 - uSec Off"=0}, "Conn2/DIO_32_39 In"={"Conn2/DIO_32_39 - 75kHz"=FALSE, "Conn2/DIO_32_39 - uSec On"=0, "Conn2/DIO_32_39 In"=[FALSE, FALSE, FALSE, FALSE, FALSE, FALSE, FALSE, FALSE], "Conn2/DIO_32_39 - uSec Off"=0}} ("Conn2 DIOs In"), "Conn2/DIO_0_7 In.Conn2/DIO_0_7 - 75kHz"=w332, "Conn2/DIO_0_7 In.Conn2/DIO_0_7 - uSec On"=w333, "Conn2/DIO_0_7 In.Conn2/DIO_0_7 In"=w334, "Conn2/DIO_0_7 In.Conn2/DIO_0_7 - uSec Off"=w335, "Conn2/DIO_8_15 In.Conn2/DIO_8_15 - 75kHz"=w298, "Conn2/DIO_8_15 In.Conn2/DIO_8_15 - uSec On"=w297, "Conn2/DIO_8_15 In.Conn2/DIO_8_15 In"=w296, "Conn2/DIO_8_15 In.Conn2/DIO_8_15 - uSec Off"=w295, "Conn2/DIO_16_23 In.Conn2/DIO_16_23 - 75kHz"=w294, "Conn2/DIO_16_23 In.Conn2/DIO_16_23 - uSec On"=w293, "Conn2/DIO_16_23 In.Conn2/DIO_16_23 In"=w292, "Conn2/DIO_16_23 In.Conn2/DIO_16_23 - uSec Off"=w291, "Conn2/DIO_24_31 In.Conn2/DIO_24_31 - 75kHz"=w290, "Conn2/DIO_24_31 In.Conn2/DIO_24_31 - uSec On"=w289, "Conn2/DIO_24_31 In.Conn2/DIO_24_31 In"=w288, "Conn2/DIO_24_31 In.Conn2/DIO_24_31 - uSec Off"=w287, "Conn2/DIO_32_39 In.Conn2/DIO_32_39 - 75kHz"=w286, "Conn2/DIO_32_39 In.Conn2/DIO_32_39 - uSec On"=w285, "Conn2/DIO_32_39 In.Conn2/DIO_32_39 In"=w284, "Conn2/DIO_32_39 In.Conn2/DIO_32_39 - uSec Off"=w283) -> (w345:T2)
        n27 = Build Array(w306, w305, w304, w303, w302, w301, w300, w299) -> (w346:i16[])
        n28 = xnode "Read/Write Control"("FPGA VI Reference In"=w327, "Conn0 DIOs In"=w330, "Conn1 DIOs In"=w344, "Conn2 DIOs In"=w345, "Connector0/AO0_7"=w346) -> ("FPGA VI Reference Out"=w328:refnum<k20>)  [unwired: 1 in, 1 out]
      }
      frame "Handswitch - Mono1 Cut" {
        w348 = u16 0  # Conn2/DIO_32_39 - uSec Off
        w349 = bool[] [FALSE, FALSE, FALSE, FALSE, FALSE, FALSE, FALSE, FALSE]  # Conn2/DIO_32_39 In
        w350 = u16 0  # Conn2/DIO_32_39 - uSec On
        w351 = FALSE  # Conn2/DIO_32_39 - 75kHz
        w352 = u16 0  # Conn2/DIO_24_31 - uSec Off
        w353 = bool[] [FALSE, FALSE, FALSE, FALSE, FALSE, FALSE, FALSE, FALSE]  # Conn2/DIO_24_31 In
        w354 = u16 0  # Conn2/DIO_24_31 - uSec On
        w355 = FALSE  # Conn2/DIO_24_31 - 75kHz
        w356 = u16 0  # Conn2/DIO_16_23 - uSec Off
        w357 = bool[] [FALSE, FALSE, FALSE, FALSE, FALSE, FALSE, FALSE, FALSE]  # Conn2/DIO_16_23 In
        w358 = u16 0  # Conn2/DIO_16_23 - uSec On
        w359 = FALSE  # Conn2/DIO_16_23 - 75kHz
        w360 = u16 0  # Conn2/DIO_8_15 - uSec Off
        w361 = bool[] [FALSE, FALSE, FALSE, FALSE, FALSE, FALSE, FALSE, FALSE]  # Conn2/DIO_8_15 In
        w362 = u16 0  # Conn2/DIO_8_15 - uSec On
        w363 = FALSE  # Conn2/DIO_8_15 - 75kHz
        w364 = i16 0  # Connector0/AO7
        w365 = i16 0  # Connector0/AO6
        w366 = i16 0  # Connector0/AO5
        w367 = i16 0  # Connector0/AO4
        w368 = i16 0  # Connector0/AO3
        w369 = i16 0  # Connector0/AO2
        w370 = i16 0  # Connector0/AO1
        w371 = i16 0  # Connector0/AO0
        w372 = u16 0  # Conn1/DIO_32_39 - uSec Off
        w373 = bool[] [FALSE, FALSE, FALSE, FALSE, FALSE, FALSE, FALSE, FALSE]  # Conn1/DIO_32_39 In
        w374 = u16 0  # Conn1/DIO_32_39 - uSec On
        w375 = FALSE  # Conn1/DIO_32_39 - 75kHz
        w376 = u16 0  # Conn1/DIO_24_31 - uSec Off
        w377 = bool[] [FALSE, FALSE, FALSE, FALSE, FALSE, FALSE, FALSE, FALSE]  # Conn1/DIO_24_31 In
        w378 = u16 0  # Conn1/DIO_24_31 - uSec On
        w379 = FALSE  # Conn1/DIO_24_31 - 75kHz
        w380 = u16 6  # Conn1/DIO_16_23 - uSec Off
        w381 = bool[] [FALSE, TRUE, FALSE, FALSE, FALSE, TRUE, FALSE, FALSE]  # Conn1/DIO_16_23 In
        w382 = u16 7  # Conn1/DIO_16_23 - uSec On
        w383 = TRUE  # Conn1/DIO_16_23 - 75kHz
        w384 = u16 6  # Conn1/DIO_8_15 - uSec Off
        w385 = bool[] [FALSE, FALSE, FALSE, TRUE, FALSE, FALSE, FALSE, FALSE]  # Conn1/DIO_8_15 In
        w386 = u16 7  # Conn1/DIO_8_15 - uSec On
        w387 = TRUE  # Conn1/DIO_8_15 - 75kHz
        w388 = u16 0  # Conn0/DIO_8_15 - uSec Off
        w389 = bool[] [FALSE, FALSE, FALSE, FALSE, FALSE, FALSE, FALSE, FALSE]  # Conn0/DIO_8_15 In
        w390 = u16 0  # Conn0/DIO_8_15 - uSec On
        w391 = FALSE  # Conn0/DIO_8_15 - 75kHz
        w408 = u16 0  # Conn0/DIO_0_7 - uSec Off
        w407 = bool[] [FALSE, FALSE, FALSE, FALSE, FALSE, FALSE, FALSE, FALSE]  # Conn0/DIO_0_7 In
        w406 = u16 0  # Conn0/DIO_0_7 - uSec On
        w405 = FALSE  # Conn0/DIO_0_7 - 75kHz
        w404 = u16 6  # Conn1/DIO_0_7 - uSec Off
        w403 = bool[] [TRUE, TRUE, TRUE, TRUE, TRUE, FALSE, FALSE, FALSE]  # Conn1/DIO_0_7 In
        w402 = u16 7  # Conn1/DIO_0_7 - uSec On
        w401 = TRUE  # Conn1/DIO_0_7 - 75kHz
        w400 = u16 0  # Conn2/DIO_0_7 - uSec Off
        w399 = bool[] [FALSE, FALSE, FALSE, FALSE, FALSE, FALSE, FALSE, FALSE]  # Conn2/DIO_0_7 In
        w398 = u16 0  # Conn2/DIO_0_7 - uSec On
        w397 = FALSE  # Conn2/DIO_0_7 - 75kHz
        # "Handswitch - Mono1 Cut"
        # "Handswitch - Mono1 Cut"
        # "Handswitch - Mono1 Cut"
        n29 = Bundle By Name(cluster=T4 {"Conn0/DIO_0_7 In"={"Conn0/DIO_0_7 - 75kHz"=FALSE, "Conn0/DIO_0_7 - uSec On"=0, "Conn0/DIO_0_7 In"=[FALSE, FALSE, FALSE, FALSE, FALSE, FALSE, FALSE, FALSE], "Conn0/DIO_0_7 - uSec Off"=0}, "Conn0/DIO_8_15 In"={"Conn0/DIO_8_15 - 75kHz"=FALSE, "Conn0/DIO_8_15 - uSec On"=0, "Conn0/DIO_8_15 In"=[FALSE, FALSE, FALSE, FALSE, FALSE, FALSE, FALSE, FALSE], "Conn0/DIO_8_15 - uSec Off"=0}} ("Conn0 DIOs In"), "Conn0/DIO_0_7 In.Conn0/DIO_0_7 - 75kHz"=w405, "Conn0/DIO_0_7 In.Conn0/DIO_0_7 - uSec On"=w406, "Conn0/DIO_0_7 In.Conn0/DIO_0_7 In"=w407, "Conn0/DIO_0_7 In.Conn0/DIO_0_7 - uSec Off"=w408, "Conn0/DIO_8_15 In.Conn0/DIO_8_15 - 75kHz"=w391, "Conn0/DIO_8_15 In.Conn0/DIO_8_15 - uSec On"=w390, "Conn0/DIO_8_15 In.Conn0/DIO_8_15 In"=w389, "Conn0/DIO_8_15 In.Conn0/DIO_8_15 - uSec Off"=w388) -> (w395:T4)
        n30 = Bundle By Name(cluster=T3 {"Conn1/DIO_0_7 In"={"Conn1/DIO_0_7 - 75kHz"=FALSE, "Conn1/DIO_0_7 - uSec On"=0, "Conn1/DIO_0_7 In"=[FALSE, FALSE, FALSE, FALSE, FALSE, FALSE, FALSE, FALSE], "Conn1/DIO_0_7 - uSec Off"=0}, "Conn1/DIO_8_15 In"={"Conn1/DIO_8_15 - 75kHz"=FALSE, "Conn1/DIO_8_15 - uSec On"=0, "Conn1/DIO_8_15 In"=[FALSE, FALSE, FALSE, FALSE, FALSE, FALSE, FALSE, FALSE], "Conn1/DIO_8_15 - uSec Off"=0}, "Conn1/DIO_16_23 In"={"Conn1/DIO_16_23 - 75kHz"=FALSE, "Conn1/DIO_16_23 - uSec On"=0, "Conn1/DIO_16_23 In"=[FALSE, FALSE, FALSE, FALSE, FALSE, FALSE, FALSE, FALSE], "Conn1/DIO_16_23 - uSec Off"=0}, "Conn1/DIO_24_31 In"={"Conn1/DIO_24_31 - 75kHz"=FALSE, "Conn1/DIO_24_31 - uSec On"=0, "Conn1/DIO_24_31 In"=[FALSE, FALSE, FALSE, FALSE, FALSE, FALSE, FALSE, FALSE], "Conn1/DIO_24_31 - uSec Off"=0}, "Conn1/DIO_32_39 In"={"Conn1/DIO_32_39 - 75kHz"=FALSE, "Conn1/DIO_32_39 - uSec On"=0, "Conn1/DIO_32_39 In"=[FALSE, FALSE, FALSE, FALSE, FALSE, FALSE, FALSE, FALSE], "Conn1/DIO_32_39 - uSec Off"=0}} ("Conn1 DIOs In"), "Conn1/DIO_0_7 In.Conn1/DIO_0_7 - 75kHz"=w401, "Conn1/DIO_0_7 In.Conn1/DIO_0_7 - uSec On"=w402, "Conn1/DIO_0_7 In.Conn1/DIO_0_7 In"=w403, "Conn1/DIO_0_7 In.Conn1/DIO_0_7 - uSec Off"=w404, "Conn1/DIO_8_15 In.Conn1/DIO_8_15 - 75kHz"=w387, "Conn1/DIO_8_15 In.Conn1/DIO_8_15 - uSec On"=w386, "Conn1/DIO_8_15 In.Conn1/DIO_8_15 In"=w385, "Conn1/DIO_8_15 In.Conn1/DIO_8_15 - uSec Off"=w384, "Conn1/DIO_16_23 In.Conn1/DIO_16_23 - 75kHz"=w383, "Conn1/DIO_16_23 In.Conn1/DIO_16_23 - uSec On"=w382, "Conn1/DIO_16_23 In.Conn1/DIO_16_23 In"=w381, "Conn1/DIO_16_23 In.Conn1/DIO_16_23 - uSec Off"=w380, "Conn1/DIO_24_31 In.Conn1/DIO_24_31 - 75kHz"=w379, "Conn1/DIO_24_31 In.Conn1/DIO_24_31 - uSec On"=w378, "Conn1/DIO_24_31 In.Conn1/DIO_24_31 In"=w377, "Conn1/DIO_24_31 In.Conn1/DIO_24_31 - uSec Off"=w376, "Conn1/DIO_32_39 In.Conn1/DIO_32_39 - 75kHz"=w375, "Conn1/DIO_32_39 In.Conn1/DIO_32_39 - uSec On"=w374, "Conn1/DIO_32_39 In.Conn1/DIO_32_39 In"=w373, "Conn1/DIO_32_39 In.Conn1/DIO_32_39 - uSec Off"=w372) -> (w409:T3)
        n31 = Bundle By Name(cluster=T2 {"Conn2/DIO_0_7 In"={"Conn2/DIO_0_7 - 75kHz"=FALSE, "Conn2/DIO_0_7 - uSec On"=0, "Conn2/DIO_0_7 In"=[FALSE, FALSE, FALSE, FALSE, FALSE, FALSE, FALSE, FALSE], "Conn2/DIO_0_7 - uSec Off"=0}, "Conn2/DIO_8_15 In"={"Conn2/DIO_8_15 - 75kHz"=FALSE, "Conn2/DIO_8_15 - uSec On"=0, "Conn2/DIO_8_15 In"=[FALSE, FALSE, FALSE, FALSE, FALSE, FALSE, FALSE, FALSE], "Conn2/DIO_8_15 - uSec Off"=0}, "Conn2/DIO_16_23 In"={"Conn2/DIO_16_23 - 75kHz"=FALSE, "Conn2/DIO_16_23 - uSec On"=0, "Conn2/DIO_16_23 In"=[FALSE, FALSE, FALSE, FALSE, FALSE, FALSE, FALSE, FALSE], "Conn2/DIO_16_23 - uSec Off"=0}, "Conn2/DIO_24_31 In"={"Conn2/DIO_24_31 - 75kHz"=FALSE, "Conn2/DIO_24_31 - uSec On"=0, "Conn2/DIO_24_31 In"=[FALSE, FALSE, FALSE, FALSE, FALSE, FALSE, FALSE, FALSE], "Conn2/DIO_24_31 - uSec Off"=0}, "Conn2/DIO_32_39 In"={"Conn2/DIO_32_39 - 75kHz"=FALSE, "Conn2/DIO_32_39 - uSec On"=0, "Conn2/DIO_32_39 In"=[FALSE, FALSE, FALSE, FALSE, FALSE, FALSE, FALSE, FALSE], "Conn2/DIO_32_39 - uSec Off"=0}} ("Conn2 DIOs In"), "Conn2/DIO_0_7 In.Conn2/DIO_0_7 - 75kHz"=w397, "Conn2/DIO_0_7 In.Conn2/DIO_0_7 - uSec On"=w398, "Conn2/DIO_0_7 In.Conn2/DIO_0_7 In"=w399, "Conn2/DIO_0_7 In.Conn2/DIO_0_7 - uSec Off"=w400, "Conn2/DIO_8_15 In.Conn2/DIO_8_15 - 75kHz"=w363, "Conn2/DIO_8_15 In.Conn2/DIO_8_15 - uSec On"=w362, "Conn2/DIO_8_15 In.Conn2/DIO_8_15 In"=w361, "Conn2/DIO_8_15 In.Conn2/DIO_8_15 - uSec Off"=w360, "Conn2/DIO_16_23 In.Conn2/DIO_16_23 - 75kHz"=w359, "Conn2/DIO_16_23 In.Conn2/DIO_16_23 - uSec On"=w358, "Conn2/DIO_16_23 In.Conn2/DIO_16_23 In"=w357, "Conn2/DIO_16_23 In.Conn2/DIO_16_23 - uSec Off"=w356, "Conn2/DIO_24_31 In.Conn2/DIO_24_31 - 75kHz"=w355, "Conn2/DIO_24_31 In.Conn2/DIO_24_31 - uSec On"=w354, "Conn2/DIO_24_31 In.Conn2/DIO_24_31 In"=w353, "Conn2/DIO_24_31 In.Conn2/DIO_24_31 - uSec Off"=w352, "Conn2/DIO_32_39 In.Conn2/DIO_32_39 - 75kHz"=w351, "Conn2/DIO_32_39 In.Conn2/DIO_32_39 - uSec On"=w350, "Conn2/DIO_32_39 In.Conn2/DIO_32_39 In"=w349, "Conn2/DIO_32_39 In.Conn2/DIO_32_39 - uSec Off"=w348) -> (w410:T2)
        n32 = Build Array(w371, w370, w369, w368, w367, w366, w365, w364) -> (w411:i16[])
        n33 = xnode "Read/Write Control"("FPGA VI Reference In"=w392, "Conn0 DIOs In"=w395, "Conn1 DIOs In"=w409, "Conn2 DIOs In"=w410, "Connector0/AO0_7"=w411) -> ("FPGA VI Reference Out"=w393:refnum<k20>)  [unwired: 1 in, 1 out]
      }
      frame "Handswitch - Mono1 Coag" {
        w413 = u16 0  # Conn2/DIO_32_39 - uSec Off
        w414 = bool[] [FALSE, FALSE, FALSE, FALSE, FALSE, FALSE, FALSE, FALSE]  # Conn2/DIO_32_39 In
        w415 = u16 0  # Conn2/DIO_32_39 - uSec On
        w416 = FALSE  # Conn2/DIO_32_39 - 75kHz
        w417 = u16 0  # Conn2/DIO_24_31 - uSec Off
        w418 = bool[] [FALSE, FALSE, FALSE, FALSE, FALSE, FALSE, FALSE, FALSE]  # Conn2/DIO_24_31 In
        w419 = u16 0  # Conn2/DIO_24_31 - uSec On
        w420 = FALSE  # Conn2/DIO_24_31 - 75kHz
        w421 = u16 0  # Conn2/DIO_16_23 - uSec Off
        w422 = bool[] [FALSE, FALSE, FALSE, FALSE, FALSE, FALSE, FALSE, FALSE]  # Conn2/DIO_16_23 In
        w423 = u16 0  # Conn2/DIO_16_23 - uSec On
        w424 = FALSE  # Conn2/DIO_16_23 - 75kHz
        w425 = u16 0  # Conn2/DIO_8_15 - uSec Off
        w426 = bool[] [FALSE, FALSE, FALSE, FALSE, FALSE, FALSE, FALSE, FALSE]  # Conn2/DIO_8_15 In
        w427 = u16 0  # Conn2/DIO_8_15 - uSec On
        w428 = FALSE  # Conn2/DIO_8_15 - 75kHz
        w429 = i16 0  # Connector0/AO7
        w430 = i16 0  # Connector0/AO6
        w431 = i16 0  # Connector0/AO5
        w432 = i16 0  # Connector0/AO4
        w433 = i16 0  # Connector0/AO3
        w434 = i16 0  # Connector0/AO2
        w435 = i16 0  # Connector0/AO1
        w436 = i16 0  # Connector0/AO0
        w437 = u16 0  # Conn1/DIO_32_39 - uSec Off
        w438 = bool[] [FALSE, FALSE, FALSE, FALSE, FALSE, FALSE, FALSE, FALSE]  # Conn1/DIO_32_39 In
        w439 = u16 0  # Conn1/DIO_32_39 - uSec On
        w440 = FALSE  # Conn1/DIO_32_39 - 75kHz
        w441 = u16 0  # Conn1/DIO_24_31 - uSec Off
        w442 = bool[] [FALSE, FALSE, FALSE, FALSE, FALSE, FALSE, FALSE, FALSE]  # Conn1/DIO_24_31 In
        w443 = u16 0  # Conn1/DIO_24_31 - uSec On
        w444 = FALSE  # Conn1/DIO_24_31 - 75kHz
        w445 = u16 6  # Conn1/DIO_16_23 - uSec Off
        w446 = bool[] [FALSE, TRUE, FALSE, FALSE, TRUE, FALSE, FALSE, FALSE]  # Conn1/DIO_16_23 In
        w447 = u16 7  # Conn1/DIO_16_23 - uSec On
        w448 = TRUE  # Conn1/DIO_16_23 - 75kHz
        w449 = u16 6  # Conn1/DIO_8_15 - uSec Off
        w450 = bool[] [FALSE, FALSE, FALSE, TRUE, FALSE, FALSE, FALSE, FALSE]  # Conn1/DIO_8_15 In
        w451 = u16 7  # Conn1/DIO_8_15 - uSec On
        w452 = TRUE  # Conn1/DIO_8_15 - 75kHz
        w453 = u16 0  # Conn0/DIO_8_15 - uSec Off
        w454 = bool[] [FALSE, FALSE, FALSE, FALSE, FALSE, FALSE, FALSE, FALSE]  # Conn0/DIO_8_15 In
        w455 = u16 0  # Conn0/DIO_8_15 - uSec On
        w456 = FALSE  # Conn0/DIO_8_15 - 75kHz
        w473 = u16 0  # Conn0/DIO_0_7 - uSec Off
        w472 = bool[] [FALSE, FALSE, FALSE, FALSE, FALSE, FALSE, FALSE, FALSE]  # Conn0/DIO_0_7 In
        w471 = u16 0  # Conn0/DIO_0_7 - uSec On
        w470 = FALSE  # Conn0/DIO_0_7 - 75kHz
        w469 = u16 6  # Conn1/DIO_0_7 - uSec Off
        w468 = bool[] [TRUE, TRUE, TRUE, TRUE, TRUE, FALSE, FALSE, FALSE]  # Conn1/DIO_0_7 In
        w467 = u16 7  # Conn1/DIO_0_7 - uSec On
        w466 = TRUE  # Conn1/DIO_0_7 - 75kHz
        w465 = u16 0  # Conn2/DIO_0_7 - uSec Off
        w464 = bool[] [FALSE, FALSE, FALSE, FALSE, FALSE, FALSE, FALSE, FALSE]  # Conn2/DIO_0_7 In
        w463 = u16 0  # Conn2/DIO_0_7 - uSec On
        w462 = FALSE  # Conn2/DIO_0_7 - 75kHz
        # "Handswitch - Mono1 Coag"
        # "Handswitch - Mono1 Coag"
        # "Handswitch - Mono1 Coag"
        n34 = Bundle By Name(cluster=T4 {"Conn0/DIO_0_7 In"={"Conn0/DIO_0_7 - 75kHz"=FALSE, "Conn0/DIO_0_7 - uSec On"=0, "Conn0/DIO_0_7 In"=[FALSE, FALSE, FALSE, FALSE, FALSE, FALSE, FALSE, FALSE], "Conn0/DIO_0_7 - uSec Off"=0}, "Conn0/DIO_8_15 In"={"Conn0/DIO_8_15 - 75kHz"=FALSE, "Conn0/DIO_8_15 - uSec On"=0, "Conn0/DIO_8_15 In"=[FALSE, FALSE, FALSE, FALSE, FALSE, FALSE, FALSE, FALSE], "Conn0/DIO_8_15 - uSec Off"=0}} ("Conn0 DIOs In"), "Conn0/DIO_0_7 In.Conn0/DIO_0_7 - 75kHz"=w470, "Conn0/DIO_0_7 In.Conn0/DIO_0_7 - uSec On"=w471, "Conn0/DIO_0_7 In.Conn0/DIO_0_7 In"=w472, "Conn0/DIO_0_7 In.Conn0/DIO_0_7 - uSec Off"=w473, "Conn0/DIO_8_15 In.Conn0/DIO_8_15 - 75kHz"=w456, "Conn0/DIO_8_15 In.Conn0/DIO_8_15 - uSec On"=w455, "Conn0/DIO_8_15 In.Conn0/DIO_8_15 In"=w454, "Conn0/DIO_8_15 In.Conn0/DIO_8_15 - uSec Off"=w453) -> (w460:T4)
        n35 = Bundle By Name(cluster=T3 {"Conn1/DIO_0_7 In"={"Conn1/DIO_0_7 - 75kHz"=FALSE, "Conn1/DIO_0_7 - uSec On"=0, "Conn1/DIO_0_7 In"=[FALSE, FALSE, FALSE, FALSE, FALSE, FALSE, FALSE, FALSE], "Conn1/DIO_0_7 - uSec Off"=0}, "Conn1/DIO_8_15 In"={"Conn1/DIO_8_15 - 75kHz"=FALSE, "Conn1/DIO_8_15 - uSec On"=0, "Conn1/DIO_8_15 In"=[FALSE, FALSE, FALSE, FALSE, FALSE, FALSE, FALSE, FALSE], "Conn1/DIO_8_15 - uSec Off"=0}, "Conn1/DIO_16_23 In"={"Conn1/DIO_16_23 - 75kHz"=FALSE, "Conn1/DIO_16_23 - uSec On"=0, "Conn1/DIO_16_23 In"=[FALSE, FALSE, FALSE, FALSE, FALSE, FALSE, FALSE, FALSE], "Conn1/DIO_16_23 - uSec Off"=0}, "Conn1/DIO_24_31 In"={"Conn1/DIO_24_31 - 75kHz"=FALSE, "Conn1/DIO_24_31 - uSec On"=0, "Conn1/DIO_24_31 In"=[FALSE, FALSE, FALSE, FALSE, FALSE, FALSE, FALSE, FALSE], "Conn1/DIO_24_31 - uSec Off"=0}, "Conn1/DIO_32_39 In"={"Conn1/DIO_32_39 - 75kHz"=FALSE, "Conn1/DIO_32_39 - uSec On"=0, "Conn1/DIO_32_39 In"=[FALSE, FALSE, FALSE, FALSE, FALSE, FALSE, FALSE, FALSE], "Conn1/DIO_32_39 - uSec Off"=0}} ("Conn1 DIOs In"), "Conn1/DIO_0_7 In.Conn1/DIO_0_7 - 75kHz"=w466, "Conn1/DIO_0_7 In.Conn1/DIO_0_7 - uSec On"=w467, "Conn1/DIO_0_7 In.Conn1/DIO_0_7 In"=w468, "Conn1/DIO_0_7 In.Conn1/DIO_0_7 - uSec Off"=w469, "Conn1/DIO_8_15 In.Conn1/DIO_8_15 - 75kHz"=w452, "Conn1/DIO_8_15 In.Conn1/DIO_8_15 - uSec On"=w451, "Conn1/DIO_8_15 In.Conn1/DIO_8_15 In"=w450, "Conn1/DIO_8_15 In.Conn1/DIO_8_15 - uSec Off"=w449, "Conn1/DIO_16_23 In.Conn1/DIO_16_23 - 75kHz"=w448, "Conn1/DIO_16_23 In.Conn1/DIO_16_23 - uSec On"=w447, "Conn1/DIO_16_23 In.Conn1/DIO_16_23 In"=w446, "Conn1/DIO_16_23 In.Conn1/DIO_16_23 - uSec Off"=w445, "Conn1/DIO_24_31 In.Conn1/DIO_24_31 - 75kHz"=w444, "Conn1/DIO_24_31 In.Conn1/DIO_24_31 - uSec On"=w443, "Conn1/DIO_24_31 In.Conn1/DIO_24_31 In"=w442, "Conn1/DIO_24_31 In.Conn1/DIO_24_31 - uSec Off"=w441, "Conn1/DIO_32_39 In.Conn1/DIO_32_39 - 75kHz"=w440, "Conn1/DIO_32_39 In.Conn1/DIO_32_39 - uSec On"=w439, "Conn1/DIO_32_39 In.Conn1/DIO_32_39 In"=w438, "Conn1/DIO_32_39 In.Conn1/DIO_32_39 - uSec Off"=w437) -> (w474:T3)
        n36 = Bundle By Name(cluster=T2 {"Conn2/DIO_0_7 In"={"Conn2/DIO_0_7 - 75kHz"=FALSE, "Conn2/DIO_0_7 - uSec On"=0, "Conn2/DIO_0_7 In"=[FALSE, FALSE, FALSE, FALSE, FALSE, FALSE, FALSE, FALSE], "Conn2/DIO_0_7 - uSec Off"=0}, "Conn2/DIO_8_15 In"={"Conn2/DIO_8_15 - 75kHz"=FALSE, "Conn2/DIO_8_15 - uSec On"=0, "Conn2/DIO_8_15 In"=[FALSE, FALSE, FALSE, FALSE, FALSE, FALSE, FALSE, FALSE], "Conn2/DIO_8_15 - uSec Off"=0}, "Conn2/DIO_16_23 In"={"Conn2/DIO_16_23 - 75kHz"=FALSE, "Conn2/DIO_16_23 - uSec On"=0, "Conn2/DIO_16_23 In"=[FALSE, FALSE, FALSE, FALSE, FALSE, FALSE, FALSE, FALSE], "Conn2/DIO_16_23 - uSec Off"=0}, "Conn2/DIO_24_31 In"={"Conn2/DIO_24_31 - 75kHz"=FALSE, "Conn2/DIO_24_31 - uSec On"=0, "Conn2/DIO_24_31 In"=[FALSE, FALSE, FALSE, FALSE, FALSE, FALSE, FALSE, FALSE], "Conn2/DIO_24_31 - uSec Off"=0}, "Conn2/DIO_32_39 In"={"Conn2/DIO_32_39 - 75kHz"=FALSE, "Conn2/DIO_32_39 - uSec On"=0, "Conn2/DIO_32_39 In"=[FALSE, FALSE, FALSE, FALSE, FALSE, FALSE, FALSE, FALSE], "Conn2/DIO_32_39 - uSec Off"=0}} ("Conn2 DIOs In"), "Conn2/DIO_0_7 In.Conn2/DIO_0_7 - 75kHz"=w462, "Conn2/DIO_0_7 In.Conn2/DIO_0_7 - uSec On"=w463, "Conn2/DIO_0_7 In.Conn2/DIO_0_7 In"=w464, "Conn2/DIO_0_7 In.Conn2/DIO_0_7 - uSec Off"=w465, "Conn2/DIO_8_15 In.Conn2/DIO_8_15 - 75kHz"=w428, "Conn2/DIO_8_15 In.Conn2/DIO_8_15 - uSec On"=w427, "Conn2/DIO_8_15 In.Conn2/DIO_8_15 In"=w426, "Conn2/DIO_8_15 In.Conn2/DIO_8_15 - uSec Off"=w425, "Conn2/DIO_16_23 In.Conn2/DIO_16_23 - 75kHz"=w424, "Conn2/DIO_16_23 In.Conn2/DIO_16_23 - uSec On"=w423, "Conn2/DIO_16_23 In.Conn2/DIO_16_23 In"=w422, "Conn2/DIO_16_23 In.Conn2/DIO_16_23 - uSec Off"=w421, "Conn2/DIO_24_31 In.Conn2/DIO_24_31 - 75kHz"=w420, "Conn2/DIO_24_31 In.Conn2/DIO_24_31 - uSec On"=w419, "Conn2/DIO_24_31 In.Conn2/DIO_24_31 In"=w418, "Conn2/DIO_24_31 In.Conn2/DIO_24_31 - uSec Off"=w417, "Conn2/DIO_32_39 In.Conn2/DIO_32_39 - 75kHz"=w416, "Conn2/DIO_32_39 In.Conn2/DIO_32_39 - uSec On"=w415, "Conn2/DIO_32_39 In.Conn2/DIO_32_39 In"=w414, "Conn2/DIO_32_39 In.Conn2/DIO_32_39 - uSec Off"=w413) -> (w475:T2)
        n37 = Build Array(w436, w435, w434, w433, w432, w431, w430, w429) -> (w476:i16[])
        n38 = xnode "Read/Write Control"("FPGA VI Reference In"=w457, "Conn0 DIOs In"=w460, "Conn1 DIOs In"=w474, "Conn2 DIOs In"=w475, "Connector0/AO0_7"=w476) -> ("FPGA VI Reference Out"=w458:refnum<k20>)  [unwired: 1 in, 1 out]
      }
      frame "Handswitch - Mono2 Cut" {
        w478 = u16 0  # Conn2/DIO_32_39 - uSec Off
        w479 = bool[] [FALSE, FALSE, FALSE, FALSE, FALSE, FALSE, FALSE, FALSE]  # Conn2/DIO_32_39 In
        w480 = u16 0  # Conn2/DIO_32_39 - uSec On
        w481 = FALSE  # Conn2/DIO_32_39 - 75kHz
        w482 = u16 0  # Conn2/DIO_24_31 - uSec Off
        w483 = bool[] [FALSE, FALSE, FALSE, FALSE, FALSE, FALSE, FALSE, FALSE]  # Conn2/DIO_24_31 In
        w484 = u16 0  # Conn2/DIO_24_31 - uSec On
        w485 = FALSE  # Conn2/DIO_24_31 - 75kHz
        w486 = u16 0  # Conn2/DIO_16_23 - uSec Off
        w487 = bool[] [FALSE, FALSE, FALSE, FALSE, FALSE, FALSE, FALSE, FALSE]  # Conn2/DIO_16_23 In
        w488 = u16 0  # Conn2/DIO_16_23 - uSec On
        w489 = FALSE  # Conn2/DIO_16_23 - 75kHz
        w490 = u16 0  # Conn2/DIO_8_15 - uSec Off
        w491 = bool[] [FALSE, FALSE, FALSE, FALSE, FALSE, FALSE, FALSE, FALSE]  # Conn2/DIO_8_15 In
        w492 = u16 0  # Conn2/DIO_8_15 - uSec On
        w493 = FALSE  # Conn2/DIO_8_15 - 75kHz
        w494 = i16 0  # Connector0/AO7
        w495 = i16 0  # Connector0/AO6
        w496 = i16 0  # Connector0/AO5
        w497 = i16 0  # Connector0/AO4
        w498 = i16 0  # Connector0/AO3
        w499 = i16 0  # Connector0/AO2
        w500 = i16 0  # Connector0/AO1
        w501 = i16 0  # Connector0/AO0
        w502 = u16 0  # Conn1/DIO_32_39 - uSec Off
        w503 = bool[] [FALSE, FALSE, FALSE, FALSE, FALSE, FALSE, FALSE, FALSE]  # Conn1/DIO_32_39 In
        w504 = u16 0  # Conn1/DIO_32_39 - uSec On
        w505 = FALSE  # Conn1/DIO_32_39 - 75kHz
        w506 = u16 6  # Conn1/DIO_24_31 - uSec Off
        w507 = bool[] [TRUE, FALSE, FALSE, FALSE, FALSE, FALSE, FALSE, FALSE]  # Conn1/DIO_24_31 In
        w508 = u16 7  # Conn1/DIO_24_31 - uSec On
        w509 = TRUE  # Conn1/DIO_24_31 - 75kHz
        w510 = u16 6  # Conn1/DIO_16_23 - uSec Off
        w511 = bool[] [FALSE, TRUE, FALSE, FALSE, FALSE, FALSE, FALSE, FALSE]  # Conn1/DIO_16_23 In
        w512 = u16 7  # Conn1/DIO_16_23 - uSec On
        w513 = TRUE  # Conn1/DIO_16_23 - 75kHz
        w514 = u16 6  # Conn1/DIO_8_15 - uSec Off
        w515 = bool[] [FALSE, FALSE, FALSE, TRUE, FALSE, FALSE, FALSE, FALSE]  # Conn1/DIO_8_15 In
        w516 = u16 7  # Conn1/DIO_8_15 - uSec On
        w517 = TRUE  # Conn1/DIO_8_15 - 75kHz
        w518 = u16 0  # Conn0/DIO_8_15 - uSec Off
        w519 = bool[] [FALSE, FALSE, FALSE, FALSE, FALSE, FALSE, FALSE, FALSE]  # Conn0/DIO_8_15 In
        w520 = u16 0  # Conn0/DIO_8_15 - uSec On
        w521 = FALSE  # Conn0/DIO_8_15 - 75kHz
        w538 = u16 0  # Conn0/DIO_0_7 - uSec Off
        w537 = bool[] [FALSE, FALSE, FALSE, FALSE, FALSE, FALSE, FALSE, FALSE]  # Conn0/DIO_0_7 In
        w536 = u16 0  # Conn0/DIO_0_7 - uSec On
        w535 = FALSE  # Conn0/DIO_0_7 - 75kHz
        w534 = u16 6  # Conn1/DIO_0_7 - uSec Off
        w533 = bool[] [FALSE, TRUE, TRUE, TRUE, TRUE, FALSE, FALSE, TRUE]  # Conn1/DIO_0_7 In
        w532 = u16 7  # Conn1/DIO_0_7 - uSec On
        w531 = TRUE  # Conn1/DIO_0_7 - 75kHz
        w530 = u16 0  # Conn2/DIO_0_7 - uSec Off
        w529 = bool[] [FALSE, FALSE, FALSE, FALSE, FALSE, FALSE, FALSE, FALSE]  # Conn2/DIO_0_7 In
        w528 = u16 0  # Conn2/DIO_0_7 - uSec On
        w527 = FALSE  # Conn2/DIO_0_7 - 75kHz
        # "Handswitch - Mono2 Cut"
        # "Handswitch - Mono2 Cut"
        # "Handswitch - Mono2 Cut"
        n39 = Bundle By Name(cluster=T4 {"Conn0/DIO_0_7 In"={"Conn0/DIO_0_7 - 75kHz"=FALSE, "Conn0/DIO_0_7 - uSec On"=0, "Conn0/DIO_0_7 In"=[FALSE, FALSE, FALSE, FALSE, FALSE, FALSE, FALSE, FALSE], "Conn0/DIO_0_7 - uSec Off"=0}, "Conn0/DIO_8_15 In"={"Conn0/DIO_8_15 - 75kHz"=FALSE, "Conn0/DIO_8_15 - uSec On"=0, "Conn0/DIO_8_15 In"=[FALSE, FALSE, FALSE, FALSE, FALSE, FALSE, FALSE, FALSE], "Conn0/DIO_8_15 - uSec Off"=0}} ("Conn0 DIOs In"), "Conn0/DIO_0_7 In.Conn0/DIO_0_7 - 75kHz"=w535, "Conn0/DIO_0_7 In.Conn0/DIO_0_7 - uSec On"=w536, "Conn0/DIO_0_7 In.Conn0/DIO_0_7 In"=w537, "Conn0/DIO_0_7 In.Conn0/DIO_0_7 - uSec Off"=w538, "Conn0/DIO_8_15 In.Conn0/DIO_8_15 - 75kHz"=w521, "Conn0/DIO_8_15 In.Conn0/DIO_8_15 - uSec On"=w520, "Conn0/DIO_8_15 In.Conn0/DIO_8_15 In"=w519, "Conn0/DIO_8_15 In.Conn0/DIO_8_15 - uSec Off"=w518) -> (w525:T4)
        n40 = Bundle By Name(cluster=T3 {"Conn1/DIO_0_7 In"={"Conn1/DIO_0_7 - 75kHz"=FALSE, "Conn1/DIO_0_7 - uSec On"=0, "Conn1/DIO_0_7 In"=[FALSE, FALSE, FALSE, FALSE, FALSE, FALSE, FALSE, FALSE], "Conn1/DIO_0_7 - uSec Off"=0}, "Conn1/DIO_8_15 In"={"Conn1/DIO_8_15 - 75kHz"=FALSE, "Conn1/DIO_8_15 - uSec On"=0, "Conn1/DIO_8_15 In"=[FALSE, FALSE, FALSE, FALSE, FALSE, FALSE, FALSE, FALSE], "Conn1/DIO_8_15 - uSec Off"=0}, "Conn1/DIO_16_23 In"={"Conn1/DIO_16_23 - 75kHz"=FALSE, "Conn1/DIO_16_23 - uSec On"=0, "Conn1/DIO_16_23 In"=[FALSE, FALSE, FALSE, FALSE, FALSE, FALSE, FALSE, FALSE], "Conn1/DIO_16_23 - uSec Off"=0}, "Conn1/DIO_24_31 In"={"Conn1/DIO_24_31 - 75kHz"=FALSE, "Conn1/DIO_24_31 - uSec On"=0, "Conn1/DIO_24_31 In"=[FALSE, FALSE, FALSE, FALSE, FALSE, FALSE, FALSE, FALSE], "Conn1/DIO_24_31 - uSec Off"=0}, "Conn1/DIO_32_39 In"={"Conn1/DIO_32_39 - 75kHz"=FALSE, "Conn1/DIO_32_39 - uSec On"=0, "Conn1/DIO_32_39 In"=[FALSE, FALSE, FALSE, FALSE, FALSE, FALSE, FALSE, FALSE], "Conn1/DIO_32_39 - uSec Off"=0}} ("Conn1 DIOs In"), "Conn1/DIO_0_7 In.Conn1/DIO_0_7 - 75kHz"=w531, "Conn1/DIO_0_7 In.Conn1/DIO_0_7 - uSec On"=w532, "Conn1/DIO_0_7 In.Conn1/DIO_0_7 In"=w533, "Conn1/DIO_0_7 In.Conn1/DIO_0_7 - uSec Off"=w534, "Conn1/DIO_8_15 In.Conn1/DIO_8_15 - 75kHz"=w517, "Conn1/DIO_8_15 In.Conn1/DIO_8_15 - uSec On"=w516, "Conn1/DIO_8_15 In.Conn1/DIO_8_15 In"=w515, "Conn1/DIO_8_15 In.Conn1/DIO_8_15 - uSec Off"=w514, "Conn1/DIO_16_23 In.Conn1/DIO_16_23 - 75kHz"=w513, "Conn1/DIO_16_23 In.Conn1/DIO_16_23 - uSec On"=w512, "Conn1/DIO_16_23 In.Conn1/DIO_16_23 In"=w511, "Conn1/DIO_16_23 In.Conn1/DIO_16_23 - uSec Off"=w510, "Conn1/DIO_24_31 In.Conn1/DIO_24_31 - 75kHz"=w509, "Conn1/DIO_24_31 In.Conn1/DIO_24_31 - uSec On"=w508, "Conn1/DIO_24_31 In.Conn1/DIO_24_31 In"=w507, "Conn1/DIO_24_31 In.Conn1/DIO_24_31 - uSec Off"=w506, "Conn1/DIO_32_39 In.Conn1/DIO_32_39 - 75kHz"=w505, "Conn1/DIO_32_39 In.Conn1/DIO_32_39 - uSec On"=w504, "Conn1/DIO_32_39 In.Conn1/DIO_32_39 In"=w503, "Conn1/DIO_32_39 In.Conn1/DIO_32_39 - uSec Off"=w502) -> (w539:T3)
        n41 = Bundle By Name(cluster=T2 {"Conn2/DIO_0_7 In"={"Conn2/DIO_0_7 - 75kHz"=FALSE, "Conn2/DIO_0_7 - uSec On"=0, "Conn2/DIO_0_7 In"=[FALSE, FALSE, FALSE, FALSE, FALSE, FALSE, FALSE, FALSE], "Conn2/DIO_0_7 - uSec Off"=0}, "Conn2/DIO_8_15 In"={"Conn2/DIO_8_15 - 75kHz"=FALSE, "Conn2/DIO_8_15 - uSec On"=0, "Conn2/DIO_8_15 In"=[FALSE, FALSE, FALSE, FALSE, FALSE, FALSE, FALSE, FALSE], "Conn2/DIO_8_15 - uSec Off"=0}, "Conn2/DIO_16_23 In"={"Conn2/DIO_16_23 - 75kHz"=FALSE, "Conn2/DIO_16_23 - uSec On"=0, "Conn2/DIO_16_23 In"=[FALSE, FALSE, FALSE, FALSE, FALSE, FALSE, FALSE, FALSE], "Conn2/DIO_16_23 - uSec Off"=0}, "Conn2/DIO_24_31 In"={"Conn2/DIO_24_31 - 75kHz"=FALSE, "Conn2/DIO_24_31 - uSec On"=0, "Conn2/DIO_24_31 In"=[FALSE, FALSE, FALSE, FALSE, FALSE, FALSE, FALSE, FALSE], "Conn2/DIO_24_31 - uSec Off"=0}, "Conn2/DIO_32_39 In"={"Conn2/DIO_32_39 - 75kHz"=FALSE, "Conn2/DIO_32_39 - uSec On"=0, "Conn2/DIO_32_39 In"=[FALSE, FALSE, FALSE, FALSE, FALSE, FALSE, FALSE, FALSE], "Conn2/DIO_32_39 - uSec Off"=0}} ("Conn2 DIOs In"), "Conn2/DIO_0_7 In.Conn2/DIO_0_7 - 75kHz"=w527, "Conn2/DIO_0_7 In.Conn2/DIO_0_7 - uSec On"=w528, "Conn2/DIO_0_7 In.Conn2/DIO_0_7 In"=w529, "Conn2/DIO_0_7 In.Conn2/DIO_0_7 - uSec Off"=w530, "Conn2/DIO_8_15 In.Conn2/DIO_8_15 - 75kHz"=w493, "Conn2/DIO_8_15 In.Conn2/DIO_8_15 - uSec On"=w492, "Conn2/DIO_8_15 In.Conn2/DIO_8_15 In"=w491, "Conn2/DIO_8_15 In.Conn2/DIO_8_15 - uSec Off"=w490, "Conn2/DIO_16_23 In.Conn2/DIO_16_23 - 75kHz"=w489, "Conn2/DIO_16_23 In.Conn2/DIO_16_23 - uSec On"=w488, "Conn2/DIO_16_23 In.Conn2/DIO_16_23 In"=w487, "Conn2/DIO_16_23 In.Conn2/DIO_16_23 - uSec Off"=w486, "Conn2/DIO_24_31 In.Conn2/DIO_24_31 - 75kHz"=w485, "Conn2/DIO_24_31 In.Conn2/DIO_24_31 - uSec On"=w484, "Conn2/DIO_24_31 In.Conn2/DIO_24_31 In"=w483, "Conn2/DIO_24_31 In.Conn2/DIO_24_31 - uSec Off"=w482, "Conn2/DIO_32_39 In.Conn2/DIO_32_39 - 75kHz"=w481, "Conn2/DIO_32_39 In.Conn2/DIO_32_39 - uSec On"=w480, "Conn2/DIO_32_39 In.Conn2/DIO_32_39 In"=w479, "Conn2/DIO_32_39 In.Conn2/DIO_32_39 - uSec Off"=w478) -> (w540:T2)
        n42 = Build Array(w501, w500, w499, w498, w497, w496, w495, w494) -> (w541:i16[])
        n43 = xnode "Read/Write Control"("FPGA VI Reference In"=w522, "Conn0 DIOs In"=w525, "Conn1 DIOs In"=w539, "Conn2 DIOs In"=w540, "Connector0/AO0_7"=w541) -> ("FPGA VI Reference Out"=w523:refnum<k20>)  [unwired: 1 in, 1 out]
      }
      frame "Handswitch - Mono2 Coag" {
        w543 = u16 0  # Conn2/DIO_32_39 - uSec Off
        w544 = bool[] [FALSE, FALSE, FALSE, FALSE, FALSE, FALSE, FALSE, FALSE]  # Conn2/DIO_32_39 In
        w545 = u16 0  # Conn2/DIO_32_39 - uSec On
        w546 = FALSE  # Conn2/DIO_32_39 - 75kHz
        w547 = u16 0  # Conn2/DIO_24_31 - uSec Off
        w548 = bool[] [FALSE, FALSE, FALSE, FALSE, FALSE, FALSE, FALSE, FALSE]  # Conn2/DIO_24_31 In
        w549 = u16 0  # Conn2/DIO_24_31 - uSec On
        w550 = FALSE  # Conn2/DIO_24_31 - 75kHz
        w551 = u16 0  # Conn2/DIO_16_23 - uSec Off
        w552 = bool[] [FALSE, FALSE, FALSE, FALSE, FALSE, FALSE, FALSE, FALSE]  # Conn2/DIO_16_23 In
        w553 = u16 0  # Conn2/DIO_16_23 - uSec On
        w554 = FALSE  # Conn2/DIO_16_23 - 75kHz
        w555 = u16 0  # Conn2/DIO_8_15 - uSec Off
        w556 = bool[] [FALSE, FALSE, FALSE, FALSE, FALSE, FALSE, FALSE, FALSE]  # Conn2/DIO_8_15 In
        w557 = u16 0  # Conn2/DIO_8_15 - uSec On
        w558 = FALSE  # Conn2/DIO_8_15 - 75kHz
        w559 = i16 0  # Connector0/AO7
        w560 = i16 0  # Connector0/AO6
        w561 = i16 0  # Connector0/AO5
        w562 = i16 0  # Connector0/AO4
        w563 = i16 0  # Connector0/AO3
        w564 = i16 0  # Connector0/AO2
        w565 = i16 0  # Connector0/AO1
        w566 = i16 0  # Connector0/AO0
        w567 = u16 0  # Conn1/DIO_32_39 - uSec Off
        w568 = bool[] [FALSE, FALSE, FALSE, FALSE, FALSE, FALSE, FALSE, FALSE]  # Conn1/DIO_32_39 In
        w569 = u16 0  # Conn1/DIO_32_39 - uSec On
        w570 = FALSE  # Conn1/DIO_32_39 - 75kHz
        w571 = u16 6  # Conn1/DIO_24_31 - uSec Off
        w572 = bool[] [FALSE, TRUE, FALSE, FALSE, FALSE, FALSE, FALSE, FALSE]  # Conn1/DIO_24_31 In
        w573 = u16 7  # Conn1/DIO_24_31 - uSec On
        w574 = TRUE  # Conn1/DIO_24_31 - 75kHz
        w575 = u16 6  # Conn1/DIO_16_23 - uSec Off
        w576 = bool[] [FALSE, TRUE, FALSE, FALSE, FALSE, FALSE, FALSE, FALSE]  # Conn1/DIO_16_23 In
        w577 = u16 7  # Conn1/DIO_16_23 - uSec On
        w578 = TRUE  # Conn1/DIO_16_23 - 75kHz
        w579 = u16 6  # Conn1/DIO_8_15 - uSec Off
        w580 = bool[] [FALSE, FALSE, FALSE, TRUE, FALSE, FALSE, FALSE, FALSE]  # Conn1/DIO_8_15 In
        w581 = u16 7  # Conn1/DIO_8_15 - uSec On
        w582 = TRUE  # Conn1/DIO_8_15 - 75kHz
        w583 = u16 0  # Conn0/DIO_8_15 - uSec Off
        w584 = bool[] [FALSE, FALSE, FALSE, FALSE, FALSE, FALSE, FALSE, FALSE]  # Conn0/DIO_8_15 In
        w585 = u16 0  # Conn0/DIO_8_15 - uSec On
        w586 = FALSE  # Conn0/DIO_8_15 - 75kHz
        w603 = u16 0  # Conn0/DIO_0_7 - uSec Off
        w602 = bool[] [FALSE, FALSE, FALSE, FALSE, FALSE, FALSE, FALSE, FALSE]  # Conn0/DIO_0_7 In
        w601 = u16 0  # Conn0/DIO_0_7 - uSec On
        w600 = FALSE  # Conn0/DIO_0_7 - 75kHz
        w599 = u16 6  # Conn1/DIO_0_7 - uSec Off
        w598 = bool[] [FALSE, TRUE, TRUE, TRUE, TRUE, FALSE, FALSE, TRUE]  # Conn1/DIO_0_7 In
        w597 = u16 7  # Conn1/DIO_0_7 - uSec On
        w596 = TRUE  # Conn1/DIO_0_7 - 75kHz
        w595 = u16 0  # Conn2/DIO_0_7 - uSec Off
        w594 = bool[] [FALSE, FALSE, FALSE, FALSE, FALSE, FALSE, FALSE, FALSE]  # Conn2/DIO_0_7 In
        w593 = u16 0  # Conn2/DIO_0_7 - uSec On
        w592 = FALSE  # Conn2/DIO_0_7 - 75kHz
        # "Handswitch - Mono2 Coag"
        # "Handswitch - Mono2 Coag"
        # "Handswitch - Mono2 Coag"
        n44 = Bundle By Name(cluster=T4 {"Conn0/DIO_0_7 In"={"Conn0/DIO_0_7 - 75kHz"=FALSE, "Conn0/DIO_0_7 - uSec On"=0, "Conn0/DIO_0_7 In"=[FALSE, FALSE, FALSE, FALSE, FALSE, FALSE, FALSE, FALSE], "Conn0/DIO_0_7 - uSec Off"=0}, "Conn0/DIO_8_15 In"={"Conn0/DIO_8_15 - 75kHz"=FALSE, "Conn0/DIO_8_15 - uSec On"=0, "Conn0/DIO_8_15 In"=[FALSE, FALSE, FALSE, FALSE, FALSE, FALSE, FALSE, FALSE], "Conn0/DIO_8_15 - uSec Off"=0}} ("Conn0 DIOs In"), "Conn0/DIO_0_7 In.Conn0/DIO_0_7 - 75kHz"=w600, "Conn0/DIO_0_7 In.Conn0/DIO_0_7 - uSec On"=w601, "Conn0/DIO_0_7 In.Conn0/DIO_0_7 In"=w602, "Conn0/DIO_0_7 In.Conn0/DIO_0_7 - uSec Off"=w603, "Conn0/DIO_8_15 In.Conn0/DIO_8_15 - 75kHz"=w586, "Conn0/DIO_8_15 In.Conn0/DIO_8_15 - uSec On"=w585, "Conn0/DIO_8_15 In.Conn0/DIO_8_15 In"=w584, "Conn0/DIO_8_15 In.Conn0/DIO_8_15 - uSec Off"=w583) -> (w590:T4)
        n45 = Bundle By Name(cluster=T3 {"Conn1/DIO_0_7 In"={"Conn1/DIO_0_7 - 75kHz"=FALSE, "Conn1/DIO_0_7 - uSec On"=0, "Conn1/DIO_0_7 In"=[FALSE, FALSE, FALSE, FALSE, FALSE, FALSE, FALSE, FALSE], "Conn1/DIO_0_7 - uSec Off"=0}, "Conn1/DIO_8_15 In"={"Conn1/DIO_8_15 - 75kHz"=FALSE, "Conn1/DIO_8_15 - uSec On"=0, "Conn1/DIO_8_15 In"=[FALSE, FALSE, FALSE, FALSE, FALSE, FALSE, FALSE, FALSE], "Conn1/DIO_8_15 - uSec Off"=0}, "Conn1/DIO_16_23 In"={"Conn1/DIO_16_23 - 75kHz"=FALSE, "Conn1/DIO_16_23 - uSec On"=0, "Conn1/DIO_16_23 In"=[FALSE, FALSE, FALSE, FALSE, FALSE, FALSE, FALSE, FALSE], "Conn1/DIO_16_23 - uSec Off"=0}, "Conn1/DIO_24_31 In"={"Conn1/DIO_24_31 - 75kHz"=FALSE, "Conn1/DIO_24_31 - uSec On"=0, "Conn1/DIO_24_31 In"=[FALSE, FALSE, FALSE, FALSE, FALSE, FALSE, FALSE, FALSE], "Conn1/DIO_24_31 - uSec Off"=0}, "Conn1/DIO_32_39 In"={"Conn1/DIO_32_39 - 75kHz"=FALSE, "Conn1/DIO_32_39 - uSec On"=0, "Conn1/DIO_32_39 In"=[FALSE, FALSE, FALSE, FALSE, FALSE, FALSE, FALSE, FALSE], "Conn1/DIO_32_39 - uSec Off"=0}} ("Conn1 DIOs In"), "Conn1/DIO_0_7 In.Conn1/DIO_0_7 - 75kHz"=w596, "Conn1/DIO_0_7 In.Conn1/DIO_0_7 - uSec On"=w597, "Conn1/DIO_0_7 In.Conn1/DIO_0_7 In"=w598, "Conn1/DIO_0_7 In.Conn1/DIO_0_7 - uSec Off"=w599, "Conn1/DIO_8_15 In.Conn1/DIO_8_15 - 75kHz"=w582, "Conn1/DIO_8_15 In.Conn1/DIO_8_15 - uSec On"=w581, "Conn1/DIO_8_15 In.Conn1/DIO_8_15 In"=w580, "Conn1/DIO_8_15 In.Conn1/DIO_8_15 - uSec Off"=w579, "Conn1/DIO_16_23 In.Conn1/DIO_16_23 - 75kHz"=w578, "Conn1/DIO_16_23 In.Conn1/DIO_16_23 - uSec On"=w577, "Conn1/DIO_16_23 In.Conn1/DIO_16_23 In"=w576, "Conn1/DIO_16_23 In.Conn1/DIO_16_23 - uSec Off"=w575, "Conn1/DIO_24_31 In.Conn1/DIO_24_31 - 75kHz"=w574, "Conn1/DIO_24_31 In.Conn1/DIO_24_31 - uSec On"=w573, "Conn1/DIO_24_31 In.Conn1/DIO_24_31 In"=w572, "Conn1/DIO_24_31 In.Conn1/DIO_24_31 - uSec Off"=w571, "Conn1/DIO_32_39 In.Conn1/DIO_32_39 - 75kHz"=w570, "Conn1/DIO_32_39 In.Conn1/DIO_32_39 - uSec On"=w569, "Conn1/DIO_32_39 In.Conn1/DIO_32_39 In"=w568, "Conn1/DIO_32_39 In.Conn1/DIO_32_39 - uSec Off"=w567) -> (w604:T3)
        n46 = Bundle By Name(cluster=T2 {"Conn2/DIO_0_7 In"={"Conn2/DIO_0_7 - 75kHz"=FALSE, "Conn2/DIO_0_7 - uSec On"=0, "Conn2/DIO_0_7 In"=[FALSE, FALSE, FALSE, FALSE, FALSE, FALSE, FALSE, FALSE], "Conn2/DIO_0_7 - uSec Off"=0}, "Conn2/DIO_8_15 In"={"Conn2/DIO_8_15 - 75kHz"=FALSE, "Conn2/DIO_8_15 - uSec On"=0, "Conn2/DIO_8_15 In"=[FALSE, FALSE, FALSE, FALSE, FALSE, FALSE, FALSE, FALSE], "Conn2/DIO_8_15 - uSec Off"=0}, "Conn2/DIO_16_23 In"={"Conn2/DIO_16_23 - 75kHz"=FALSE, "Conn2/DIO_16_23 - uSec On"=0, "Conn2/DIO_16_23 In"=[FALSE, FALSE, FALSE, FALSE, FALSE, FALSE, FALSE, FALSE], "Conn2/DIO_16_23 - uSec Off"=0}, "Conn2/DIO_24_31 In"={"Conn2/DIO_24_31 - 75kHz"=FALSE, "Conn2/DIO_24_31 - uSec On"=0, "Conn2/DIO_24_31 In"=[FALSE, FALSE, FALSE, FALSE, FALSE, FALSE, FALSE, FALSE], "Conn2/DIO_24_31 - uSec Off"=0}, "Conn2/DIO_32_39 In"={"Conn2/DIO_32_39 - 75kHz"=FALSE, "Conn2/DIO_32_39 - uSec On"=0, "Conn2/DIO_32_39 In"=[FALSE, FALSE, FALSE, FALSE, FALSE, FALSE, FALSE, FALSE], "Conn2/DIO_32_39 - uSec Off"=0}} ("Conn2 DIOs In"), "Conn2/DIO_0_7 In.Conn2/DIO_0_7 - 75kHz"=w592, "Conn2/DIO_0_7 In.Conn2/DIO_0_7 - uSec On"=w593, "Conn2/DIO_0_7 In.Conn2/DIO_0_7 In"=w594, "Conn2/DIO_0_7 In.Conn2/DIO_0_7 - uSec Off"=w595, "Conn2/DIO_8_15 In.Conn2/DIO_8_15 - 75kHz"=w558, "Conn2/DIO_8_15 In.Conn2/DIO_8_15 - uSec On"=w557, "Conn2/DIO_8_15 In.Conn2/DIO_8_15 In"=w556, "Conn2/DIO_8_15 In.Conn2/DIO_8_15 - uSec Off"=w555, "Conn2/DIO_16_23 In.Conn2/DIO_16_23 - 75kHz"=w554, "Conn2/DIO_16_23 In.Conn2/DIO_16_23 - uSec On"=w553, "Conn2/DIO_16_23 In.Conn2/DIO_16_23 In"=w552, "Conn2/DIO_16_23 In.Conn2/DIO_16_23 - uSec Off"=w551, "Conn2/DIO_24_31 In.Conn2/DIO_24_31 - 75kHz"=w550, "Conn2/DIO_24_31 In.Conn2/DIO_24_31 - uSec On"=w549, "Conn2/DIO_24_31 In.Conn2/DIO_24_31 In"=w548, "Conn2/DIO_24_31 In.Conn2/DIO_24_31 - uSec Off"=w547, "Conn2/DIO_32_39 In.Conn2/DIO_32_39 - 75kHz"=w546, "Conn2/DIO_32_39 In.Conn2/DIO_32_39 - uSec On"=w545, "Conn2/DIO_32_39 In.Conn2/DIO_32_39 In"=w544, "Conn2/DIO_32_39 In.Conn2/DIO_32_39 - uSec Off"=w543) -> (w605:T2)
        n47 = Build Array(w566, w565, w564, w563, w562, w561, w560, w559) -> (w606:i16[])
        n48 = xnode "Read/Write Control"("FPGA VI Reference In"=w587, "Conn0 DIOs In"=w590, "Conn1 DIOs In"=w604, "Conn2 DIOs In"=w605, "Connector0/AO0_7"=w606) -> ("FPGA VI Reference Out"=w588:refnum<k20>)  [unwired: 1 in, 1 out]
      }
      frame "Switch to Triverse Mode" {
        w611 = u16 0  # Conn2/DIO_32_39 - uSec Off
        w612 = bool[] [FALSE, FALSE, FALSE, FALSE, FALSE, FALSE, FALSE, FALSE]  # Conn2/DIO_32_39 In
        w613 = u16 0  # Conn2/DIO_32_39 - uSec On
        w614 = FALSE  # Conn2/DIO_32_39 - 75kHz
        w615 = u16 0  # Conn2/DIO_24_31 - uSec Off
        w616 = bool[] [FALSE, FALSE, FALSE, FALSE, FALSE, FALSE, FALSE, FALSE]  # Conn2/DIO_24_31 In
        w617 = u16 0  # Conn2/DIO_24_31 - uSec On
        w618 = FALSE  # Conn2/DIO_24_31 - 75kHz
        w619 = u16 0  # Conn2/DIO_16_23 - uSec Off
        w620 = bool[] [FALSE, FALSE, FALSE, FALSE, FALSE, FALSE, FALSE, FALSE]  # Conn2/DIO_16_23 In
        w621 = u16 0  # Conn2/DIO_16_23 - uSec On
        w622 = FALSE  # Conn2/DIO_16_23 - 75kHz
        w623 = u16 6  # Conn2/DIO_8_15 - uSec Off
        w624 = bool[] [FALSE, TRUE, TRUE, FALSE, FALSE, FALSE, FALSE, FALSE]  # Conn2/DIO_8_15 In
        w625 = u16 7  # Conn2/DIO_8_15 - uSec On
        w626 = TRUE  # Conn2/DIO_8_15 - 75kHz
        w627 = i16 0  # Connector0/AO7
        w628 = i16 0  # Connector0/AO6
        w629 = i16 0  # Connector0/AO5
        w630 = i16 0  # Connector0/AO4
        w631 = i16 0  # Connector0/AO3
        w632 = i16 0  # Connector0/AO2
        w633 = i16 0  # Connector0/AO1
        w634 = i16 0  # Connector0/AO0
        w635 = u16 0  # Conn1/DIO_32_39 - uSec Off
        w636 = bool[] [FALSE, FALSE, FALSE, FALSE, FALSE, FALSE, FALSE, FALSE]  # Conn1/DIO_32_39 In
        w637 = u16 0  # Conn1/DIO_32_39 - uSec On
        w638 = FALSE  # Conn1/DIO_32_39 - 75kHz
        w639 = u16 0  # Conn1/DIO_24_31 - uSec Off
        w640 = bool[] [FALSE, FALSE, FALSE, FALSE, FALSE, FALSE, FALSE, FALSE]  # Conn1/DIO_24_31 In
        w641 = u16 0  # Conn1/DIO_24_31 - uSec On
        w642 = FALSE  # Conn1/DIO_24_31 - 75kHz
        w643 = u16 6  # Conn1/DIO_16_23 - uSec Off
        w644 = bool[] [FALSE, TRUE, FALSE, FALSE, FALSE, FALSE, FALSE, FALSE]  # Conn1/DIO_16_23 In
        w645 = u16 7  # Conn1/DIO_16_23 - uSec On
        w646 = TRUE  # Conn1/DIO_16_23 - 75kHz
        w647 = u16 0  # Conn1/DIO_8_15 - uSec Off
        w648 = bool[] [FALSE, FALSE, FALSE, FALSE, FALSE, FALSE, FALSE, FALSE]  # Conn1/DIO_8_15 In
        w649 = u16 0  # Conn1/DIO_8_15 - uSec On
        w650 = FALSE  # Conn1/DIO_8_15 - 75kHz
        w651 = u16 0  # Conn0/DIO_8_15 - uSec Off
        w652 = bool[] [FALSE, FALSE, FALSE, FALSE, FALSE, FALSE, FALSE, FALSE]  # Conn0/DIO_8_15 In
        w653 = u16 0  # Conn0/DIO_8_15 - uSec On
        w654 = FALSE  # Conn0/DIO_8_15 - 75kHz
        w671 = u16 0  # Conn0/DIO_0_7 - uSec Off
        w670 = bool[] [FALSE, FALSE, FALSE, FALSE, FALSE, FALSE, FALSE, FALSE]  # Conn0/DIO_0_7 In
        w669 = u16 0  # Conn0/DIO_0_7 - uSec On
        w668 = FALSE  # Conn0/DIO_0_7 - 75kHz
        w667 = u16 0  # Conn1/DIO_0_7 - uSec Off
        w666 = bool[] [FALSE, FALSE, FALSE, FALSE, FALSE, FALSE, FALSE, FALSE]  # Conn1/DIO_0_7 In
        w665 = u16 0  # Conn1/DIO_0_7 - uSec On
        w664 = FALSE  # Conn1/DIO_0_7 - 75kHz
        w663 = u16 0  # Conn2/DIO_0_7 - uSec Off
        w662 = bool[] [FALSE, FALSE, FALSE, FALSE, FALSE, FALSE, FALSE, FALSE]  # Conn2/DIO_0_7 In
        w661 = u16 0  # Conn2/DIO_0_7 - uSec On
        w660 = FALSE  # Conn2/DIO_0_7 - 75kHz
        # "Switch to Triverse Mode"
        # "Switch to Triverse Mode"
        # "Switch to Triverse Mode"
        n49 = Bundle By Name(cluster=T4 {"Conn0/DIO_0_7 In"={"Conn0/DIO_0_7 - 75kHz"=FALSE, "Conn0/DIO_0_7 - uSec On"=0, "Conn0/DIO_0_7 In"=[FALSE, FALSE, FALSE, FALSE, FALSE, FALSE, FALSE, FALSE], "Conn0/DIO_0_7 - uSec Off"=0}, "Conn0/DIO_8_15 In"={"Conn0/DIO_8_15 - 75kHz"=FALSE, "Conn0/DIO_8_15 - uSec On"=0, "Conn0/DIO_8_15 In"=[FALSE, FALSE, FALSE, FALSE, FALSE, FALSE, FALSE, FALSE], "Conn0/DIO_8_15 - uSec Off"=0}} ("Conn0 DIOs In"), "Conn0/DIO_0_7 In.Conn0/DIO_0_7 - 75kHz"=w668, "Conn0/DIO_0_7 In.Conn0/DIO_0_7 - uSec On"=w669, "Conn0/DIO_0_7 In.Conn0/DIO_0_7 In"=w670, "Conn0/DIO_0_7 In.Conn0/DIO_0_7 - uSec Off"=w671, "Conn0/DIO_8_15 In.Conn0/DIO_8_15 - 75kHz"=w654, "Conn0/DIO_8_15 In.Conn0/DIO_8_15 - uSec On"=w653, "Conn0/DIO_8_15 In.Conn0/DIO_8_15 In"=w652, "Conn0/DIO_8_15 In.Conn0/DIO_8_15 - uSec Off"=w651) -> (w658:T4)
        n50 = Bundle By Name(cluster=T3 {"Conn1/DIO_0_7 In"={"Conn1/DIO_0_7 - 75kHz"=FALSE, "Conn1/DIO_0_7 - uSec On"=0, "Conn1/DIO_0_7 In"=[FALSE, FALSE, FALSE, FALSE, FALSE, FALSE, FALSE, FALSE], "Conn1/DIO_0_7 - uSec Off"=0}, "Conn1/DIO_8_15 In"={"Conn1/DIO_8_15 - 75kHz"=FALSE, "Conn1/DIO_8_15 - uSec On"=0, "Conn1/DIO_8_15 In"=[FALSE, FALSE, FALSE, FALSE, FALSE, FALSE, FALSE, FALSE], "Conn1/DIO_8_15 - uSec Off"=0}, "Conn1/DIO_16_23 In"={"Conn1/DIO_16_23 - 75kHz"=FALSE, "Conn1/DIO_16_23 - uSec On"=0, "Conn1/DIO_16_23 In"=[FALSE, FALSE, FALSE, FALSE, FALSE, FALSE, FALSE, FALSE], "Conn1/DIO_16_23 - uSec Off"=0}, "Conn1/DIO_24_31 In"={"Conn1/DIO_24_31 - 75kHz"=FALSE, "Conn1/DIO_24_31 - uSec On"=0, "Conn1/DIO_24_31 In"=[FALSE, FALSE, FALSE, FALSE, FALSE, FALSE, FALSE, FALSE], "Conn1/DIO_24_31 - uSec Off"=0}, "Conn1/DIO_32_39 In"={"Conn1/DIO_32_39 - 75kHz"=FALSE, "Conn1/DIO_32_39 - uSec On"=0, "Conn1/DIO_32_39 In"=[FALSE, FALSE, FALSE, FALSE, FALSE, FALSE, FALSE, FALSE], "Conn1/DIO_32_39 - uSec Off"=0}} ("Conn1 DIOs In"), "Conn1/DIO_0_7 In.Conn1/DIO_0_7 - 75kHz"=w664, "Conn1/DIO_0_7 In.Conn1/DIO_0_7 - uSec On"=w665, "Conn1/DIO_0_7 In.Conn1/DIO_0_7 In"=w666, "Conn1/DIO_0_7 In.Conn1/DIO_0_7 - uSec Off"=w667, "Conn1/DIO_8_15 In.Conn1/DIO_8_15 - 75kHz"=w650, "Conn1/DIO_8_15 In.Conn1/DIO_8_15 - uSec On"=w649, "Conn1/DIO_8_15 In.Conn1/DIO_8_15 In"=w648, "Conn1/DIO_8_15 In.Conn1/DIO_8_15 - uSec Off"=w647, "Conn1/DIO_16_23 In.Conn1/DIO_16_23 - 75kHz"=w646, "Conn1/DIO_16_23 In.Conn1/DIO_16_23 - uSec On"=w645, "Conn1/DIO_16_23 In.Conn1/DIO_16_23 In"=w644, "Conn1/DIO_16_23 In.Conn1/DIO_16_23 - uSec Off"=w643, "Conn1/DIO_24_31 In.Conn1/DIO_24_31 - 75kHz"=w642, "Conn1/DIO_24_31 In.Conn1/DIO_24_31 - uSec On"=w641, "Conn1/DIO_24_31 In.Conn1/DIO_24_31 In"=w640, "Conn1/DIO_24_31 In.Conn1/DIO_24_31 - uSec Off"=w639, "Conn1/DIO_32_39 In.Conn1/DIO_32_39 - 75kHz"=w638, "Conn1/DIO_32_39 In.Conn1/DIO_32_39 - uSec On"=w637, "Conn1/DIO_32_39 In.Conn1/DIO_32_39 In"=w636, "Conn1/DIO_32_39 In.Conn1/DIO_32_39 - uSec Off"=w635) -> (w672:T3)
        n51 = Bundle By Name(cluster=T2 {"Conn2/DIO_0_7 In"={"Conn2/DIO_0_7 - 75kHz"=FALSE, "Conn2/DIO_0_7 - uSec On"=0, "Conn2/DIO_0_7 In"=[FALSE, FALSE, FALSE, FALSE, FALSE, FALSE, FALSE, FALSE], "Conn2/DIO_0_7 - uSec Off"=0}, "Conn2/DIO_8_15 In"={"Conn2/DIO_8_15 - 75kHz"=FALSE, "Conn2/DIO_8_15 - uSec On"=0, "Conn2/DIO_8_15 In"=[FALSE, FALSE, FALSE, FALSE, FALSE, FALSE, FALSE, FALSE], "Conn2/DIO_8_15 - uSec Off"=0}, "Conn2/DIO_16_23 In"={"Conn2/DIO_16_23 - 75kHz"=FALSE, "Conn2/DIO_16_23 - uSec On"=0, "Conn2/DIO_16_23 In"=[FALSE, FALSE, FALSE, FALSE, FALSE, FALSE, FALSE, FALSE], "Conn2/DIO_16_23 - uSec Off"=0}, "Conn2/DIO_24_31 In"={"Conn2/DIO_24_31 - 75kHz"=FALSE, "Conn2/DIO_24_31 - uSec On"=0, "Conn2/DIO_24_31 In"=[FALSE, FALSE, FALSE, FALSE, FALSE, FALSE, FALSE, FALSE], "Conn2/DIO_24_31 - uSec Off"=0}, "Conn2/DIO_32_39 In"={"Conn2/DIO_32_39 - 75kHz"=FALSE, "Conn2/DIO_32_39 - uSec On"=0, "Conn2/DIO_32_39 In"=[FALSE, FALSE, FALSE, FALSE, FALSE, FALSE, FALSE, FALSE], "Conn2/DIO_32_39 - uSec Off"=0}} ("Conn2 DIOs In"), "Conn2/DIO_0_7 In.Conn2/DIO_0_7 - 75kHz"=w660, "Conn2/DIO_0_7 In.Conn2/DIO_0_7 - uSec On"=w661, "Conn2/DIO_0_7 In.Conn2/DIO_0_7 In"=w662, "Conn2/DIO_0_7 In.Conn2/DIO_0_7 - uSec Off"=w663, "Conn2/DIO_8_15 In.Conn2/DIO_8_15 - 75kHz"=w626, "Conn2/DIO_8_15 In.Conn2/DIO_8_15 - uSec On"=w625, "Conn2/DIO_8_15 In.Conn2/DIO_8_15 In"=w624, "Conn2/DIO_8_15 In.Conn2/DIO_8_15 - uSec Off"=w623, "Conn2/DIO_16_23 In.Conn2/DIO_16_23 - 75kHz"=w622, "Conn2/DIO_16_23 In.Conn2/DIO_16_23 - uSec On"=w621, "Conn2/DIO_16_23 In.Conn2/DIO_16_23 In"=w620, "Conn2/DIO_16_23 In.Conn2/DIO_16_23 - uSec Off"=w619, "Conn2/DIO_24_31 In.Conn2/DIO_24_31 - 75kHz"=w618, "Conn2/DIO_24_31 In.Conn2/DIO_24_31 - uSec On"=w617, "Conn2/DIO_24_31 In.Conn2/DIO_24_31 In"=w616, "Conn2/DIO_24_31 In.Conn2/DIO_24_31 - uSec Off"=w615, "Conn2/DIO_32_39 In.Conn2/DIO_32_39 - 75kHz"=w614, "Conn2/DIO_32_39 In.Conn2/DIO_32_39 - uSec On"=w613, "Conn2/DIO_32_39 In.Conn2/DIO_32_39 In"=w612, "Conn2/DIO_32_39 In.Conn2/DIO_32_39 - uSec Off"=w611) -> (w673:T2)
        n52 = Build Array(w634, w633, w632, w631, w630, w629, w628, w627) -> (w674:i16[])
        n53 = xnode "Read/Write Control"("FPGA VI Reference In"=w655, "Conn0 DIOs In"=w658, "Conn1 DIOs In"=w672, "Conn2 DIOs In"=w673, "Connector0/AO0_7"=w674) -> ("FPGA VI Reference Out"=w656:refnum<k20>)  [unwired: 1 in, 1 out]
      }
      frame "Switch to Mono2 - 2 button Mode" {
        w677 = u16 0  # Conn2/DIO_32_39 - uSec Off
        w678 = bool[] [FALSE, FALSE, FALSE, FALSE, FALSE, FALSE, FALSE, FALSE]  # Conn2/DIO_32_39 In
        w679 = u16 0  # Conn2/DIO_32_39 - uSec On
        w680 = FALSE  # Conn2/DIO_32_39 - 75kHz
        w681 = u16 0  # Conn2/DIO_24_31 - uSec Off
        w682 = bool[] [FALSE, FALSE, FALSE, FALSE, FALSE, FALSE, FALSE, FALSE]  # Conn2/DIO_24_31 In
        w683 = u16 0  # Conn2/DIO_24_31 - uSec On
        w684 = FALSE  # Conn2/DIO_24_31 - 75kHz
        w685 = u16 0  # Conn2/DIO_16_23 - uSec Off
        w686 = bool[] [FALSE, FALSE, FALSE, FALSE, FALSE, FALSE, FALSE, FALSE]  # Conn2/DIO_16_23 In
        w687 = u16 0  # Conn2/DIO_16_23 - uSec On
        w688 = FALSE  # Conn2/DIO_16_23 - 75kHz
        w689 = u16 0  # Conn2/DIO_8_15 - uSec Off
        w690 = bool[] [FALSE, FALSE, FALSE, FALSE, FALSE, FALSE, FALSE, FALSE]  # Conn2/DIO_8_15 In
        w691 = u16 0  # Conn2/DIO_8_15 - uSec On
        w692 = FALSE  # Conn2/DIO_8_15 - 75kHz
        w693 = i16 0  # Connector0/AO7
        w694 = i16 0  # Connector0/AO6
        w695 = i16 0  # Connector0/AO5
        w696 = i16 0  # Connector0/AO4
        w697 = i16 0  # Connector0/AO3
        w698 = i16 0  # Connector0/AO2
        w699 = i16 0  # Connector0/AO1
        w700 = i16 0  # Connector0/AO0
        w701 = u16 0  # Conn1/DIO_32_39 - uSec Off
        w702 = bool[] [FALSE, FALSE, FALSE, FALSE, FALSE, FALSE, FALSE, FALSE]  # Conn1/DIO_32_39 In
        w703 = u16 0  # Conn1/DIO_32_39 - uSec On
        w704 = FALSE  # Conn1/DIO_32_39 - 75kHz
        w705 = u16 0  # Conn1/DIO_24_31 - uSec Off
        w706 = bool[] [FALSE, FALSE, FALSE, FALSE, FALSE, FALSE, FALSE, FALSE]  # Conn1/DIO_24_31 In
        w707 = u16 0  # Conn1/DIO_24_31 - uSec On
        w708 = FALSE  # Conn1/DIO_24_31 - 75kHz
        w709 = u16 6  # Conn1/DIO_16_23 - uSec Off
        w710 = bool[] [FALSE, TRUE, FALSE, FALSE, FALSE, FALSE, FALSE, FALSE]  # Conn1/DIO_16_23 In
        w711 = u16 7  # Conn1/DIO_16_23 - uSec On
        w712 = TRUE  # Conn1/DIO_16_23 - 75kHz
        w713 = u16 0  # Conn1/DIO_8_15 - uSec Off
        w714 = bool[] [FALSE, FALSE, FALSE, FALSE, FALSE, FALSE, FALSE, FALSE]  # Conn1/DIO_8_15 In
        w715 = u16 0  # Conn1/DIO_8_15 - uSec On
        w716 = FALSE  # Conn1/DIO_8_15 - 75kHz
        w717 = u16 0  # Conn0/DIO_8_15 - uSec Off
        w718 = bool[] [FALSE, FALSE, FALSE, FALSE, FALSE, FALSE, FALSE, FALSE]  # Conn0/DIO_8_15 In
        w719 = u16 0  # Conn0/DIO_8_15 - uSec On
        w720 = FALSE  # Conn0/DIO_8_15 - 75kHz
        w737 = u16 0  # Conn0/DIO_0_7 - uSec Off
        w736 = bool[] [FALSE, FALSE, FALSE, FALSE, FALSE, FALSE, FALSE, FALSE]  # Conn0/DIO_0_7 In
        w735 = u16 0  # Conn0/DIO_0_7 - uSec On
        w734 = FALSE  # Conn0/DIO_0_7 - 75kHz
        w733 = u16 0  # Conn1/DIO_0_7 - uSec Off
        w732 = bool[] [FALSE, FALSE, FALSE, FALSE, FALSE, FALSE, FALSE, FALSE]  # Conn1/DIO_0_7 In
        w731 = u16 0  # Conn1/DIO_0_7 - uSec On
        w730 = FALSE  # Conn1/DIO_0_7 - 75kHz
        w729 = u16 0  # Conn2/DIO_0_7 - uSec Off
        w728 = bool[] [FALSE, FALSE, FALSE, FALSE, FALSE, FALSE, FALSE, FALSE]  # Conn2/DIO_0_7 In
        w727 = u16 0  # Conn2/DIO_0_7 - uSec On
        w726 = FALSE  # Conn2/DIO_0_7 - 75kHz
        # "Switch to Mono2 - 2 button Mode"
        # "Switch to Mono2 - 2 button Mode"
        # "Switch to Mono2 - 2 button Mode"
        n54 = Bundle By Name(cluster=T4 {"Conn0/DIO_0_7 In"={"Conn0/DIO_0_7 - 75kHz"=FALSE, "Conn0/DIO_0_7 - uSec On"=0, "Conn0/DIO_0_7 In"=[FALSE, FALSE, FALSE, FALSE, FALSE, FALSE, FALSE, FALSE], "Conn0/DIO_0_7 - uSec Off"=0}, "Conn0/DIO_8_15 In"={"Conn0/DIO_8_15 - 75kHz"=FALSE, "Conn0/DIO_8_15 - uSec On"=0, "Conn0/DIO_8_15 In"=[FALSE, FALSE, FALSE, FALSE, FALSE, FALSE, FALSE, FALSE], "Conn0/DIO_8_15 - uSec Off"=0}} ("Conn0 DIOs In"), "Conn0/DIO_0_7 In.Conn0/DIO_0_7 - 75kHz"=w734, "Conn0/DIO_0_7 In.Conn0/DIO_0_7 - uSec On"=w735, "Conn0/DIO_0_7 In.Conn0/DIO_0_7 In"=w736, "Conn0/DIO_0_7 In.Conn0/DIO_0_7 - uSec Off"=w737, "Conn0/DIO_8_15 In.Conn0/DIO_8_15 - 75kHz"=w720, "Conn0/DIO_8_15 In.Conn0/DIO_8_15 - uSec On"=w719, "Conn0/DIO_8_15 In.Conn0/DIO_8_15 In"=w718, "Conn0/DIO_8_15 In.Conn0/DIO_8_15 - uSec Off"=w717) -> (w724:T4)
        n55 = Bundle By Name(cluster=T3 {"Conn1/DIO_0_7 In"={"Conn1/DIO_0_7 - 75kHz"=FALSE, "Conn1/DIO_0_7 - uSec On"=0, "Conn1/DIO_0_7 In"=[FALSE, FALSE, FALSE, FALSE, FALSE, FALSE, FALSE, FALSE], "Conn1/DIO_0_7 - uSec Off"=0}, "Conn1/DIO_8_15 In"={"Conn1/DIO_8_15 - 75kHz"=FALSE, "Conn1/DIO_8_15 - uSec On"=0, "Conn1/DIO_8_15 In"=[FALSE, FALSE, FALSE, FALSE, FALSE, FALSE, FALSE, FALSE], "Conn1/DIO_8_15 - uSec Off"=0}, "Conn1/DIO_16_23 In"={"Conn1/DIO_16_23 - 75kHz"=FALSE, "Conn1/DIO_16_23 - uSec On"=0, "Conn1/DIO_16_23 In"=[FALSE, FALSE, FALSE, FALSE, FALSE, FALSE, FALSE, FALSE], "Conn1/DIO_16_23 - uSec Off"=0}, "Conn1/DIO_24_31 In"={"Conn1/DIO_24_31 - 75kHz"=FALSE, "Conn1/DIO_24_31 - uSec On"=0, "Conn1/DIO_24_31 In"=[FALSE, FALSE, FALSE, FALSE, FALSE, FALSE, FALSE, FALSE], "Conn1/DIO_24_31 - uSec Off"=0}, "Conn1/DIO_32_39 In"={"Conn1/DIO_32_39 - 75kHz"=FALSE, "Conn1/DIO_32_39 - uSec On"=0, "Conn1/DIO_32_39 In"=[FALSE, FALSE, FALSE, FALSE, FALSE, FALSE, FALSE, FALSE], "Conn1/DIO_32_39 - uSec Off"=0}} ("Conn1 DIOs In"), "Conn1/DIO_0_7 In.Conn1/DIO_0_7 - 75kHz"=w730, "Conn1/DIO_0_7 In.Conn1/DIO_0_7 - uSec On"=w731, "Conn1/DIO_0_7 In.Conn1/DIO_0_7 In"=w732, "Conn1/DIO_0_7 In.Conn1/DIO_0_7 - uSec Off"=w733, "Conn1/DIO_8_15 In.Conn1/DIO_8_15 - 75kHz"=w716, "Conn1/DIO_8_15 In.Conn1/DIO_8_15 - uSec On"=w715, "Conn1/DIO_8_15 In.Conn1/DIO_8_15 In"=w714, "Conn1/DIO_8_15 In.Conn1/DIO_8_15 - uSec Off"=w713, "Conn1/DIO_16_23 In.Conn1/DIO_16_23 - 75kHz"=w712, "Conn1/DIO_16_23 In.Conn1/DIO_16_23 - uSec On"=w711, "Conn1/DIO_16_23 In.Conn1/DIO_16_23 In"=w710, "Conn1/DIO_16_23 In.Conn1/DIO_16_23 - uSec Off"=w709, "Conn1/DIO_24_31 In.Conn1/DIO_24_31 - 75kHz"=w708, "Conn1/DIO_24_31 In.Conn1/DIO_24_31 - uSec On"=w707, "Conn1/DIO_24_31 In.Conn1/DIO_24_31 In"=w706, "Conn1/DIO_24_31 In.Conn1/DIO_24_31 - uSec Off"=w705, "Conn1/DIO_32_39 In.Conn1/DIO_32_39 - 75kHz"=w704, "Conn1/DIO_32_39 In.Conn1/DIO_32_39 - uSec On"=w703, "Conn1/DIO_32_39 In.Conn1/DIO_32_39 In"=w702, "Conn1/DIO_32_39 In.Conn1/DIO_32_39 - uSec Off"=w701) -> (w738:T3)
        n56 = Bundle By Name(cluster=T2 {"Conn2/DIO_0_7 In"={"Conn2/DIO_0_7 - 75kHz"=FALSE, "Conn2/DIO_0_7 - uSec On"=0, "Conn2/DIO_0_7 In"=[FALSE, FALSE, FALSE, FALSE, FALSE, FALSE, FALSE, FALSE], "Conn2/DIO_0_7 - uSec Off"=0}, "Conn2/DIO_8_15 In"={"Conn2/DIO_8_15 - 75kHz"=FALSE, "Conn2/DIO_8_15 - uSec On"=0, "Conn2/DIO_8_15 In"=[FALSE, FALSE, FALSE, FALSE, FALSE, FALSE, FALSE, FALSE], "Conn2/DIO_8_15 - uSec Off"=0}, "Conn2/DIO_16_23 In"={"Conn2/DIO_16_23 - 75kHz"=FALSE, "Conn2/DIO_16_23 - uSec On"=0, "Conn2/DIO_16_23 In"=[FALSE, FALSE, FALSE, FALSE, FALSE, FALSE, FALSE, FALSE], "Conn2/DIO_16_23 - uSec Off"=0}, "Conn2/DIO_24_31 In"={"Conn2/DIO_24_31 - 75kHz"=FALSE, "Conn2/DIO_24_31 - uSec On"=0, "Conn2/DIO_24_31 In"=[FALSE, FALSE, FALSE, FALSE, FALSE, FALSE, FALSE, FALSE], "Conn2/DIO_24_31 - uSec Off"=0}, "Conn2/DIO_32_39 In"={"Conn2/DIO_32_39 - 75kHz"=FALSE, "Conn2/DIO_32_39 - uSec On"=0, "Conn2/DIO_32_39 In"=[FALSE, FALSE, FALSE, FALSE, FALSE, FALSE, FALSE, FALSE], "Conn2/DIO_32_39 - uSec Off"=0}} ("Conn2 DIOs In"), "Conn2/DIO_0_7 In.Conn2/DIO_0_7 - 75kHz"=w726, "Conn2/DIO_0_7 In.Conn2/DIO_0_7 - uSec On"=w727, "Conn2/DIO_0_7 In.Conn2/DIO_0_7 In"=w728, "Conn2/DIO_0_7 In.Conn2/DIO_0_7 - uSec Off"=w729, "Conn2/DIO_8_15 In.Conn2/DIO_8_15 - 75kHz"=w692, "Conn2/DIO_8_15 In.Conn2/DIO_8_15 - uSec On"=w691, "Conn2/DIO_8_15 In.Conn2/DIO_8_15 In"=w690, "Conn2/DIO_8_15 In.Conn2/DIO_8_15 - uSec Off"=w689, "Conn2/DIO_16_23 In.Conn2/DIO_16_23 - 75kHz"=w688, "Conn2/DIO_16_23 In.Conn2/DIO_16_23 - uSec On"=w687, "Conn2/DIO_16_23 In.Conn2/DIO_16_23 In"=w686, "Conn2/DIO_16_23 In.Conn2/DIO_16_23 - uSec Off"=w685, "Conn2/DIO_24_31 In.Conn2/DIO_24_31 - 75kHz"=w684, "Conn2/DIO_24_31 In.Conn2/DIO_24_31 - uSec On"=w683, "Conn2/DIO_24_31 In.Conn2/DIO_24_31 In"=w682, "Conn2/DIO_24_31 In.Conn2/DIO_24_31 - uSec Off"=w681, "Conn2/DIO_32_39 In.Conn2/DIO_32_39 - 75kHz"=w680, "Conn2/DIO_32_39 In.Conn2/DIO_32_39 - uSec On"=w679, "Conn2/DIO_32_39 In.Conn2/DIO_32_39 In"=w678, "Conn2/DIO_32_39 In.Conn2/DIO_32_39 - uSec Off"=w677) -> (w739:T2)
        n57 = Build Array(w700, w699, w698, w697, w696, w695, w694, w693) -> (w740:i16[])
        n58 = One Button Dialog(message="Unplug & Re-plug connector\nto exit Triverse mode") -> ()  [unwired: 1 in, 1 out]
        n59 = xnode "Read/Write Control"("FPGA VI Reference In"=w721, "Conn0 DIOs In"=w724, "Conn1 DIOs In"=w738, "Conn2 DIOs In"=w739, "Connector0/AO0_7"=w740) -> ("FPGA VI Reference Out"=w722:refnum<k20>)  [unwired: 1 in, 1 out]
      }
      frame "Triverse Power 1" {
        w745 = FALSE  # Conn2/DIO_7
        w749 = FALSE  # Conn2/DIO_6
        w741 = TRUE  # Conn2/DIO_5
        w742 = TRUE  # Conn2/DIO_4
        w743 = TRUE  # Conn2/DIO_3
        w748 = TRUE  # Conn2/DIO_2
        w747 = FALSE  # Conn2/DIO_1
        w746 = FALSE  # Conn2/DIO_0
        w751 = u16 0  # Conn2/DIO_32_39 - uSec Off
        w752 = bool[] [FALSE, FALSE, FALSE, FALSE, FALSE, FALSE, FALSE, FALSE]  # Conn2/DIO_32_39 In
        w753 = u16 0  # Conn2/DIO_32_39 - uSec On
        w754 = FALSE  # Conn2/DIO_32_39 - 75kHz
        w755 = u16 0  # Conn2/DIO_24_31 - uSec Off
        w756 = bool[] [FALSE, FALSE, FALSE, FALSE, FALSE, FALSE, FALSE, FALSE]  # Conn2/DIO_24_31 In
        w757 = u16 0  # Conn2/DIO_24_31 - uSec On
        w758 = FALSE  # Conn2/DIO_24_31 - 75kHz
        w759 = u16 0  # Conn2/DIO_16_23 - uSec Off
        w760 = bool[] [FALSE, FALSE, FALSE, FALSE, FALSE, FALSE, FALSE, FALSE]  # Conn2/DIO_16_23 In
        w761 = u16 0  # Conn2/DIO_16_23 - uSec On
        w762 = FALSE  # Conn2/DIO_16_23 - 75kHz
        w763 = u16 6  # Conn2/DIO_8_15 - uSec Off
        w764 = bool[] [FALSE, TRUE, FALSE, FALSE, FALSE, FALSE, FALSE, FALSE]  # Conn2/DIO_8_15 In
        w765 = u16 7  # Conn2/DIO_8_15 - uSec On
        w766 = TRUE  # Conn2/DIO_8_15 - 75kHz
        w767 = i16 0  # Connector0/AO7
        w768 = i16 0  # Connector0/AO6
        w769 = i16 0  # Connector0/AO5
        w770 = i16 0  # Connector0/AO4
        w771 = i16 0  # Connector0/AO3
        w772 = i16 0  # Connector0/AO2
        w773 = i16 0  # Connector0/AO1
        w774 = i16 0  # Connector0/AO0
        w775 = u16 0  # Conn1/DIO_32_39 - uSec Off
        w776 = bool[] [FALSE, FALSE, FALSE, FALSE, FALSE, FALSE, FALSE, FALSE]  # Conn1/DIO_32_39 In
        w777 = u16 0  # Conn1/DIO_32_39 - uSec On
        w778 = FALSE  # Conn1/DIO_32_39 - 75kHz
        w779 = u16 0  # Conn1/DIO_24_31 - uSec Off
        w780 = bool[] [FALSE, FALSE, FALSE, FALSE, FALSE, FALSE, FALSE, FALSE]  # Conn1/DIO_24_31 In
        w781 = u16 0  # Conn1/DIO_24_31 - uSec On
        w782 = FALSE  # Conn1/DIO_24_31 - 75kHz
        w783 = u16 6  # Conn1/DIO_16_23 - uSec Off
        w784 = bool[] [FALSE, TRUE, FALSE, FALSE, FALSE, FALSE, FALSE, FALSE]  # Conn1/DIO_16_23 In
        w785 = u16 7  # Conn1/DIO_16_23 - uSec On
        w786 = TRUE  # Conn1/DIO_16_23 - 75kHz
        w787 = u16 6  # Conn1/DIO_8_15 - uSec Off
        w788 = bool[] [FALSE, FALSE, FALSE, TRUE, FALSE, FALSE, FALSE, FALSE]  # Conn1/DIO_8_15 In
        w789 = u16 7  # Conn1/DIO_8_15 - uSec On
        w790 = TRUE  # Conn1/DIO_8_15 - 75kHz
        w791 = u16 0  # Conn0/DIO_8_15 - uSec Off
        w792 = bool[] [FALSE, FALSE, FALSE, FALSE, FALSE, FALSE, FALSE, FALSE]  # Conn0/DIO_8_15 In
        w793 = u16 0  # Conn0/DIO_8_15 - uSec On
        w794 = FALSE  # Conn0/DIO_8_15 - 75kHz
        w810 = u16 0  # Conn0/DIO_0_7 - uSec Off
        w809 = bool[] [FALSE, FALSE, FALSE, FALSE, FALSE, FALSE, FALSE, FALSE]  # Conn0/DIO_0_7 In
        w808 = u16 0  # Conn0/DIO_0_7 - uSec On
        w807 = FALSE  # Conn0/DIO_0_7 - 75kHz
        w806 = u16 6  # Conn1/DIO_0_7 - uSec Off
        w805 = bool[] [FALSE, TRUE, TRUE, TRUE, TRUE, FALSE, FALSE, TRUE]  # Conn1/DIO_0_7 In
        w804 = u16 7  # Conn1/DIO_0_7 - uSec On
        w803 = TRUE  # Conn1/DIO_0_7 - 75kHz
        w802 = u16 6  # Conn2/DIO_0_7 - uSec Off
        w801 = u16 7  # Conn2/DIO_0_7 - uSec On
        w800 = TRUE  # Conn2/DIO_0_7 - 75kHz
        # "Triverse Power 1"
        # "Triverse Power 1"
        # "Triverse Power 1"
        n60 = Build Array(w746, w747, w748, w743, w742, w741, w749, w745) -> (w744:bool[])
        n61 = Bundle By Name(cluster=T4 {"Conn0/DIO_0_7 In"={"Conn0/DIO_0_7 - 75kHz"=FALSE, "Conn0/DIO_0_7 - uSec On"=0, "Conn0/DIO_0_7 In"=[FALSE, FALSE, FALSE, FALSE, FALSE, FALSE, FALSE, FALSE], "Conn0/DIO_0_7 - uSec Off"=0}, "Conn0/DIO_8_15 In"={"Conn0/DIO_8_15 - 75kHz"=FALSE, "Conn0/DIO_8_15 - uSec On"=0, "Conn0/DIO_8_15 In"=[FALSE, FALSE, FALSE, FALSE, FALSE, FALSE, FALSE, FALSE], "Conn0/DIO_8_15 - uSec Off"=0}} ("Conn0 DIOs In"), "Conn0/DIO_0_7 In.Conn0/DIO_0_7 - 75kHz"=w807, "Conn0/DIO_0_7 In.Conn0/DIO_0_7 - uSec On"=w808, "Conn0/DIO_0_7 In.Conn0/DIO_0_7 In"=w809, "Conn0/DIO_0_7 In.Conn0/DIO_0_7 - uSec Off"=w810, "Conn0/DIO_8_15 In.Conn0/DIO_8_15 - 75kHz"=w794, "Conn0/DIO_8_15 In.Conn0/DIO_8_15 - uSec On"=w793, "Conn0/DIO_8_15 In.Conn0/DIO_8_15 In"=w792, "Conn0/DIO_8_15 In.Conn0/DIO_8_15 - uSec Off"=w791) -> (w798:T4)
        n62 = Bundle By Name(cluster=T3 {"Conn1/DIO_0_7 In"={"Conn1/DIO_0_7 - 75kHz"=FALSE, "Conn1/DIO_0_7 - uSec On"=0, "Conn1/DIO_0_7 In"=[FALSE, FALSE, FALSE, FALSE, FALSE, FALSE, FALSE, FALSE], "Conn1/DIO_0_7 - uSec Off"=0}, "Conn1/DIO_8_15 In"={"Conn1/DIO_8_15 - 75kHz"=FALSE, "Conn1/DIO_8_15 - uSec On"=0, "Conn1/DIO_8_15 In"=[FALSE, FALSE, FALSE, FALSE, FALSE, FALSE, FALSE, FALSE], "Conn1/DIO_8_15 - uSec Off"=0}, "Conn1/DIO_16_23 In"={"Conn1/DIO_16_23 - 75kHz"=FALSE, "Conn1/DIO_16_23 - uSec On"=0, "Conn1/DIO_16_23 In"=[FALSE, FALSE, FALSE, FALSE, FALSE, FALSE, FALSE, FALSE], "Conn1/DIO_16_23 - uSec Off"=0}, "Conn1/DIO_24_31 In"={"Conn1/DIO_24_31 - 75kHz"=FALSE, "Conn1/DIO_24_31 - uSec On"=0, "Conn1/DIO_24_31 In"=[FALSE, FALSE, FALSE, FALSE, FALSE, FALSE, FALSE, FALSE], "Conn1/DIO_24_31 - uSec Off"=0}, "Conn1/DIO_32_39 In"={"Conn1/DIO_32_39 - 75kHz"=FALSE, "Conn1/DIO_32_39 - uSec On"=0, "Conn1/DIO_32_39 In"=[FALSE, FALSE, FALSE, FALSE, FALSE, FALSE, FALSE, FALSE], "Conn1/DIO_32_39 - uSec Off"=0}} ("Conn1 DIOs In"), "Conn1/DIO_0_7 In.Conn1/DIO_0_7 - 75kHz"=w803, "Conn1/DIO_0_7 In.Conn1/DIO_0_7 - uSec On"=w804, "Conn1/DIO_0_7 In.Conn1/DIO_0_7 In"=w805, "Conn1/DIO_0_7 In.Conn1/DIO_0_7 - uSec Off"=w806, "Conn1/DIO_8_15 In.Conn1/DIO_8_15 - 75kHz"=w790, "Conn1/DIO_8_15 In.Conn1/DIO_8_15 - uSec On"=w789, "Conn1/DIO_8_15 In.Conn1/DIO_8_15 In"=w788, "Conn1/DIO_8_15 In.Conn1/DIO_8_15 - uSec Off"=w787, "Conn1/DIO_16_23 In.Conn1/DIO_16_23 - 75kHz"=w786, "Conn1/DIO_16_23 In.Conn1/DIO_16_23 - uSec On"=w785, "Conn1/DIO_16_23 In.Conn1/DIO_16_23 In"=w784, "Conn1/DIO_16_23 In.Conn1/DIO_16_23 - uSec Off"=w783, "Conn1/DIO_24_31 In.Conn1/DIO_24_31 - 75kHz"=w782, "Conn1/DIO_24_31 In.Conn1/DIO_24_31 - uSec On"=w781, "Conn1/DIO_24_31 In.Conn1/DIO_24_31 In"=w780, "Conn1/DIO_24_31 In.Conn1/DIO_24_31 - uSec Off"=w779, "Conn1/DIO_32_39 In.Conn1/DIO_32_39 - 75kHz"=w778, "Conn1/DIO_32_39 In.Conn1/DIO_32_39 - uSec On"=w777, "Conn1/DIO_32_39 In.Conn1/DIO_32_39 In"=w776, "Conn1/DIO_32_39 In.Conn1/DIO_32_39 - uSec Off"=w775) -> (w811:T3)
        n63 = Bundle By Name(cluster=T2 {"Conn2/DIO_0_7 In"={"Conn2/DIO_0_7 - 75kHz"=FALSE, "Conn2/DIO_0_7 - uSec On"=0, "Conn2/DIO_0_7 In"=[FALSE, FALSE, FALSE, FALSE, FALSE, FALSE, FALSE, FALSE], "Conn2/DIO_0_7 - uSec Off"=0}, "Conn2/DIO_8_15 In"={"Conn2/DIO_8_15 - 75kHz"=FALSE, "Conn2/DIO_8_15 - uSec On"=0, "Conn2/DIO_8_15 In"=[FALSE, FALSE, FALSE, FALSE, FALSE, FALSE, FALSE, FALSE], "Conn2/DIO_8_15 - uSec Off"=0}, "Conn2/DIO_16_23 In"={"Conn2/DIO_16_23 - 75kHz"=FALSE, "Conn2/DIO_16_23 - uSec On"=0, "Conn2/DIO_16_23 In"=[FALSE, FALSE, FALSE, FALSE, FALSE, FALSE, FALSE, FALSE], "Conn2/DIO_16_23 - uSec Off"=0}, "Conn2/DIO_24_31 In"={"Conn2/DIO_24_31 - 75kHz"=FALSE, "Conn2/DIO_24_31 - uSec On"=0, "Conn2/DIO_24_31 In"=[FALSE, FALSE, FALSE, FALSE, FALSE, FALSE, FALSE, FALSE], "Conn2/DIO_24_31 - uSec Off"=0}, "Conn2/DIO_32_39 In"={"Conn2/DIO_32_39 - 75kHz"=FALSE, "Conn2/DIO_32_39 - uSec On"=0, "Conn2/DIO_32_39 In"=[FALSE, FALSE, FALSE, FALSE, FALSE, FALSE, FALSE, FALSE], "Conn2/DIO_32_39 - uSec Off"=0}} ("Conn2 DIOs In"), "Conn2/DIO_0_7 In.Conn2/DIO_0_7 - 75kHz"=w800, "Conn2/DIO_0_7 In.Conn2/DIO_0_7 - uSec On"=w801, "Conn2/DIO_0_7 In.Conn2/DIO_0_7 In"=w744, "Conn2/DIO_0_7 In.Conn2/DIO_0_7 - uSec Off"=w802, "Conn2/DIO_8_15 In.Conn2/DIO_8_15 - 75kHz"=w766, "Conn2/DIO_8_15 In.Conn2/DIO_8_15 - uSec On"=w765, "Conn2/DIO_8_15 In.Conn2/DIO_8_15 In"=w764, "Conn2/DIO_8_15 In.Conn2/DIO_8_15 - uSec Off"=w763, "Conn2/DIO_16_23 In.Conn2/DIO_16_23 - 75kHz"=w762, "Conn2/DIO_16_23 In.Conn2/DIO_16_23 - uSec On"=w761, "Conn2/DIO_16_23 In.Conn2/DIO_16_23 In"=w760, "Conn2/DIO_16_23 In.Conn2/DIO_16_23 - uSec Off"=w759, "Conn2/DIO_24_31 In.Conn2/DIO_24_31 - 75kHz"=w758, "Conn2/DIO_24_31 In.Conn2/DIO_24_31 - uSec On"=w757, "Conn2/DIO_24_31 In.Conn2/DIO_24_31 In"=w756, "Conn2/DIO_24_31 In.Conn2/DIO_24_31 - uSec Off"=w755, "Conn2/DIO_32_39 In.Conn2/DIO_32_39 - 75kHz"=w754, "Conn2/DIO_32_39 In.Conn2/DIO_32_39 - uSec On"=w753, "Conn2/DIO_32_39 In.Conn2/DIO_32_39 In"=w752, "Conn2/DIO_32_39 In.Conn2/DIO_32_39 - uSec Off"=w751) -> (w812:T2)
        n64 = Build Array(w774, w773, w772, w771, w770, w769, w768, w767) -> (w813:i16[])
        n65 = xnode "Read/Write Control"("FPGA VI Reference In"=w795, "Conn0 DIOs In"=w798, "Conn1 DIOs In"=w811, "Conn2 DIOs In"=w812, "Connector0/AO0_7"=w813) -> ("FPGA VI Reference Out"=w796:refnum<k20>)  [unwired: 1 in, 1 out]
      }
      frame "Triverse Power 2" {
        w822 = FALSE  # Conn2/DIO_7
        w821 = FALSE  # Conn2/DIO_6
        w814 = FALSE  # Conn2/DIO_5
        w815 = TRUE  # Conn2/DIO_4
        w816 = TRUE  # Conn2/DIO_3
        w820 = TRUE  # Conn2/DIO_2
        w819 = FALSE  # Conn2/DIO_1
        w818 = FALSE  # Conn2/DIO_0
        w824 = u16 0  # Conn2/DIO_32_39 - uSec Off
        w825 = bool[] [FALSE, FALSE, FALSE, FALSE, FALSE, FALSE, FALSE, FALSE]  # Conn2/DIO_32_39 In
        w826 = u16 0  # Conn2/DIO_32_39 - uSec On
        w827 = FALSE  # Conn2/DIO_32_39 - 75kHz
        w828 = u16 0  # Conn2/DIO_24_31 - uSec Off
        w829 = bool[] [FALSE, FALSE, FALSE, FALSE, FALSE, FALSE, FALSE, FALSE]  # Conn2/DIO_24_31 In
        w830 = u16 0  # Conn2/DIO_24_31 - uSec On
        w831 = FALSE  # Conn2/DIO_24_31 - 75kHz
        w832 = u16 0  # Conn2/DIO_16_23 - uSec Off
        w833 = bool[] [FALSE, FALSE, FALSE, FALSE, FALSE, FALSE, FALSE, FALSE]  # Conn2/DIO_16_23 In
        w834 = u16 0  # Conn2/DIO_16_23 - uSec On
        w835 = FALSE  # Conn2/DIO_16_23 - 75kHz
        w836 = u16 6  # Conn2/DIO_8_15 - uSec Off
        w837 = bool[] [FALSE, TRUE, FALSE, FALSE, FALSE, FALSE, FALSE, FALSE]  # Conn2/DIO_8_15 In
        w838 = u16 7  # Conn2/DIO_8_15 - uSec On
        w839 = TRUE  # Conn2/DIO_8_15 - 75kHz
        w840 = i16 0  # Connector0/AO7
        w841 = i16 0  # Connector0/AO6
        w842 = i16 0  # Connector0/AO5
        w843 = i16 0  # Connector0/AO4
        w844 = i16 0  # Connector0/AO3
        w845 = i16 0  # Connector0/AO2
        w846 = i16 0  # Connector0/AO1
        w847 = i16 0  # Connector0/AO0
        w848 = u16 0  # Conn1/DIO_32_39 - uSec Off
        w849 = bool[] [FALSE, FALSE, FALSE, FALSE, FALSE, FALSE, FALSE, FALSE]  # Conn1/DIO_32_39 In
        w850 = u16 0  # Conn1/DIO_32_39 - uSec On
        w851 = FALSE  # Conn1/DIO_32_39 - 75kHz
        w852 = u16 0  # Conn1/DIO_24_31 - uSec Off
        w853 = bool[] [FALSE, FALSE, FALSE, FALSE, FALSE, FALSE, FALSE, FALSE]  # Conn1/DIO_24_31 In
        w854 = u16 0  # Conn1/DIO_24_31 - uSec On
        w855 = FALSE  # Conn1/DIO_24_31 - 75kHz
        w856 = u16 6  # Conn1/DIO_16_23 - uSec Off
        w857 = bool[] [FALSE, TRUE, FALSE, FALSE, FALSE, FALSE, FALSE, FALSE]  # Conn1/DIO_16_23 In
        w858 = u16 7  # Conn1/DIO_16_23 - uSec On
        w859 = TRUE  # Conn1/DIO_16_23 - 75kHz
        w860 = u16 6  # Conn1/DIO_8_15 - uSec Off
        w861 = bool[] [FALSE, FALSE, FALSE, TRUE, FALSE, FALSE, FALSE, FALSE]  # Conn1/DIO_8_15 In
        w862 = u16 7  # Conn1/DIO_8_15 - uSec On
        w863 = TRUE  # Conn1/DIO_8_15 - 75kHz
        w864 = u16 0  # Conn0/DIO_8_15 - uSec Off
        w865 = bool[] [FALSE, FALSE, FALSE, FALSE, FALSE, FALSE, FALSE, FALSE]  # Conn0/DIO_8_15 In
        w866 = u16 0  # Conn0/DIO_8_15 - uSec On
        w867 = FALSE  # Conn0/DIO_8_15 - 75kHz
        w883 = u16 0  # Conn0/DIO_0_7 - uSec Off
        w882 = bool[] [FALSE, FALSE, FALSE, FALSE, FALSE, FALSE, FALSE, FALSE]  # Conn0/DIO_0_7 In
        w881 = u16 0  # Conn0/DIO_0_7 - uSec On
        w880 = FALSE  # Conn0/DIO_0_7 - 75kHz
        w879 = u16 6  # Conn1/DIO_0_7 - uSec Off
        w878 = bool[] [FALSE, TRUE, TRUE, TRUE, TRUE, FALSE, FALSE, TRUE]  # Conn1/DIO_0_7 In
        w877 = u16 7  # Conn1/DIO_0_7 - uSec On
        w876 = TRUE  # Conn1/DIO_0_7 - 75kHz
        w875 = u16 6  # Conn2/DIO_0_7 - uSec Off
        w874 = u16 7  # Conn2/DIO_0_7 - uSec On
        w873 = TRUE  # Conn2/DIO_0_7 - 75kHz
        # "Triverse Power 2"
        # "Triverse Power 2"
        # "Triverse Power 2"
        n66 = Build Array(w818, w819, w820, w816, w815, w814, w821, w822) -> (w817:bool[])
        n67 = Bundle By Name(cluster=T4 {"Conn0/DIO_0_7 In"={"Conn0/DIO_0_7 - 75kHz"=FALSE, "Conn0/DIO_0_7 - uSec On"=0, "Conn0/DIO_0_7 In"=[FALSE, FALSE, FALSE, FALSE, FALSE, FALSE, FALSE, FALSE], "Conn0/DIO_0_7 - uSec Off"=0}, "Conn0/DIO_8_15 In"={"Conn0/DIO_8_15 - 75kHz"=FALSE, "Conn0/DIO_8_15 - uSec On"=0, "Conn0/DIO_8_15 In"=[FALSE, FALSE, FALSE, FALSE, FALSE, FALSE, FALSE, FALSE], "Conn0/DIO_8_15 - uSec Off"=0}} ("Conn0 DIOs In"), "Conn0/DIO_0_7 In.Conn0/DIO_0_7 - 75kHz"=w880, "Conn0/DIO_0_7 In.Conn0/DIO_0_7 - uSec On"=w881, "Conn0/DIO_0_7 In.Conn0/DIO_0_7 In"=w882, "Conn0/DIO_0_7 In.Conn0/DIO_0_7 - uSec Off"=w883, "Conn0/DIO_8_15 In.Conn0/DIO_8_15 - 75kHz"=w867, "Conn0/DIO_8_15 In.Conn0/DIO_8_15 - uSec On"=w866, "Conn0/DIO_8_15 In.Conn0/DIO_8_15 In"=w865, "Conn0/DIO_8_15 In.Conn0/DIO_8_15 - uSec Off"=w864) -> (w871:T4)
        n68 = Bundle By Name(cluster=T3 {"Conn1/DIO_0_7 In"={"Conn1/DIO_0_7 - 75kHz"=FALSE, "Conn1/DIO_0_7 - uSec On"=0, "Conn1/DIO_0_7 In"=[FALSE, FALSE, FALSE, FALSE, FALSE, FALSE, FALSE, FALSE], "Conn1/DIO_0_7 - uSec Off"=0}, "Conn1/DIO_8_15 In"={"Conn1/DIO_8_15 - 75kHz"=FALSE, "Conn1/DIO_8_15 - uSec On"=0, "Conn1/DIO_8_15 In"=[FALSE, FALSE, FALSE, FALSE, FALSE, FALSE, FALSE, FALSE], "Conn1/DIO_8_15 - uSec Off"=0}, "Conn1/DIO_16_23 In"={"Conn1/DIO_16_23 - 75kHz"=FALSE, "Conn1/DIO_16_23 - uSec On"=0, "Conn1/DIO_16_23 In"=[FALSE, FALSE, FALSE, FALSE, FALSE, FALSE, FALSE, FALSE], "Conn1/DIO_16_23 - uSec Off"=0}, "Conn1/DIO_24_31 In"={"Conn1/DIO_24_31 - 75kHz"=FALSE, "Conn1/DIO_24_31 - uSec On"=0, "Conn1/DIO_24_31 In"=[FALSE, FALSE, FALSE, FALSE, FALSE, FALSE, FALSE, FALSE], "Conn1/DIO_24_31 - uSec Off"=0}, "Conn1/DIO_32_39 In"={"Conn1/DIO_32_39 - 75kHz"=FALSE, "Conn1/DIO_32_39 - uSec On"=0, "Conn1/DIO_32_39 In"=[FALSE, FALSE, FALSE, FALSE, FALSE, FALSE, FALSE, FALSE], "Conn1/DIO_32_39 - uSec Off"=0}} ("Conn1 DIOs In"), "Conn1/DIO_0_7 In.Conn1/DIO_0_7 - 75kHz"=w876, "Conn1/DIO_0_7 In.Conn1/DIO_0_7 - uSec On"=w877, "Conn1/DIO_0_7 In.Conn1/DIO_0_7 In"=w878, "Conn1/DIO_0_7 In.Conn1/DIO_0_7 - uSec Off"=w879, "Conn1/DIO_8_15 In.Conn1/DIO_8_15 - 75kHz"=w863, "Conn1/DIO_8_15 In.Conn1/DIO_8_15 - uSec On"=w862, "Conn1/DIO_8_15 In.Conn1/DIO_8_15 In"=w861, "Conn1/DIO_8_15 In.Conn1/DIO_8_15 - uSec Off"=w860, "Conn1/DIO_16_23 In.Conn1/DIO_16_23 - 75kHz"=w859, "Conn1/DIO_16_23 In.Conn1/DIO_16_23 - uSec On"=w858, "Conn1/DIO_16_23 In.Conn1/DIO_16_23 In"=w857, "Conn1/DIO_16_23 In.Conn1/DIO_16_23 - uSec Off"=w856, "Conn1/DIO_24_31 In.Conn1/DIO_24_31 - 75kHz"=w855, "Conn1/DIO_24_31 In.Conn1/DIO_24_31 - uSec On"=w854, "Conn1/DIO_24_31 In.Conn1/DIO_24_31 In"=w853, "Conn1/DIO_24_31 In.Conn1/DIO_24_31 - uSec Off"=w852, "Conn1/DIO_32_39 In.Conn1/DIO_32_39 - 75kHz"=w851, "Conn1/DIO_32_39 In.Conn1/DIO_32_39 - uSec On"=w850, "Conn1/DIO_32_39 In.Conn1/DIO_32_39 In"=w849, "Conn1/DIO_32_39 In.Conn1/DIO_32_39 - uSec Off"=w848) -> (w884:T3)
        n69 = Bundle By Name(cluster=T2 {"Conn2/DIO_0_7 In"={"Conn2/DIO_0_7 - 75kHz"=FALSE, "Conn2/DIO_0_7 - uSec On"=0, "Conn2/DIO_0_7 In"=[FALSE, FALSE, FALSE, FALSE, FALSE, FALSE, FALSE, FALSE], "Conn2/DIO_0_7 - uSec Off"=0}, "Conn2/DIO_8_15 In"={"Conn2/DIO_8_15 - 75kHz"=FALSE, "Conn2/DIO_8_15 - uSec On"=0, "Conn2/DIO_8_15 In"=[FALSE, FALSE, FALSE, FALSE, FALSE, FALSE, FALSE, FALSE], "Conn2/DIO_8_15 - uSec Off"=0}, "Conn2/DIO_16_23 In"={"Conn2/DIO_16_23 - 75kHz"=FALSE, "Conn2/DIO_16_23 - uSec On"=0, "Conn2/DIO_16_23 In"=[FALSE, FALSE, FALSE, FALSE, FALSE, FALSE, FALSE, FALSE], "Conn2/DIO_16_23 - uSec Off"=0}, "Conn2/DIO_24_31 In"={"Conn2/DIO_24_31 - 75kHz"=FALSE, "Conn2/DIO_24_31 - uSec On"=0, "Conn2/DIO_24_31 In"=[FALSE, FALSE, FALSE, FALSE, FALSE, FALSE, FALSE, FALSE], "Conn2/DIO_24_31 - uSec Off"=0}, "Conn2/DIO_32_39 In"={"Conn2/DIO_32_39 - 75kHz"=FALSE, "Conn2/DIO_32_39 - uSec On"=0, "Conn2/DIO_32_39 In"=[FALSE, FALSE, FALSE, FALSE, FALSE, FALSE, FALSE, FALSE], "Conn2/DIO_32_39 - uSec Off"=0}} ("Conn2 DIOs In"), "Conn2/DIO_0_7 In.Conn2/DIO_0_7 - 75kHz"=w873, "Conn2/DIO_0_7 In.Conn2/DIO_0_7 - uSec On"=w874, "Conn2/DIO_0_7 In.Conn2/DIO_0_7 In"=w817, "Conn2/DIO_0_7 In.Conn2/DIO_0_7 - uSec Off"=w875, "Conn2/DIO_8_15 In.Conn2/DIO_8_15 - 75kHz"=w839, "Conn2/DIO_8_15 In.Conn2/DIO_8_15 - uSec On"=w838, "Conn2/DIO_8_15 In.Conn2/DIO_8_15 In"=w837, "Conn2/DIO_8_15 In.Conn2/DIO_8_15 - uSec Off"=w836, "Conn2/DIO_16_23 In.Conn2/DIO_16_23 - 75kHz"=w835, "Conn2/DIO_16_23 In.Conn2/DIO_16_23 - uSec On"=w834, "Conn2/DIO_16_23 In.Conn2/DIO_16_23 In"=w833, "Conn2/DIO_16_23 In.Conn2/DIO_16_23 - uSec Off"=w832, "Conn2/DIO_24_31 In.Conn2/DIO_24_31 - 75kHz"=w831, "Conn2/DIO_24_31 In.Conn2/DIO_24_31 - uSec On"=w830, "Conn2/DIO_24_31 In.Conn2/DIO_24_31 In"=w829, "Conn2/DIO_24_31 In.Conn2/DIO_24_31 - uSec Off"=w828, "Conn2/DIO_32_39 In.Conn2/DIO_32_39 - 75kHz"=w827, "Conn2/DIO_32_39 In.Conn2/DIO_32_39 - uSec On"=w826, "Conn2/DIO_32_39 In.Conn2/DIO_32_39 In"=w825, "Conn2/DIO_32_39 In.Conn2/DIO_32_39 - uSec Off"=w824) -> (w885:T2)
        n70 = Build Array(w847, w846, w845, w844, w843, w842, w841, w840) -> (w886:i16[])
        n71 = xnode "Read/Write Control"("FPGA VI Reference In"=w868, "Conn0 DIOs In"=w871, "Conn1 DIOs In"=w884, "Conn2 DIOs In"=w885, "Connector0/AO0_7"=w886) -> ("FPGA VI Reference Out"=w869:refnum<k20>)  [unwired: 1 in, 1 out]
      }
      frame "Triverse Power 3" {
        w895 = FALSE  # Conn2/DIO_7
        w894 = FALSE  # Conn2/DIO_6
        w887 = FALSE  # Conn2/DIO_5
        w888 = FALSE  # Conn2/DIO_4
        w889 = FALSE  # Conn2/DIO_3
        w893 = TRUE  # Conn2/DIO_2
        w892 = FALSE  # Conn2/DIO_1
        w891 = FALSE  # Conn2/DIO_0
        w897 = u16 0  # Conn2/DIO_32_39 - uSec Off
        w898 = bool[] [FALSE, FALSE, FALSE, FALSE, FALSE, FALSE, FALSE, FALSE]  # Conn2/DIO_32_39 In
        w899 = u16 0  # Conn2/DIO_32_39 - uSec On
        w900 = FALSE  # Conn2/DIO_32_39 - 75kHz
        w901 = u16 0  # Conn2/DIO_24_31 - uSec Off
        w902 = bool[] [FALSE, FALSE, FALSE, FALSE, FALSE, FALSE, FALSE, FALSE]  # Conn2/DIO_24_31 In
        w903 = u16 0  # Conn2/DIO_24_31 - uSec On
        w904 = FALSE  # Conn2/DIO_24_31 - 75kHz
        w905 = u16 0  # Conn2/DIO_16_23 - uSec Off
        w906 = bool[] [FALSE, FALSE, FALSE, FALSE, FALSE, FALSE, FALSE, FALSE]  # Conn2/DIO_16_23 In
        w907 = u16 0  # Conn2/DIO_16_23 - uSec On
        w908 = FALSE  # Conn2/DIO_16_23 - 75kHz
        w909 = u16 6  # Conn2/DIO_8_15 - uSec Off
        w910 = bool[] [FALSE, TRUE, FALSE, FALSE, FALSE, FALSE, FALSE, FALSE]  # Conn2/DIO_8_15 In
        w911 = u16 7  # Conn2/DIO_8_15 - uSec On
        w912 = TRUE  # Conn2/DIO_8_15 - 75kHz
        w913 = i16 0  # Connector0/AO7
        w914 = i16 0  # Connector0/AO6
        w915 = i16 0  # Connector0/AO5
        w916 = i16 0  # Connector0/AO4
        w917 = i16 0  # Connector0/AO3
        w918 = i16 0  # Connector0/AO2
        w919 = i16 0  # Connector0/AO1
        w920 = i16 0  # Connector0/AO0
        w921 = u16 0  # Conn1/DIO_32_39 - uSec Off
        w922 = bool[] [FALSE, FALSE, FALSE, FALSE, FALSE, FALSE, FALSE, FALSE]  # Conn1/DIO_32_39 In
        w923 = u16 0  # Conn1/DIO_32_39 - uSec On
        w924 = FALSE  # Conn1/DIO_32_39 - 75kHz
        w925 = u16 0  # Conn1/DIO_24_31 - uSec Off
        w926 = bool[] [FALSE, FALSE, FALSE, FALSE, FALSE, FALSE, FALSE, FALSE]  # Conn1/DIO_24_31 In
        w927 = u16 0  # Conn1/DIO_24_31 - uSec On
        w928 = FALSE  # Conn1/DIO_24_31 - 75kHz
        w929 = u16 6  # Conn1/DIO_16_23 - uSec Off
        w930 = bool[] [FALSE, TRUE, FALSE, FALSE, FALSE, FALSE, FALSE, FALSE]  # Conn1/DIO_16_23 In
        w931 = u16 7  # Conn1/DIO_16_23 - uSec On
        w932 = TRUE  # Conn1/DIO_16_23 - 75kHz
        w933 = u16 6  # Conn1/DIO_8_15 - uSec Off
        w934 = bool[] [FALSE, FALSE, FALSE, TRUE, FALSE, FALSE, FALSE, FALSE]  # Conn1/DIO_8_15 In
        w935 = u16 7  # Conn1/DIO_8_15 - uSec On
        w936 = TRUE  # Conn1/DIO_8_15 - 75kHz
        w937 = u16 0  # Conn0/DIO_8_15 - uSec Off
        w938 = bool[] [FALSE, FALSE, FALSE, FALSE, FALSE, FALSE, FALSE, FALSE]  # Conn0/DIO_8_15 In
        w939 = u16 0  # Conn0/DIO_8_15 - uSec On
        w940 = FALSE  # Conn0/DIO_8_15 - 75kHz
        w956 = u16 0  # Conn0/DIO_0_7 - uSec Off
        w955 = bool[] [FALSE, FALSE, FALSE, FALSE, FALSE, FALSE, FALSE, FALSE]  # Conn0/DIO_0_7 In
        w954 = u16 0  # Conn0/DIO_0_7 - uSec On
        w953 = FALSE  # Conn0/DIO_0_7 - 75kHz
        w952 = u16 6  # Conn1/DIO_0_7 - uSec Off
        w951 = bool[] [FALSE, TRUE, TRUE, TRUE, TRUE, FALSE, FALSE, TRUE]  # Conn1/DIO_0_7 In
        w950 = u16 7  # Conn1/DIO_0_7 - uSec On
        w949 = TRUE  # Conn1/DIO_0_7 - 75kHz
        w948 = u16 6  # Conn2/DIO_0_7 - uSec Off
        w947 = u16 7  # Conn2/DIO_0_7 - uSec On
        w946 = TRUE  # Conn2/DIO_0_7 - 75kHz
        # "Triverse Power 3"
        # "Triverse Power 3"
        # "Triverse Power 3"
        n72 = Build Array(w891, w892, w893, w889, w888, w887, w894, w895) -> (w890:bool[])
        n73 = Bundle By Name(cluster=T4 {"Conn0/DIO_0_7 In"={"Conn0/DIO_0_7 - 75kHz"=FALSE, "Conn0/DIO_0_7 - uSec On"=0, "Conn0/DIO_0_7 In"=[FALSE, FALSE, FALSE, FALSE, FALSE, FALSE, FALSE, FALSE], "Conn0/DIO_0_7 - uSec Off"=0}, "Conn0/DIO_8_15 In"={"Conn0/DIO_8_15 - 75kHz"=FALSE, "Conn0/DIO_8_15 - uSec On"=0, "Conn0/DIO_8_15 In"=[FALSE, FALSE, FALSE, FALSE, FALSE, FALSE, FALSE, FALSE], "Conn0/DIO_8_15 - uSec Off"=0}} ("Conn0 DIOs In"), "Conn0/DIO_0_7 In.Conn0/DIO_0_7 - 75kHz"=w953, "Conn0/DIO_0_7 In.Conn0/DIO_0_7 - uSec On"=w954, "Conn0/DIO_0_7 In.Conn0/DIO_0_7 In"=w955, "Conn0/DIO_0_7 In.Conn0/DIO_0_7 - uSec Off"=w956, "Conn0/DIO_8_15 In.Conn0/DIO_8_15 - 75kHz"=w940, "Conn0/DIO_8_15 In.Conn0/DIO_8_15 - uSec On"=w939, "Conn0/DIO_8_15 In.Conn0/DIO_8_15 In"=w938, "Conn0/DIO_8_15 In.Conn0/DIO_8_15 - uSec Off"=w937) -> (w944:T4)
        n74 = Bundle By Name(cluster=T3 {"Conn1/DIO_0_7 In"={"Conn1/DIO_0_7 - 75kHz"=FALSE, "Conn1/DIO_0_7 - uSec On"=0, "Conn1/DIO_0_7 In"=[FALSE, FALSE, FALSE, FALSE, FALSE, FALSE, FALSE, FALSE], "Conn1/DIO_0_7 - uSec Off"=0}, "Conn1/DIO_8_15 In"={"Conn1/DIO_8_15 - 75kHz"=FALSE, "Conn1/DIO_8_15 - uSec On"=0, "Conn1/DIO_8_15 In"=[FALSE, FALSE, FALSE, FALSE, FALSE, FALSE, FALSE, FALSE], "Conn1/DIO_8_15 - uSec Off"=0}, "Conn1/DIO_16_23 In"={"Conn1/DIO_16_23 - 75kHz"=FALSE, "Conn1/DIO_16_23 - uSec On"=0, "Conn1/DIO_16_23 In"=[FALSE, FALSE, FALSE, FALSE, FALSE, FALSE, FALSE, FALSE], "Conn1/DIO_16_23 - uSec Off"=0}, "Conn1/DIO_24_31 In"={"Conn1/DIO_24_31 - 75kHz"=FALSE, "Conn1/DIO_24_31 - uSec On"=0, "Conn1/DIO_24_31 In"=[FALSE, FALSE, FALSE, FALSE, FALSE, FALSE, FALSE, FALSE], "Conn1/DIO_24_31 - uSec Off"=0}, "Conn1/DIO_32_39 In"={"Conn1/DIO_32_39 - 75kHz"=FALSE, "Conn1/DIO_32_39 - uSec On"=0, "Conn1/DIO_32_39 In"=[FALSE, FALSE, FALSE, FALSE, FALSE, FALSE, FALSE, FALSE], "Conn1/DIO_32_39 - uSec Off"=0}} ("Conn1 DIOs In"), "Conn1/DIO_0_7 In.Conn1/DIO_0_7 - 75kHz"=w949, "Conn1/DIO_0_7 In.Conn1/DIO_0_7 - uSec On"=w950, "Conn1/DIO_0_7 In.Conn1/DIO_0_7 In"=w951, "Conn1/DIO_0_7 In.Conn1/DIO_0_7 - uSec Off"=w952, "Conn1/DIO_8_15 In.Conn1/DIO_8_15 - 75kHz"=w936, "Conn1/DIO_8_15 In.Conn1/DIO_8_15 - uSec On"=w935, "Conn1/DIO_8_15 In.Conn1/DIO_8_15 In"=w934, "Conn1/DIO_8_15 In.Conn1/DIO_8_15 - uSec Off"=w933, "Conn1/DIO_16_23 In.Conn1/DIO_16_23 - 75kHz"=w932, "Conn1/DIO_16_23 In.Conn1/DIO_16_23 - uSec On"=w931, "Conn1/DIO_16_23 In.Conn1/DIO_16_23 In"=w930, "Conn1/DIO_16_23 In.Conn1/DIO_16_23 - uSec Off"=w929, "Conn1/DIO_24_31 In.Conn1/DIO_24_31 - 75kHz"=w928, "Conn1/DIO_24_31 In.Conn1/DIO_24_31 - uSec On"=w927, "Conn1/DIO_24_31 In.Conn1/DIO_24_31 In"=w926, "Conn1/DIO_24_31 In.Conn1/DIO_24_31 - uSec Off"=w925, "Conn1/DIO_32_39 In.Conn1/DIO_32_39 - 75kHz"=w924, "Conn1/DIO_32_39 In.Conn1/DIO_32_39 - uSec On"=w923, "Conn1/DIO_32_39 In.Conn1/DIO_32_39 In"=w922, "Conn1/DIO_32_39 In.Conn1/DIO_32_39 - uSec Off"=w921) -> (w957:T3)
        n75 = Bundle By Name(cluster=T2 {"Conn2/DIO_0_7 In"={"Conn2/DIO_0_7 - 75kHz"=FALSE, "Conn2/DIO_0_7 - uSec On"=0, "Conn2/DIO_0_7 In"=[FALSE, FALSE, FALSE, FALSE, FALSE, FALSE, FALSE, FALSE], "Conn2/DIO_0_7 - uSec Off"=0}, "Conn2/DIO_8_15 In"={"Conn2/DIO_8_15 - 75kHz"=FALSE, "Conn2/DIO_8_15 - uSec On"=0, "Conn2/DIO_8_15 In"=[FALSE, FALSE, FALSE, FALSE, FALSE, FALSE, FALSE, FALSE], "Conn2/DIO_8_15 - uSec Off"=0}, "Conn2/DIO_16_23 In"={"Conn2/DIO_16_23 - 75kHz"=FALSE, "Conn2/DIO_16_23 - uSec On"=0, "Conn2/DIO_16_23 In"=[FALSE, FALSE, FALSE, FALSE, FALSE, FALSE, FALSE, FALSE], "Conn2/DIO_16_23 - uSec Off"=0}, "Conn2/DIO_24_31 In"={"Conn2/DIO_24_31 - 75kHz"=FALSE, "Conn2/DIO_24_31 - uSec On"=0, "Conn2/DIO_24_31 In"=[FALSE, FALSE, FALSE, FALSE, FALSE, FALSE, FALSE, FALSE], "Conn2/DIO_24_31 - uSec Off"=0}, "Conn2/DIO_32_39 In"={"Conn2/DIO_32_39 - 75kHz"=FALSE, "Conn2/DIO_32_39 - uSec On"=0, "Conn2/DIO_32_39 In"=[FALSE, FALSE, FALSE, FALSE, FALSE, FALSE, FALSE, FALSE], "Conn2/DIO_32_39 - uSec Off"=0}} ("Conn2 DIOs In"), "Conn2/DIO_0_7 In.Conn2/DIO_0_7 - 75kHz"=w946, "Conn2/DIO_0_7 In.Conn2/DIO_0_7 - uSec On"=w947, "Conn2/DIO_0_7 In.Conn2/DIO_0_7 In"=w890, "Conn2/DIO_0_7 In.Conn2/DIO_0_7 - uSec Off"=w948, "Conn2/DIO_8_15 In.Conn2/DIO_8_15 - 75kHz"=w912, "Conn2/DIO_8_15 In.Conn2/DIO_8_15 - uSec On"=w911, "Conn2/DIO_8_15 In.Conn2/DIO_8_15 In"=w910, "Conn2/DIO_8_15 In.Conn2/DIO_8_15 - uSec Off"=w909, "Conn2/DIO_16_23 In.Conn2/DIO_16_23 - 75kHz"=w908, "Conn2/DIO_16_23 In.Conn2/DIO_16_23 - uSec On"=w907, "Conn2/DIO_16_23 In.Conn2/DIO_16_23 In"=w906, "Conn2/DIO_16_23 In.Conn2/DIO_16_23 - uSec Off"=w905, "Conn2/DIO_24_31 In.Conn2/DIO_24_31 - 75kHz"=w904, "Conn2/DIO_24_31 In.Conn2/DIO_24_31 - uSec On"=w903, "Conn2/DIO_24_31 In.Conn2/DIO_24_31 In"=w902, "Conn2/DIO_24_31 In.Conn2/DIO_24_31 - uSec Off"=w901, "Conn2/DIO_32_39 In.Conn2/DIO_32_39 - 75kHz"=w900, "Conn2/DIO_32_39 In.Conn2/DIO_32_39 - uSec On"=w899, "Conn2/DIO_32_39 In.Conn2/DIO_32_39 In"=w898, "Conn2/DIO_32_39 In.Conn2/DIO_32_39 - uSec Off"=w897) -> (w958:T2)
        n76 = Build Array(w920, w919, w918, w917, w916, w915, w914, w913) -> (w959:i16[])
        n77 = xnode "Read/Write Control"("FPGA VI Reference In"=w941, "Conn0 DIOs In"=w944, "Conn1 DIOs In"=w957, "Conn2 DIOs In"=w958, "Connector0/AO0_7"=w959) -> ("FPGA VI Reference Out"=w942:refnum<k20>)  [unwired: 1 in, 1 out]
      }
      frame "Triverse Power 4" {
        w968 = FALSE  # Conn2/DIO_7
        w967 = FALSE  # Conn2/DIO_6
        w960 = TRUE  # Conn2/DIO_5
        w961 = FALSE  # Conn2/DIO_4
        w962 = TRUE  # Conn2/DIO_3
        w966 = TRUE  # Conn2/DIO_2
        w965 = FALSE  # Conn2/DIO_1
        w964 = FALSE  # Conn2/DIO_0
        w970 = u16 0  # Conn2/DIO_32_39 - uSec Off
        w971 = bool[] [FALSE, FALSE, FALSE, FALSE, FALSE, FALSE, FALSE, FALSE]  # Conn2/DIO_32_39 In
        w972 = u16 0  # Conn2/DIO_32_39 - uSec On
        w973 = FALSE  # Conn2/DIO_32_39 - 75kHz
        w974 = u16 0  # Conn2/DIO_24_31 - uSec Off
        w975 = bool[] [FALSE, FALSE, FALSE, FALSE, FALSE, FALSE, FALSE, FALSE]  # Conn2/DIO_24_31 In
        w976 = u16 0  # Conn2/DIO_24_31 - uSec On
        w977 = FALSE  # Conn2/DIO_24_31 - 75kHz
        w978 = u16 0  # Conn2/DIO_16_23 - uSec Off
        w979 = bool[] [FALSE, FALSE, FALSE, FALSE, FALSE, FALSE, FALSE, FALSE]  # Conn2/DIO_16_23 In
        w980 = u16 0  # Conn2/DIO_16_23 - uSec On
        w981 = FALSE  # Conn2/DIO_16_23 - 75kHz
        w982 = u16 6  # Conn2/DIO_8_15 - uSec Off
        w983 = bool[] [FALSE, TRUE, FALSE, FALSE, FALSE, FALSE, FALSE, FALSE]  # Conn2/DIO_8_15 In
        w984 = u16 7  # Conn2/DIO_8_15 - uSec On
        w985 = TRUE  # Conn2/DIO_8_15 - 75kHz
        w986 = i16 0  # Connector0/AO7
        w987 = i16 0  # Connector0/AO6
        w988 = i16 0  # Connector0/AO5
        w989 = i16 0  # Connector0/AO4
        w990 = i16 0  # Connector0/AO3
        w991 = i16 0  # Connector0/AO2
        w992 = i16 0  # Connector0/AO1
        w993 = i16 0  # Connector0/AO0
        w994 = u16 0  # Conn1/DIO_32_39 - uSec Off
        w995 = bool[] [FALSE, FALSE, FALSE, FALSE, FALSE, FALSE, FALSE, FALSE]  # Conn1/DIO_32_39 In
        w996 = u16 0  # Conn1/DIO_32_39 - uSec On
        w997 = FALSE  # Conn1/DIO_32_39 - 75kHz
        w998 = u16 0  # Conn1/DIO_24_31 - uSec Off
        w999 = bool[] [FALSE, FALSE, FALSE, FALSE, FALSE, FALSE, FALSE, FALSE]  # Conn1/DIO_24_31 In
        w1000 = u16 0  # Conn1/DIO_24_31 - uSec On
        w1001 = FALSE  # Conn1/DIO_24_31 - 75kHz
        w1002 = u16 6  # Conn1/DIO_16_23 - uSec Off
        w1003 = bool[] [FALSE, TRUE, FALSE, FALSE, FALSE, FALSE, FALSE, FALSE]  # Conn1/DIO_16_23 In
        w1004 = u16 7  # Conn1/DIO_16_23 - uSec On
        w1005 = TRUE  # Conn1/DIO_16_23 - 75kHz
        w1006 = u16 6  # Conn1/DIO_8_15 - uSec Off
        w1007 = bool[] [FALSE, FALSE, FALSE, TRUE, FALSE, FALSE, FALSE, FALSE]  # Conn1/DIO_8_15 In
        w1008 = u16 7  # Conn1/DIO_8_15 - uSec On
        w1009 = TRUE  # Conn1/DIO_8_15 - 75kHz
        w1010 = u16 0  # Conn0/DIO_8_15 - uSec Off
        w1011 = bool[] [FALSE, FALSE, FALSE, FALSE, FALSE, FALSE, FALSE, FALSE]  # Conn0/DIO_8_15 In
        w1012 = u16 0  # Conn0/DIO_8_15 - uSec On
        w1013 = FALSE  # Conn0/DIO_8_15 - 75kHz
        w1029 = u16 0  # Conn0/DIO_0_7 - uSec Off
        w1028 = bool[] [FALSE, FALSE, FALSE, FALSE, FALSE, FALSE, FALSE, FALSE]  # Conn0/DIO_0_7 In
        w1027 = u16 0  # Conn0/DIO_0_7 - uSec On
        w1026 = FALSE  # Conn0/DIO_0_7 - 75kHz
        w1025 = u16 6  # Conn1/DIO_0_7 - uSec Off
        w1024 = bool[] [FALSE, TRUE, TRUE, TRUE, TRUE, FALSE, FALSE, TRUE]  # Conn1/DIO_0_7 In
        w1023 = u16 7  # Conn1/DIO_0_7 - uSec On
        w1022 = TRUE  # Conn1/DIO_0_7 - 75kHz
        w1021 = u16 6  # Conn2/DIO_0_7 - uSec Off
        w1020 = u16 7  # Conn2/DIO_0_7 - uSec On
        w1019 = TRUE  # Conn2/DIO_0_7 - 75kHz
        # "Triverse Power 4"
        # "Triverse Power 4"
        # "Triverse Power 4"
        n78 = Build Array(w964, w965, w966, w962, w961, w960, w967, w968) -> (w963:bool[])
        n79 = Bundle By Name(cluster=T4 {"Conn0/DIO_0_7 In"={"Conn0/DIO_0_7 - 75kHz"=FALSE, "Conn0/DIO_0_7 - uSec On"=0, "Conn0/DIO_0_7 In"=[FALSE, FALSE, FALSE, FALSE, FALSE, FALSE, FALSE, FALSE], "Conn0/DIO_0_7 - uSec Off"=0}, "Conn0/DIO_8_15 In"={"Conn0/DIO_8_15 - 75kHz"=FALSE, "Conn0/DIO_8_15 - uSec On"=0, "Conn0/DIO_8_15 In"=[FALSE, FALSE, FALSE, FALSE, FALSE, FALSE, FALSE, FALSE], "Conn0/DIO_8_15 - uSec Off"=0}} ("Conn0 DIOs In"), "Conn0/DIO_0_7 In.Conn0/DIO_0_7 - 75kHz"=w1026, "Conn0/DIO_0_7 In.Conn0/DIO_0_7 - uSec On"=w1027, "Conn0/DIO_0_7 In.Conn0/DIO_0_7 In"=w1028, "Conn0/DIO_0_7 In.Conn0/DIO_0_7 - uSec Off"=w1029, "Conn0/DIO_8_15 In.Conn0/DIO_8_15 - 75kHz"=w1013, "Conn0/DIO_8_15 In.Conn0/DIO_8_15 - uSec On"=w1012, "Conn0/DIO_8_15 In.Conn0/DIO_8_15 In"=w1011, "Conn0/DIO_8_15 In.Conn0/DIO_8_15 - uSec Off"=w1010) -> (w1017:T4)
        n80 = Bundle By Name(cluster=T3 {"Conn1/DIO_0_7 In"={"Conn1/DIO_0_7 - 75kHz"=FALSE, "Conn1/DIO_0_7 - uSec On"=0, "Conn1/DIO_0_7 In"=[FALSE, FALSE, FALSE, FALSE, FALSE, FALSE, FALSE, FALSE], "Conn1/DIO_0_7 - uSec Off"=0}, "Conn1/DIO_8_15 In"={"Conn1/DIO_8_15 - 75kHz"=FALSE, "Conn1/DIO_8_15 - uSec On"=0, "Conn1/DIO_8_15 In"=[FALSE, FALSE, FALSE, FALSE, FALSE, FALSE, FALSE, FALSE], "Conn1/DIO_8_15 - uSec Off"=0}, "Conn1/DIO_16_23 In"={"Conn1/DIO_16_23 - 75kHz"=FALSE, "Conn1/DIO_16_23 - uSec On"=0, "Conn1/DIO_16_23 In"=[FALSE, FALSE, FALSE, FALSE, FALSE, FALSE, FALSE, FALSE], "Conn1/DIO_16_23 - uSec Off"=0}, "Conn1/DIO_24_31 In"={"Conn1/DIO_24_31 - 75kHz"=FALSE, "Conn1/DIO_24_31 - uSec On"=0, "Conn1/DIO_24_31 In"=[FALSE, FALSE, FALSE, FALSE, FALSE, FALSE, FALSE, FALSE], "Conn1/DIO_24_31 - uSec Off"=0}, "Conn1/DIO_32_39 In"={"Conn1/DIO_32_39 - 75kHz"=FALSE, "Conn1/DIO_32_39 - uSec On"=0, "Conn1/DIO_32_39 In"=[FALSE, FALSE, FALSE, FALSE, FALSE, FALSE, FALSE, FALSE], "Conn1/DIO_32_39 - uSec Off"=0}} ("Conn1 DIOs In"), "Conn1/DIO_0_7 In.Conn1/DIO_0_7 - 75kHz"=w1022, "Conn1/DIO_0_7 In.Conn1/DIO_0_7 - uSec On"=w1023, "Conn1/DIO_0_7 In.Conn1/DIO_0_7 In"=w1024, "Conn1/DIO_0_7 In.Conn1/DIO_0_7 - uSec Off"=w1025, "Conn1/DIO_8_15 In.Conn1/DIO_8_15 - 75kHz"=w1009, "Conn1/DIO_8_15 In.Conn1/DIO_8_15 - uSec On"=w1008, "Conn1/DIO_8_15 In.Conn1/DIO_8_15 In"=w1007, "Conn1/DIO_8_15 In.Conn1/DIO_8_15 - uSec Off"=w1006, "Conn1/DIO_16_23 In.Conn1/DIO_16_23 - 75kHz"=w1005, "Conn1/DIO_16_23 In.Conn1/DIO_16_23 - uSec On"=w1004, "Conn1/DIO_16_23 In.Conn1/DIO_16_23 In"=w1003, "Conn1/DIO_16_23 In.Conn1/DIO_16_23 - uSec Off"=w1002, "Conn1/DIO_24_31 In.Conn1/DIO_24_31 - 75kHz"=w1001, "Conn1/DIO_24_31 In.Conn1/DIO_24_31 - uSec On"=w1000, "Conn1/DIO_24_31 In.Conn1/DIO_24_31 In"=w999, "Conn1/DIO_24_31 In.Conn1/DIO_24_31 - uSec Off"=w998, "Conn1/DIO_32_39 In.Conn1/DIO_32_39 - 75kHz"=w997, "Conn1/DIO_32_39 In.Conn1/DIO_32_39 - uSec On"=w996, "Conn1/DIO_32_39 In.Conn1/DIO_32_39 In"=w995, "Conn1/DIO_32_39 In.Conn1/DIO_32_39 - uSec Off"=w994) -> (w1030:T3)
        n81 = Bundle By Name(cluster=T2 {"Conn2/DIO_0_7 In"={"Conn2/DIO_0_7 - 75kHz"=FALSE, "Conn2/DIO_0_7 - uSec On"=0, "Conn2/DIO_0_7 In"=[FALSE, FALSE, FALSE, FALSE, FALSE, FALSE, FALSE, FALSE], "Conn2/DIO_0_7 - uSec Off"=0}, "Conn2/DIO_8_15 In"={"Conn2/DIO_8_15 - 75kHz"=FALSE, "Conn2/DIO_8_15 - uSec On"=0, "Conn2/DIO_8_15 In"=[FALSE, FALSE, FALSE, FALSE, FALSE, FALSE, FALSE, FALSE], "Conn2/DIO_8_15 - uSec Off"=0}, "Conn2/DIO_16_23 In"={"Conn2/DIO_16_23 - 75kHz"=FALSE, "Conn2/DIO_16_23 - uSec On"=0, "Conn2/DIO_16_23 In"=[FALSE, FALSE, FALSE, FALSE, FALSE, FALSE, FALSE, FALSE], "Conn2/DIO_16_23 - uSec Off"=0}, "Conn2/DIO_24_31 In"={"Conn2/DIO_24_31 - 75kHz"=FALSE, "Conn2/DIO_24_31 - uSec On"=0, "Conn2/DIO_24_31 In"=[FALSE, FALSE, FALSE, FALSE, FALSE, FALSE, FALSE, FALSE], "Conn2/DIO_24_31 - uSec Off"=0}, "Conn2/DIO_32_39 In"={"Conn2/DIO_32_39 - 75kHz"=FALSE, "Conn2/DIO_32_39 - uSec On"=0, "Conn2/DIO_32_39 In"=[FALSE, FALSE, FALSE, FALSE, FALSE, FALSE, FALSE, FALSE], "Conn2/DIO_32_39 - uSec Off"=0}} ("Conn2 DIOs In"), "Conn2/DIO_0_7 In.Conn2/DIO_0_7 - 75kHz"=w1019, "Conn2/DIO_0_7 In.Conn2/DIO_0_7 - uSec On"=w1020, "Conn2/DIO_0_7 In.Conn2/DIO_0_7 In"=w963, "Conn2/DIO_0_7 In.Conn2/DIO_0_7 - uSec Off"=w1021, "Conn2/DIO_8_15 In.Conn2/DIO_8_15 - 75kHz"=w985, "Conn2/DIO_8_15 In.Conn2/DIO_8_15 - uSec On"=w984, "Conn2/DIO_8_15 In.Conn2/DIO_8_15 In"=w983, "Conn2/DIO_8_15 In.Conn2/DIO_8_15 - uSec Off"=w982, "Conn2/DIO_16_23 In.Conn2/DIO_16_23 - 75kHz"=w981, "Conn2/DIO_16_23 In.Conn2/DIO_16_23 - uSec On"=w980, "Conn2/DIO_16_23 In.Conn2/DIO_16_23 In"=w979, "Conn2/DIO_16_23 In.Conn2/DIO_16_23 - uSec Off"=w978, "Conn2/DIO_24_31 In.Conn2/DIO_24_31 - 75kHz"=w977, "Conn2/DIO_24_31 In.Conn2/DIO_24_31 - uSec On"=w976, "Conn2/DIO_24_31 In.Conn2/DIO_24_31 In"=w975, "Conn2/DIO_24_31 In.Conn2/DIO_24_31 - uSec Off"=w974, "Conn2/DIO_32_39 In.Conn2/DIO_32_39 - 75kHz"=w973, "Conn2/DIO_32_39 In.Conn2/DIO_32_39 - uSec On"=w972, "Conn2/DIO_32_39 In.Conn2/DIO_32_39 In"=w971, "Conn2/DIO_32_39 In.Conn2/DIO_32_39 - uSec Off"=w970) -> (w1031:T2)
        n82 = Build Array(w993, w992, w991, w990, w989, w988, w987, w986) -> (w1032:i16[])
        n83 = xnode "Read/Write Control"("FPGA VI Reference In"=w1014, "Conn0 DIOs In"=w1017, "Conn1 DIOs In"=w1030, "Conn2 DIOs In"=w1031, "Connector0/AO0_7"=w1032) -> ("FPGA VI Reference Out"=w1015:refnum<k20>)  [unwired: 1 in, 1 out]
      }
      frame "Triverse Power 5" {
        w1041 = FALSE  # Conn2/DIO_7
        w1040 = FALSE  # Conn2/DIO_6
        w1033 = FALSE  # Conn2/DIO_5
        w1034 = FALSE  # Conn2/DIO_4
        w1035 = TRUE  # Conn2/DIO_3
        w1039 = TRUE  # Conn2/DIO_2
        w1038 = FALSE  # Conn2/DIO_1
        w1037 = FALSE  # Conn2/DIO_0
        w1043 = u16 0  # Conn2/DIO_32_39 - uSec Off
        w1044 = bool[] [FALSE, FALSE, FALSE, FALSE, FALSE, FALSE, FALSE, FALSE]  # Conn2/DIO_32_39 In
        w1045 = u16 0  # Conn2/DIO_32_39 - uSec On
        w1046 = FALSE  # Conn2/DIO_32_39 - 75kHz
        w1047 = u16 0  # Conn2/DIO_24_31 - uSec Off
        w1048 = bool[] [FALSE, FALSE, FALSE, FALSE, FALSE, FALSE, FALSE, FALSE]  # Conn2/DIO_24_31 In
        w1049 = u16 0  # Conn2/DIO_24_31 - uSec On
        w1050 = FALSE  # Conn2/DIO_24_31 - 75kHz
        w1051 = u16 0  # Conn2/DIO_16_23 - uSec Off
        w1052 = bool[] [FALSE, FALSE, FALSE, FALSE, FALSE, FALSE, FALSE, FALSE]  # Conn2/DIO_16_23 In
        w1053 = u16 0  # Conn2/DIO_16_23 - uSec On
        w1054 = FALSE  # Conn2/DIO_16_23 - 75kHz
        w1055 = u16 6  # Conn2/DIO_8_15 - uSec Off
        w1056 = bool[] [FALSE, TRUE, FALSE, FALSE, FALSE, FALSE, FALSE, FALSE]  # Conn2/DIO_8_15 In
        w1057 = u16 7  # Conn2/DIO_8_15 - uSec On
        w1058 = TRUE  # Conn2/DIO_8_15 - 75kHz
        w1059 = i16 0  # Connector0/AO7
        w1060 = i16 0  # Connector0/AO6
        w1061 = i16 0  # Connector0/AO5
        w1062 = i16 0  # Connector0/AO4
        w1063 = i16 0  # Connector0/AO3
        w1064 = i16 0  # Connector0/AO2
        w1065 = i16 0  # Connector0/AO1
        w1066 = i16 0  # Connector0/AO0
        w1067 = u16 0  # Conn1/DIO_32_39 - uSec Off
        w1068 = bool[] [FALSE, FALSE, FALSE, FALSE, FALSE, FALSE, FALSE, FALSE]  # Conn1/DIO_32_39 In
        w1069 = u16 0  # Conn1/DIO_32_39 - uSec On
        w1070 = FALSE  # Conn1/DIO_32_39 - 75kHz
        w1071 = u16 0  # Conn1/DIO_24_31 - uSec Off
        w1072 = bool[] [FALSE, FALSE, FALSE, FALSE, FALSE, FALSE, FALSE, FALSE]  # Conn1/DIO_24_31 In
        w1073 = u16 0  # Conn1/DIO_24_31 - uSec On
        w1074 = FALSE  # Conn1/DIO_24_31 - 75kHz
        w1075 = u16 6  # Conn1/DIO_16_23 - uSec Off
        w1076 = bool[] [FALSE, TRUE, FALSE, FALSE, FALSE, FALSE, FALSE, FALSE]  # Conn1/DIO_16_23 In
        w1077 = u16 7  # Conn1/DIO_16_23 - uSec On
        w1078 = TRUE  # Conn1/DIO_16_23 - 75kHz
        w1079 = u16 6  # Conn1/DIO_8_15 - uSec Off
        w1080 = bool[] [FALSE, FALSE, FALSE, TRUE, FALSE, FALSE, FALSE, FALSE]  # Conn1/DIO_8_15 In
        w1081 = u16 7  # Conn1/DIO_8_15 - uSec On
        w1082 = TRUE  # Conn1/DIO_8_15 - 75kHz
        w1083 = u16 0  # Conn0/DIO_8_15 - uSec Off
        w1084 = bool[] [FALSE, FALSE, FALSE, FALSE, FALSE, FALSE, FALSE, FALSE]  # Conn0/DIO_8_15 In
        w1085 = u16 0  # Conn0/DIO_8_15 - uSec On
        w1086 = FALSE  # Conn0/DIO_8_15 - 75kHz
        w1102 = u16 0  # Conn0/DIO_0_7 - uSec Off
        w1101 = bool[] [FALSE, FALSE, FALSE, FALSE, FALSE, FALSE, FALSE, FALSE]  # Conn0/DIO_0_7 In
        w1100 = u16 0  # Conn0/DIO_0_7 - uSec On
        w1099 = FALSE  # Conn0/DIO_0_7 - 75kHz
        w1098 = u16 6  # Conn1/DIO_0_7 - uSec Off
        w1097 = bool[] [FALSE, TRUE, TRUE, TRUE, TRUE, FALSE, FALSE, TRUE]  # Conn1/DIO_0_7 In
        w1096 = u16 7  # Conn1/DIO_0_7 - uSec On
        w1095 = TRUE  # Conn1/DIO_0_7 - 75kHz
        w1094 = u16 6  # Conn2/DIO_0_7 - uSec Off
        w1093 = u16 7  # Conn2/DIO_0_7 - uSec On
        w1092 = TRUE  # Conn2/DIO_0_7 - 75kHz
        # "Triverse Power 5"
        # "Triverse Power 5"
        # "Triverse Power 5"
        n84 = Build Array(w1037, w1038, w1039, w1035, w1034, w1033, w1040, w1041) -> (w1036:bool[])
        n85 = Bundle By Name(cluster=T4 {"Conn0/DIO_0_7 In"={"Conn0/DIO_0_7 - 75kHz"=FALSE, "Conn0/DIO_0_7 - uSec On"=0, "Conn0/DIO_0_7 In"=[FALSE, FALSE, FALSE, FALSE, FALSE, FALSE, FALSE, FALSE], "Conn0/DIO_0_7 - uSec Off"=0}, "Conn0/DIO_8_15 In"={"Conn0/DIO_8_15 - 75kHz"=FALSE, "Conn0/DIO_8_15 - uSec On"=0, "Conn0/DIO_8_15 In"=[FALSE, FALSE, FALSE, FALSE, FALSE, FALSE, FALSE, FALSE], "Conn0/DIO_8_15 - uSec Off"=0}} ("Conn0 DIOs In"), "Conn0/DIO_0_7 In.Conn0/DIO_0_7 - 75kHz"=w1099, "Conn0/DIO_0_7 In.Conn0/DIO_0_7 - uSec On"=w1100, "Conn0/DIO_0_7 In.Conn0/DIO_0_7 In"=w1101, "Conn0/DIO_0_7 In.Conn0/DIO_0_7 - uSec Off"=w1102, "Conn0/DIO_8_15 In.Conn0/DIO_8_15 - 75kHz"=w1086, "Conn0/DIO_8_15 In.Conn0/DIO_8_15 - uSec On"=w1085, "Conn0/DIO_8_15 In.Conn0/DIO_8_15 In"=w1084, "Conn0/DIO_8_15 In.Conn0/DIO_8_15 - uSec Off"=w1083) -> (w1090:T4)
        n86 = Bundle By Name(cluster=T3 {"Conn1/DIO_0_7 In"={"Conn1/DIO_0_7 - 75kHz"=FALSE, "Conn1/DIO_0_7 - uSec On"=0, "Conn1/DIO_0_7 In"=[FALSE, FALSE, FALSE, FALSE, FALSE, FALSE, FALSE, FALSE], "Conn1/DIO_0_7 - uSec Off"=0}, "Conn1/DIO_8_15 In"={"Conn1/DIO_8_15 - 75kHz"=FALSE, "Conn1/DIO_8_15 - uSec On"=0, "Conn1/DIO_8_15 In"=[FALSE, FALSE, FALSE, FALSE, FALSE, FALSE, FALSE, FALSE], "Conn1/DIO_8_15 - uSec Off"=0}, "Conn1/DIO_16_23 In"={"Conn1/DIO_16_23 - 75kHz"=FALSE, "Conn1/DIO_16_23 - uSec On"=0, "Conn1/DIO_16_23 In"=[FALSE, FALSE, FALSE, FALSE, FALSE, FALSE, FALSE, FALSE], "Conn1/DIO_16_23 - uSec Off"=0}, "Conn1/DIO_24_31 In"={"Conn1/DIO_24_31 - 75kHz"=FALSE, "Conn1/DIO_24_31 - uSec On"=0, "Conn1/DIO_24_31 In"=[FALSE, FALSE, FALSE, FALSE, FALSE, FALSE, FALSE, FALSE], "Conn1/DIO_24_31 - uSec Off"=0}, "Conn1/DIO_32_39 In"={"Conn1/DIO_32_39 - 75kHz"=FALSE, "Conn1/DIO_32_39 - uSec On"=0, "Conn1/DIO_32_39 In"=[FALSE, FALSE, FALSE, FALSE, FALSE, FALSE, FALSE, FALSE], "Conn1/DIO_32_39 - uSec Off"=0}} ("Conn1 DIOs In"), "Conn1/DIO_0_7 In.Conn1/DIO_0_7 - 75kHz"=w1095, "Conn1/DIO_0_7 In.Conn1/DIO_0_7 - uSec On"=w1096, "Conn1/DIO_0_7 In.Conn1/DIO_0_7 In"=w1097, "Conn1/DIO_0_7 In.Conn1/DIO_0_7 - uSec Off"=w1098, "Conn1/DIO_8_15 In.Conn1/DIO_8_15 - 75kHz"=w1082, "Conn1/DIO_8_15 In.Conn1/DIO_8_15 - uSec On"=w1081, "Conn1/DIO_8_15 In.Conn1/DIO_8_15 In"=w1080, "Conn1/DIO_8_15 In.Conn1/DIO_8_15 - uSec Off"=w1079, "Conn1/DIO_16_23 In.Conn1/DIO_16_23 - 75kHz"=w1078, "Conn1/DIO_16_23 In.Conn1/DIO_16_23 - uSec On"=w1077, "Conn1/DIO_16_23 In.Conn1/DIO_16_23 In"=w1076, "Conn1/DIO_16_23 In.Conn1/DIO_16_23 - uSec Off"=w1075, "Conn1/DIO_24_31 In.Conn1/DIO_24_31 - 75kHz"=w1074, "Conn1/DIO_24_31 In.Conn1/DIO_24_31 - uSec On"=w1073, "Conn1/DIO_24_31 In.Conn1/DIO_24_31 In"=w1072, "Conn1/DIO_24_31 In.Conn1/DIO_24_31 - uSec Off"=w1071, "Conn1/DIO_32_39 In.Conn1/DIO_32_39 - 75kHz"=w1070, "Conn1/DIO_32_39 In.Conn1/DIO_32_39 - uSec On"=w1069, "Conn1/DIO_32_39 In.Conn1/DIO_32_39 In"=w1068, "Conn1/DIO_32_39 In.Conn1/DIO_32_39 - uSec Off"=w1067) -> (w1103:T3)
        n87 = Bundle By Name(cluster=T2 {"Conn2/DIO_0_7 In"={"Conn2/DIO_0_7 - 75kHz"=FALSE, "Conn2/DIO_0_7 - uSec On"=0, "Conn2/DIO_0_7 In"=[FALSE, FALSE, FALSE, FALSE, FALSE, FALSE, FALSE, FALSE], "Conn2/DIO_0_7 - uSec Off"=0}, "Conn2/DIO_8_15 In"={"Conn2/DIO_8_15 - 75kHz"=FALSE, "Conn2/DIO_8_15 - uSec On"=0, "Conn2/DIO_8_15 In"=[FALSE, FALSE, FALSE, FALSE, FALSE, FALSE, FALSE, FALSE], "Conn2/DIO_8_15 - uSec Off"=0}, "Conn2/DIO_16_23 In"={"Conn2/DIO_16_23 - 75kHz"=FALSE, "Conn2/DIO_16_23 - uSec On"=0, "Conn2/DIO_16_23 In"=[FALSE, FALSE, FALSE, FALSE, FALSE, FALSE, FALSE, FALSE], "Conn2/DIO_16_23 - uSec Off"=0}, "Conn2/DIO_24_31 In"={"Conn2/DIO_24_31 - 75kHz"=FALSE, "Conn2/DIO_24_31 - uSec On"=0, "Conn2/DIO_24_31 In"=[FALSE, FALSE, FALSE, FALSE, FALSE, FALSE, FALSE, FALSE], "Conn2/DIO_24_31 - uSec Off"=0}, "Conn2/DIO_32_39 In"={"Conn2/DIO_32_39 - 75kHz"=FALSE, "Conn2/DIO_32_39 - uSec On"=0, "Conn2/DIO_32_39 In"=[FALSE, FALSE, FALSE, FALSE, FALSE, FALSE, FALSE, FALSE], "Conn2/DIO_32_39 - uSec Off"=0}} ("Conn2 DIOs In"), "Conn2/DIO_0_7 In.Conn2/DIO_0_7 - 75kHz"=w1092, "Conn2/DIO_0_7 In.Conn2/DIO_0_7 - uSec On"=w1093, "Conn2/DIO_0_7 In.Conn2/DIO_0_7 In"=w1036, "Conn2/DIO_0_7 In.Conn2/DIO_0_7 - uSec Off"=w1094, "Conn2/DIO_8_15 In.Conn2/DIO_8_15 - 75kHz"=w1058, "Conn2/DIO_8_15 In.Conn2/DIO_8_15 - uSec On"=w1057, "Conn2/DIO_8_15 In.Conn2/DIO_8_15 In"=w1056, "Conn2/DIO_8_15 In.Conn2/DIO_8_15 - uSec Off"=w1055, "Conn2/DIO_16_23 In.Conn2/DIO_16_23 - 75kHz"=w1054, "Conn2/DIO_16_23 In.Conn2/DIO_16_23 - uSec On"=w1053, "Conn2/DIO_16_23 In.Conn2/DIO_16_23 In"=w1052, "Conn2/DIO_16_23 In.Conn2/DIO_16_23 - uSec Off"=w1051, "Conn2/DIO_24_31 In.Conn2/DIO_24_31 - 75kHz"=w1050, "Conn2/DIO_24_31 In.Conn2/DIO_24_31 - uSec On"=w1049, "Conn2/DIO_24_31 In.Conn2/DIO_24_31 In"=w1048, "Conn2/DIO_24_31 In.Conn2/DIO_24_31 - uSec Off"=w1047, "Conn2/DIO_32_39 In.Conn2/DIO_32_39 - 75kHz"=w1046, "Conn2/DIO_32_39 In.Conn2/DIO_32_39 - uSec On"=w1045, "Conn2/DIO_32_39 In.Conn2/DIO_32_39 In"=w1044, "Conn2/DIO_32_39 In.Conn2/DIO_32_39 - uSec Off"=w1043) -> (w1104:T2)
        n88 = Build Array(w1066, w1065, w1064, w1063, w1062, w1061, w1060, w1059) -> (w1105:i16[])
        n89 = xnode "Read/Write Control"("FPGA VI Reference In"=w1087, "Conn0 DIOs In"=w1090, "Conn1 DIOs In"=w1103, "Conn2 DIOs In"=w1104, "Connector0/AO0_7"=w1105) -> ("FPGA VI Reference Out"=w1088:refnum<k20>)  [unwired: 1 in, 1 out]
      }
      frame "Handswitch - Triverse Seal" {
        w1114 = TRUE  # Conn2/DIO_7
        w1113 = FALSE  # Conn2/DIO_6
        w1112 = TRUE  # Conn2/DIO_2
        w1111 = FALSE  # Conn2/DIO_1
        w1110 = FALSE  # Conn2/DIO_0
        w1116 = u16 0  # Conn2/DIO_32_39 - uSec Off
        w1117 = bool[] [FALSE, FALSE, FALSE, FALSE, FALSE, FALSE, FALSE, FALSE]  # Conn2/DIO_32_39 In
        w1118 = u16 0  # Conn2/DIO_32_39 - uSec On
        w1119 = FALSE  # Conn2/DIO_32_39 - 75kHz
        w1120 = u16 0  # Conn2/DIO_24_31 - uSec Off
        w1121 = bool[] [FALSE, FALSE, FALSE, FALSE, FALSE, FALSE, FALSE, FALSE]  # Conn2/DIO_24_31 In
        w1122 = u16 0  # Conn2/DIO_24_31 - uSec On
        w1123 = FALSE  # Conn2/DIO_24_31 - 75kHz
        w1124 = u16 0  # Conn2/DIO_16_23 - uSec Off
        w1125 = bool[] [FALSE, FALSE, FALSE, FALSE, FALSE, FALSE, FALSE, FALSE]  # Conn2/DIO_16_23 In
        w1126 = u16 0  # Conn2/DIO_16_23 - uSec On
        w1127 = FALSE  # Conn2/DIO_16_23 - 75kHz
        w1128 = u16 6  # Conn2/DIO_8_15 - uSec Off
        w1129 = bool[] [FALSE, FALSE, TRUE, FALSE, FALSE, FALSE, FALSE, FALSE]  # Conn2/DIO_8_15 In
        w1130 = u16 7  # Conn2/DIO_8_15 - uSec On
        w1131 = TRUE  # Conn2/DIO_8_15 - 75kHz
        w1132 = i16 0  # Connector0/AO7
        w1133 = i16 0  # Connector0/AO6
        w1134 = i16 0  # Connector0/AO5
        w1135 = i16 0  # Connector0/AO4
        w1136 = i16 0  # Connector0/AO3
        w1137 = i16 0  # Connector0/AO2
        w1138 = i16 0  # Connector0/AO1
        w1139 = i16 0  # Connector0/AO0
        w1140 = u16 0  # Conn1/DIO_32_39 - uSec Off
        w1141 = bool[] [FALSE, FALSE, FALSE, FALSE, FALSE, FALSE, FALSE, FALSE]  # Conn1/DIO_32_39 In
        w1142 = u16 0  # Conn1/DIO_32_39 - uSec On
        w1143 = FALSE  # Conn1/DIO_32_39 - 75kHz
        w1144 = u16 0  # Conn1/DIO_24_31 - uSec Off
        w1145 = bool[] [FALSE, FALSE, FALSE, FALSE, FALSE, FALSE, FALSE, FALSE]  # Conn1/DIO_24_31 In
        w1146 = u16 0  # Conn1/DIO_24_31 - uSec On
        w1147 = FALSE  # Conn1/DIO_24_31 - 75kHz
        w1148 = u16 6  # Conn1/DIO_16_23 - uSec Off
        w1149 = bool[] [FALSE, TRUE, FALSE, FALSE, FALSE, FALSE, FALSE, FALSE]  # Conn1/DIO_16_23 In
        w1150 = u16 7  # Conn1/DIO_16_23 - uSec On
        w1151 = TRUE  # Conn1/DIO_16_23 - 75kHz
        w1152 = u16 6  # Conn1/DIO_8_15 - uSec Off
        w1153 = bool[] [FALSE, FALSE, FALSE, TRUE, FALSE, FALSE, FALSE, FALSE]  # Conn1/DIO_8_15 In
        w1154 = u16 7  # Conn1/DIO_8_15 - uSec On
        w1155 = TRUE  # Conn1/DIO_8_15 - 75kHz
        w1156 = u16 0  # Conn0/DIO_8_15 - uSec Off
        w1157 = bool[] [FALSE, FALSE, FALSE, FALSE, FALSE, FALSE, FALSE, FALSE]  # Conn0/DIO_8_15 In
        w1158 = u16 0  # Conn0/DIO_8_15 - uSec On
        w1159 = FALSE  # Conn0/DIO_8_15 - 75kHz
        w1175 = u16 0  # Conn0/DIO_0_7 - uSec Off
        w1174 = bool[] [FALSE, FALSE, FALSE, FALSE, FALSE, FALSE, FALSE, FALSE]  # Conn0/DIO_0_7 In
        w1173 = u16 0  # Conn0/DIO_0_7 - uSec On
        w1172 = FALSE  # Conn0/DIO_0_7 - 75kHz
        w1171 = u16 6  # Conn1/DIO_0_7 - uSec Off
        w1170 = bool[] [FALSE, TRUE, TRUE, TRUE, TRUE, FALSE, FALSE, TRUE]  # Conn1/DIO_0_7 In
        w1169 = u16 7  # Conn1/DIO_0_7 - uSec On
        w1168 = TRUE  # Conn1/DIO_0_7 - 75kHz
        w1167 = u16 6  # Conn2/DIO_0_7 - uSec Off
        w1166 = u16 7  # Conn2/DIO_0_7 - uSec On
        w1165 = TRUE  # Conn2/DIO_0_7 - 75kHz
        # "Handswitch - Triverse Seal"
        # "Handswitch - Triverse Seal"
        # "Handswitch - Triverse Seal"
        n90 = Build Array(w1110, w1111, w1112, w1108, w1107, w1106, w1113, w1114) -> (w1109:bool[])
        n91 = Bundle By Name(cluster=T4 {"Conn0/DIO_0_7 In"={"Conn0/DIO_0_7 - 75kHz"=FALSE, "Conn0/DIO_0_7 - uSec On"=0, "Conn0/DIO_0_7 In"=[FALSE, FALSE, FALSE, FALSE, FALSE, FALSE, FALSE, FALSE], "Conn0/DIO_0_7 - uSec Off"=0}, "Conn0/DIO_8_15 In"={"Conn0/DIO_8_15 - 75kHz"=FALSE, "Conn0/DIO_8_15 - uSec On"=0, "Conn0/DIO_8_15 In"=[FALSE, FALSE, FALSE, FALSE, FALSE, FALSE, FALSE, FALSE], "Conn0/DIO_8_15 - uSec Off"=0}} ("Conn0 DIOs In"), "Conn0/DIO_0_7 In.Conn0/DIO_0_7 - 75kHz"=w1172, "Conn0/DIO_0_7 In.Conn0/DIO_0_7 - uSec On"=w1173, "Conn0/DIO_0_7 In.Conn0/DIO_0_7 In"=w1174, "Conn0/DIO_0_7 In.Conn0/DIO_0_7 - uSec Off"=w1175, "Conn0/DIO_8_15 In.Conn0/DIO_8_15 - 75kHz"=w1159, "Conn0/DIO_8_15 In.Conn0/DIO_8_15 - uSec On"=w1158, "Conn0/DIO_8_15 In.Conn0/DIO_8_15 In"=w1157, "Conn0/DIO_8_15 In.Conn0/DIO_8_15 - uSec Off"=w1156) -> (w1163:T4)
        n92 = Bundle By Name(cluster=T3 {"Conn1/DIO_0_7 In"={"Conn1/DIO_0_7 - 75kHz"=FALSE, "Conn1/DIO_0_7 - uSec On"=0, "Conn1/DIO_0_7 In"=[FALSE, FALSE, FALSE, FALSE, FALSE, FALSE, FALSE, FALSE], "Conn1/DIO_0_7 - uSec Off"=0}, "Conn1/DIO_8_15 In"={"Conn1/DIO_8_15 - 75kHz"=FALSE, "Conn1/DIO_8_15 - uSec On"=0, "Conn1/DIO_8_15 In"=[FALSE, FALSE, FALSE, FALSE, FALSE, FALSE, FALSE, FALSE], "Conn1/DIO_8_15 - uSec Off"=0}, "Conn1/DIO_16_23 In"={"Conn1/DIO_16_23 - 75kHz"=FALSE, "Conn1/DIO_16_23 - uSec On"=0, "Conn1/DIO_16_23 In"=[FALSE, FALSE, FALSE, FALSE, FALSE, FALSE, FALSE, FALSE], "Conn1/DIO_16_23 - uSec Off"=0}, "Conn1/DIO_24_31 In"={"Conn1/DIO_24_31 - 75kHz"=FALSE, "Conn1/DIO_24_31 - uSec On"=0, "Conn1/DIO_24_31 In"=[FALSE, FALSE, FALSE, FALSE, FALSE, FALSE, FALSE, FALSE], "Conn1/DIO_24_31 - uSec Off"=0}, "Conn1/DIO_32_39 In"={"Conn1/DIO_32_39 - 75kHz"=FALSE, "Conn1/DIO_32_39 - uSec On"=0, "Conn1/DIO_32_39 In"=[FALSE, FALSE, FALSE, FALSE, FALSE, FALSE, FALSE, FALSE], "Conn1/DIO_32_39 - uSec Off"=0}} ("Conn1 DIOs In"), "Conn1/DIO_0_7 In.Conn1/DIO_0_7 - 75kHz"=w1168, "Conn1/DIO_0_7 In.Conn1/DIO_0_7 - uSec On"=w1169, "Conn1/DIO_0_7 In.Conn1/DIO_0_7 In"=w1170, "Conn1/DIO_0_7 In.Conn1/DIO_0_7 - uSec Off"=w1171, "Conn1/DIO_8_15 In.Conn1/DIO_8_15 - 75kHz"=w1155, "Conn1/DIO_8_15 In.Conn1/DIO_8_15 - uSec On"=w1154, "Conn1/DIO_8_15 In.Conn1/DIO_8_15 In"=w1153, "Conn1/DIO_8_15 In.Conn1/DIO_8_15 - uSec Off"=w1152, "Conn1/DIO_16_23 In.Conn1/DIO_16_23 - 75kHz"=w1151, "Conn1/DIO_16_23 In.Conn1/DIO_16_23 - uSec On"=w1150, "Conn1/DIO_16_23 In.Conn1/DIO_16_23 In"=w1149, "Conn1/DIO_16_23 In.Conn1/DIO_16_23 - uSec Off"=w1148, "Conn1/DIO_24_31 In.Conn1/DIO_24_31 - 75kHz"=w1147, "Conn1/DIO_24_31 In.Conn1/DIO_24_31 - uSec On"=w1146, "Conn1/DIO_24_31 In.Conn1/DIO_24_31 In"=w1145, "Conn1/DIO_24_31 In.Conn1/DIO_24_31 - uSec Off"=w1144, "Conn1/DIO_32_39 In.Conn1/DIO_32_39 - 75kHz"=w1143, "Conn1/DIO_32_39 In.Conn1/DIO_32_39 - uSec On"=w1142, "Conn1/DIO_32_39 In.Conn1/DIO_32_39 In"=w1141, "Conn1/DIO_32_39 In.Conn1/DIO_32_39 - uSec Off"=w1140) -> (w1176:T3)
        n93 = Bundle By Name(cluster=T2 {"Conn2/DIO_0_7 In"={"Conn2/DIO_0_7 - 75kHz"=FALSE, "Conn2/DIO_0_7 - uSec On"=0, "Conn2/DIO_0_7 In"=[FALSE, FALSE, FALSE, FALSE, FALSE, FALSE, FALSE, FALSE], "Conn2/DIO_0_7 - uSec Off"=0}, "Conn2/DIO_8_15 In"={"Conn2/DIO_8_15 - 75kHz"=FALSE, "Conn2/DIO_8_15 - uSec On"=0, "Conn2/DIO_8_15 In"=[FALSE, FALSE, FALSE, FALSE, FALSE, FALSE, FALSE, FALSE], "Conn2/DIO_8_15 - uSec Off"=0}, "Conn2/DIO_16_23 In"={"Conn2/DIO_16_23 - 75kHz"=FALSE, "Conn2/DIO_16_23 - uSec On"=0, "Conn2/DIO_16_23 In"=[FALSE, FALSE, FALSE, FALSE, FALSE, FALSE, FALSE, FALSE], "Conn2/DIO_16_23 - uSec Off"=0}, "Conn2/DIO_24_31 In"={"Conn2/DIO_24_31 - 75kHz"=FALSE, "Conn2/DIO_24_31 - uSec On"=0, "Conn2/DIO_24_31 In"=[FALSE, FALSE, FALSE, FALSE, FALSE, FALSE, FALSE, FALSE], "Conn2/DIO_24_31 - uSec Off"=0}, "Conn2/DIO_32_39 In"={"Conn2/DIO_32_39 - 75kHz"=FALSE, "Conn2/DIO_32_39 - uSec On"=0, "Conn2/DIO_32_39 In"=[FALSE, FALSE, FALSE, FALSE, FALSE, FALSE, FALSE, FALSE], "Conn2/DIO_32_39 - uSec Off"=0}} ("Conn2 DIOs In"), "Conn2/DIO_0_7 In.Conn2/DIO_0_7 - 75kHz"=w1165, "Conn2/DIO_0_7 In.Conn2/DIO_0_7 - uSec On"=w1166, "Conn2/DIO_0_7 In.Conn2/DIO_0_7 In"=w1109, "Conn2/DIO_0_7 In.Conn2/DIO_0_7 - uSec Off"=w1167, "Conn2/DIO_8_15 In.Conn2/DIO_8_15 - 75kHz"=w1131, "Conn2/DIO_8_15 In.Conn2/DIO_8_15 - uSec On"=w1130, "Conn2/DIO_8_15 In.Conn2/DIO_8_15 In"=w1129, "Conn2/DIO_8_15 In.Conn2/DIO_8_15 - uSec Off"=w1128, "Conn2/DIO_16_23 In.Conn2/DIO_16_23 - 75kHz"=w1127, "Conn2/DIO_16_23 In.Conn2/DIO_16_23 - uSec On"=w1126, "Conn2/DIO_16_23 In.Conn2/DIO_16_23 In"=w1125, "Conn2/DIO_16_23 In.Conn2/DIO_16_23 - uSec Off"=w1124, "Conn2/DIO_24_31 In.Conn2/DIO_24_31 - 75kHz"=w1123, "Conn2/DIO_24_31 In.Conn2/DIO_24_31 - uSec On"=w1122, "Conn2/DIO_24_31 In.Conn2/DIO_24_31 In"=w1121, "Conn2/DIO_24_31 In.Conn2/DIO_24_31 - uSec Off"=w1120, "Conn2/DIO_32_39 In.Conn2/DIO_32_39 - 75kHz"=w1119, "Conn2/DIO_32_39 In.Conn2/DIO_32_39 - uSec On"=w1118, "Conn2/DIO_32_39 In.Conn2/DIO_32_39 In"=w1117, "Conn2/DIO_32_39 In.Conn2/DIO_32_39 - uSec Off"=w1116) -> (w1177:T2)
        n94 = Build Array(w1139, w1138, w1137, w1136, w1135, w1134, w1133, w1132) -> (w1178:i16[])
        n95 = xnode "Read/Write Control"("FPGA VI Reference In"=w1160, "Conn0 DIOs In"=w1163, "Conn1 DIOs In"=w1176, "Conn2 DIOs In"=w1177, "Connector0/AO0_7"=w1178) -> ("FPGA VI Reference Out"=w1161:refnum<k20>)  [unwired: 1 in, 1 out]
      }
      frame "Handswitch - Triverse Cut" {
        w1187 = FALSE  # Conn2/DIO_7
        w1186 = TRUE  # Conn2/DIO_6
        w1185 = TRUE  # Conn2/DIO_2
        w1184 = FALSE  # Conn2/DIO_1
        w1183 = FALSE  # Conn2/DIO_0
        w1189 = u16 0  # Conn2/DIO_32_39 - uSec Off
        w1190 = bool[] [FALSE, FALSE, FALSE, FALSE, FALSE, FALSE, FALSE, FALSE]  # Conn2/DIO_32_39 In
        w1191 = u16 0  # Conn2/DIO_32_39 - uSec On
        w1192 = FALSE  # Conn2/DIO_32_39 - 75kHz
        w1193 = u16 0  # Conn2/DIO_24_31 - uSec Off
        w1194 = bool[] [FALSE, FALSE, FALSE, FALSE, FALSE, FALSE, FALSE, FALSE]  # Conn2/DIO_24_31 In
        w1195 = u16 0  # Conn2/DIO_24_31 - uSec On
        w1196 = FALSE  # Conn2/DIO_24_31 - 75kHz
        w1197 = u16 0  # Conn2/DIO_16_23 - uSec Off
        w1198 = bool[] [FALSE, FALSE, FALSE, FALSE, FALSE, FALSE, FALSE, FALSE]  # Conn2/DIO_16_23 In
        w1199 = u16 0  # Conn2/DIO_16_23 - uSec On
        w1200 = FALSE  # Conn2/DIO_16_23 - 75kHz
        w1201 = u16 6  # Conn2/DIO_8_15 - uSec Off
        w1202 = bool[] [FALSE, FALSE, TRUE, FALSE, FALSE, FALSE, FALSE, FALSE]  # Conn2/DIO_8_15 In
        w1203 = u16 7  # Conn2/DIO_8_15 - uSec On
        w1204 = TRUE  # Conn2/DIO_8_15 - 75kHz
        w1205 = i16 0  # Connector0/AO7
        w1206 = i16 0  # Connector0/AO6
        w1207 = i16 0  # Connector0/AO5
        w1208 = i16 0  # Connector0/AO4
        w1209 = i16 0  # Connector0/AO3
        w1210 = i16 0  # Connector0/AO2
        w1211 = i16 0  # Connector0/AO1
        w1212 = i16 0  # Connector0/AO0
        w1213 = u16 0  # Conn1/DIO_32_39 - uSec Off
        w1214 = bool[] [FALSE, FALSE, FALSE, FALSE, FALSE, FALSE, FALSE, FALSE]  # Conn1/DIO_32_39 In
        w1215 = u16 0  # Conn1/DIO_32_39 - uSec On
        w1216 = FALSE  # Conn1/DIO_32_39 - 75kHz
        w1217 = u16 0  # Conn1/DIO_24_31 - uSec Off
        w1218 = bool[] [FALSE, FALSE, FALSE, FALSE, FALSE, FALSE, FALSE, FALSE]  # Conn1/DIO_24_31 In
        w1219 = u16 0  # Conn1/DIO_24_31 - uSec On
        w1220 = FALSE  # Conn1/DIO_24_31 - 75kHz
        w1221 = u16 6  # Conn1/DIO_16_23 - uSec Off
        w1222 = bool[] [FALSE, TRUE, FALSE, FALSE, FALSE, FALSE, FALSE, FALSE]  # Conn1/DIO_16_23 In
        w1223 = u16 7  # Conn1/DIO_16_23 - uSec On
        w1224 = TRUE  # Conn1/DIO_16_23 - 75kHz
        w1225 = u16 6  # Conn1/DIO_8_15 - uSec Off
        w1226 = bool[] [FALSE, FALSE, FALSE, TRUE, FALSE, FALSE, FALSE, FALSE]  # Conn1/DIO_8_15 In
        w1227 = u16 7  # Conn1/DIO_8_15 - uSec On
        w1228 = TRUE  # Conn1/DIO_8_15 - 75kHz
        w1229 = u16 0  # Conn0/DIO_8_15 - uSec Off
        w1230 = bool[] [FALSE, FALSE, FALSE, FALSE, FALSE, FALSE, FALSE, FALSE]  # Conn0/DIO_8_15 In
        w1231 = u16 0  # Conn0/DIO_8_15 - uSec On
        w1232 = FALSE  # Conn0/DIO_8_15 - 75kHz
        w1248 = u16 0  # Conn0/DIO_0_7 - uSec Off
        w1247 = bool[] [FALSE, FALSE, FALSE, FALSE, FALSE, FALSE, FALSE, FALSE]  # Conn0/DIO_0_7 In
        w1246 = u16 0  # Conn0/DIO_0_7 - uSec On
        w1245 = FALSE  # Conn0/DIO_0_7 - 75kHz
        w1244 = u16 6  # Conn1/DIO_0_7 - uSec Off
        w1243 = bool[] [FALSE, TRUE, TRUE, TRUE, TRUE, FALSE, FALSE, TRUE]  # Conn1/DIO_0_7 In
        w1242 = u16 7  # Conn1/DIO_0_7 - uSec On
        w1241 = TRUE  # Conn1/DIO_0_7 - 75kHz
        w1240 = u16 6  # Conn2/DIO_0_7 - uSec Off
        w1239 = u16 7  # Conn2/DIO_0_7 - uSec On
        w1238 = TRUE  # Conn2/DIO_0_7 - 75kHz
        # "Handswitch - Triverse Cut"
        # "Handswitch - Triverse Cut"
        # "Handswitch - Triverse Cut"
        n96 = Build Array(w1183, w1184, w1185, w1181, w1180, w1179, w1186, w1187) -> (w1182:bool[])
        n97 = Bundle By Name(cluster=T4 {"Conn0/DIO_0_7 In"={"Conn0/DIO_0_7 - 75kHz"=FALSE, "Conn0/DIO_0_7 - uSec On"=0, "Conn0/DIO_0_7 In"=[FALSE, FALSE, FALSE, FALSE, FALSE, FALSE, FALSE, FALSE], "Conn0/DIO_0_7 - uSec Off"=0}, "Conn0/DIO_8_15 In"={"Conn0/DIO_8_15 - 75kHz"=FALSE, "Conn0/DIO_8_15 - uSec On"=0, "Conn0/DIO_8_15 In"=[FALSE, FALSE, FALSE, FALSE, FALSE, FALSE, FALSE, FALSE], "Conn0/DIO_8_15 - uSec Off"=0}} ("Conn0 DIOs In"), "Conn0/DIO_0_7 In.Conn0/DIO_0_7 - 75kHz"=w1245, "Conn0/DIO_0_7 In.Conn0/DIO_0_7 - uSec On"=w1246, "Conn0/DIO_0_7 In.Conn0/DIO_0_7 In"=w1247, "Conn0/DIO_0_7 In.Conn0/DIO_0_7 - uSec Off"=w1248, "Conn0/DIO_8_15 In.Conn0/DIO_8_15 - 75kHz"=w1232, "Conn0/DIO_8_15 In.Conn0/DIO_8_15 - uSec On"=w1231, "Conn0/DIO_8_15 In.Conn0/DIO_8_15 In"=w1230, "Conn0/DIO_8_15 In.Conn0/DIO_8_15 - uSec Off"=w1229) -> (w1236:T4)
        n98 = Bundle By Name(cluster=T3 {"Conn1/DIO_0_7 In"={"Conn1/DIO_0_7 - 75kHz"=FALSE, "Conn1/DIO_0_7 - uSec On"=0, "Conn1/DIO_0_7 In"=[FALSE, FALSE, FALSE, FALSE, FALSE, FALSE, FALSE, FALSE], "Conn1/DIO_0_7 - uSec Off"=0}, "Conn1/DIO_8_15 In"={"Conn1/DIO_8_15 - 75kHz"=FALSE, "Conn1/DIO_8_15 - uSec On"=0, "Conn1/DIO_8_15 In"=[FALSE, FALSE, FALSE, FALSE, FALSE, FALSE, FALSE, FALSE], "Conn1/DIO_8_15 - uSec Off"=0}, "Conn1/DIO_16_23 In"={"Conn1/DIO_16_23 - 75kHz"=FALSE, "Conn1/DIO_16_23 - uSec On"=0, "Conn1/DIO_16_23 In"=[FALSE, FALSE, FALSE, FALSE, FALSE, FALSE, FALSE, FALSE], "Conn1/DIO_16_23 - uSec Off"=0}, "Conn1/DIO_24_31 In"={"Conn1/DIO_24_31 - 75kHz"=FALSE, "Conn1/DIO_24_31 - uSec On"=0, "Conn1/DIO_24_31 In"=[FALSE, FALSE, FALSE, FALSE, FALSE, FALSE, FALSE, FALSE], "Conn1/DIO_24_31 - uSec Off"=0}, "Conn1/DIO_32_39 In"={"Conn1/DIO_32_39 - 75kHz"=FALSE, "Conn1/DIO_32_39 - uSec On"=0, "Conn1/DIO_32_39 In"=[FALSE, FALSE, FALSE, FALSE, FALSE, FALSE, FALSE, FALSE], "Conn1/DIO_32_39 - uSec Off"=0}} ("Conn1 DIOs In"), "Conn1/DIO_0_7 In.Conn1/DIO_0_7 - 75kHz"=w1241, "Conn1/DIO_0_7 In.Conn1/DIO_0_7 - uSec On"=w1242, "Conn1/DIO_0_7 In.Conn1/DIO_0_7 In"=w1243, "Conn1/DIO_0_7 In.Conn1/DIO_0_7 - uSec Off"=w1244, "Conn1/DIO_8_15 In.Conn1/DIO_8_15 - 75kHz"=w1228, "Conn1/DIO_8_15 In.Conn1/DIO_8_15 - uSec On"=w1227, "Conn1/DIO_8_15 In.Conn1/DIO_8_15 In"=w1226, "Conn1/DIO_8_15 In.Conn1/DIO_8_15 - uSec Off"=w1225, "Conn1/DIO_16_23 In.Conn1/DIO_16_23 - 75kHz"=w1224, "Conn1/DIO_16_23 In.Conn1/DIO_16_23 - uSec On"=w1223, "Conn1/DIO_16_23 In.Conn1/DIO_16_23 In"=w1222, "Conn1/DIO_16_23 In.Conn1/DIO_16_23 - uSec Off"=w1221, "Conn1/DIO_24_31 In.Conn1/DIO_24_31 - 75kHz"=w1220, "Conn1/DIO_24_31 In.Conn1/DIO_24_31 - uSec On"=w1219, "Conn1/DIO_24_31 In.Conn1/DIO_24_31 In"=w1218, "Conn1/DIO_24_31 In.Conn1/DIO_24_31 - uSec Off"=w1217, "Conn1/DIO_32_39 In.Conn1/DIO_32_39 - 75kHz"=w1216, "Conn1/DIO_32_39 In.Conn1/DIO_32_39 - uSec On"=w1215, "Conn1/DIO_32_39 In.Conn1/DIO_32_39 In"=w1214, "Conn1/DIO_32_39 In.Conn1/DIO_32_39 - uSec Off"=w1213) -> (w1249:T3)
        n99 = Bundle By Name(cluster=T2 {"Conn2/DIO_0_7 In"={"Conn2/DIO_0_7 - 75kHz"=FALSE, "Conn2/DIO_0_7 - uSec On"=0, "Conn2/DIO_0_7 In"=[FALSE, FALSE, FALSE, FALSE, FALSE, FALSE, FALSE, FALSE], "Conn2/DIO_0_7 - uSec Off"=0}, "Conn2/DIO_8_15 In"={"Conn2/DIO_8_15 - 75kHz"=FALSE, "Conn2/DIO_8_15 - uSec On"=0, "Conn2/DIO_8_15 In"=[FALSE, FALSE, FALSE, FALSE, FALSE, FALSE, FALSE, FALSE], "Conn2/DIO_8_15 - uSec Off"=0}, "Conn2/DIO_16_23 In"={"Conn2/DIO_16_23 - 75kHz"=FALSE, "Conn2/DIO_16_23 - uSec On"=0, "Conn2/DIO_16_23 In"=[FALSE, FALSE, FALSE, FALSE, FALSE, FALSE, FALSE, FALSE], "Conn2/DIO_16_23 - uSec Off"=0}, "Conn2/DIO_24_31 In"={"Conn2/DIO_24_31 - 75kHz"=FALSE, "Conn2/DIO_24_31 - uSec On"=0, "Conn2/DIO_24_31 In"=[FALSE, FALSE, FALSE, FALSE, FALSE, FALSE, FALSE, FALSE], "Conn2/DIO_24_31 - uSec Off"=0}, "Conn2/DIO_32_39 In"={"Conn2/DIO_32_39 - 75kHz"=FALSE, "Conn2/DIO_32_39 - uSec On"=0, "Conn2/DIO_32_39 In"=[FALSE, FALSE, FALSE, FALSE, FALSE, FALSE, FALSE, FALSE], "Conn2/DIO_32_39 - uSec Off"=0}} ("Conn2 DIOs In"), "Conn2/DIO_0_7 In.Conn2/DIO_0_7 - 75kHz"=w1238, "Conn2/DIO_0_7 In.Conn2/DIO_0_7 - uSec On"=w1239, "Conn2/DIO_0_7 In.Conn2/DIO_0_7 In"=w1182, "Conn2/DIO_0_7 In.Conn2/DIO_0_7 - uSec Off"=w1240, "Conn2/DIO_8_15 In.Conn2/DIO_8_15 - 75kHz"=w1204, "Conn2/DIO_8_15 In.Conn2/DIO_8_15 - uSec On"=w1203, "Conn2/DIO_8_15 In.Conn2/DIO_8_15 In"=w1202, "Conn2/DIO_8_15 In.Conn2/DIO_8_15 - uSec Off"=w1201, "Conn2/DIO_16_23 In.Conn2/DIO_16_23 - 75kHz"=w1200, "Conn2/DIO_16_23 In.Conn2/DIO_16_23 - uSec On"=w1199, "Conn2/DIO_16_23 In.Conn2/DIO_16_23 In"=w1198, "Conn2/DIO_16_23 In.Conn2/DIO_16_23 - uSec Off"=w1197, "Conn2/DIO_24_31 In.Conn2/DIO_24_31 - 75kHz"=w1196, "Conn2/DIO_24_31 In.Conn2/DIO_24_31 - uSec On"=w1195, "Conn2/DIO_24_31 In.Conn2/DIO_24_31 In"=w1194, "Conn2/DIO_24_31 In.Conn2/DIO_24_31 - uSec Off"=w1193, "Conn2/DIO_32_39 In.Conn2/DIO_32_39 - 75kHz"=w1192, "Conn2/DIO_32_39 In.Conn2/DIO_32_39 - uSec On"=w1191, "Conn2/DIO_32_39 In.Conn2/DIO_32_39 In"=w1190, "Conn2/DIO_32_39 In.Conn2/DIO_32_39 - uSec Off"=w1189) -> (w1250:T2)
        n100 = Build Array(w1212, w1211, w1210, w1209, w1208, w1207, w1206, w1205) -> (w1251:i16[])
        n101 = xnode "Read/Write Control"("FPGA VI Reference In"=w1233, "Conn0 DIOs In"=w1236, "Conn1 DIOs In"=w1249, "Conn2 DIOs In"=w1250, "Connector0/AO0_7"=w1251) -> ("FPGA VI Reference Out"=w1234:refnum<k20>)  [unwired: 1 in, 1 out]
      }
      frame "Handswitch - Triverse Coag" {
        w1260 = FALSE  # Conn2/DIO_7
        w1259 = FALSE  # Conn2/DIO_6
        w1258 = TRUE  # Conn2/DIO_2
        w1257 = FALSE  # Conn2/DIO_1
        w1256 = FALSE  # Conn2/DIO_0
        w1262 = u16 0  # Conn2/DIO_32_39 - uSec Off
        w1263 = bool[] [FALSE, FALSE, FALSE, FALSE, FALSE, FALSE, FALSE, FALSE]  # Conn2/DIO_32_39 In
        w1264 = u16 0  # Conn2/DIO_32_39 - uSec On
        w1265 = FALSE  # Conn2/DIO_32_39 - 75kHz
        w1266 = u16 0  # Conn2/DIO_24_31 - uSec Off
        w1267 = bool[] [FALSE, FALSE, FALSE, FALSE, FALSE, FALSE, FALSE, FALSE]  # Conn2/DIO_24_31 In
        w1268 = u16 0  # Conn2/DIO_24_31 - uSec On
        w1269 = FALSE  # Conn2/DIO_24_31 - 75kHz
        w1270 = u16 0  # Conn2/DIO_16_23 - uSec Off
        w1271 = bool[] [FALSE, FALSE, FALSE, FALSE, FALSE, FALSE, FALSE, FALSE]  # Conn2/DIO_16_23 In
        w1272 = u16 0  # Conn2/DIO_16_23 - uSec On
        w1273 = FALSE  # Conn2/DIO_16_23 - 75kHz
        w1274 = u16 6  # Conn2/DIO_8_15 - uSec Off
        w1275 = bool[] [TRUE, FALSE, TRUE, FALSE, FALSE, FALSE, FALSE, FALSE]  # Conn2/DIO_8_15 In
        w1276 = u16 7  # Conn2/DIO_8_15 - uSec On
        w1277 = TRUE  # Conn2/DIO_8_15 - 75kHz
        w1278 = i16 0  # Connector0/AO7
        w1279 = i16 0  # Connector0/AO6
        w1280 = i16 0  # Connector0/AO5
        w1281 = i16 0  # Connector0/AO4
        w1282 = i16 0  # Connector0/AO3
        w1283 = i16 0  # Connector0/AO2
        w1284 = i16 0  # Connector0/AO1
        w1285 = i16 0  # Connector0/AO0
        w1286 = u16 0  # Conn1/DIO_32_39 - uSec Off
        w1287 = bool[] [FALSE, FALSE, FALSE, FALSE, FALSE, FALSE, FALSE, FALSE]  # Conn1/DIO_32_39 In
        w1288 = u16 0  # Conn1/DIO_32_39 - uSec On
        w1289 = FALSE  # Conn1/DIO_32_39 - 75kHz
        w1290 = u16 0  # Conn1/DIO_24_31 - uSec Off
        w1291 = bool[] [FALSE, FALSE, FALSE, FALSE, FALSE, FALSE, FALSE, FALSE]  # Conn1/DIO_24_31 In
        w1292 = u16 0  # Conn1/DIO_24_31 - uSec On
        w1293 = FALSE  # Conn1/DIO_24_31 - 75kHz
        w1294 = u16 6  # Conn1/DIO_16_23 - uSec Off
        w1295 = bool[] [FALSE, TRUE, FALSE, FALSE, FALSE, FALSE, FALSE, FALSE]  # Conn1/DIO_16_23 In
        w1296 = u16 7  # Conn1/DIO_16_23 - uSec On
        w1297 = TRUE  # Conn1/DIO_16_23 - 75kHz
        w1298 = u16 6  # Conn1/DIO_8_15 - uSec Off
        w1299 = bool[] [FALSE, FALSE, FALSE, TRUE, FALSE, FALSE, FALSE, FALSE]  # Conn1/DIO_8_15 In
        w1300 = u16 7  # Conn1/DIO_8_15 - uSec On
        w1301 = TRUE  # Conn1/DIO_8_15 - 75kHz
        w1302 = u16 0  # Conn0/DIO_8_15 - uSec Off
        w1303 = bool[] [FALSE, FALSE, FALSE, FALSE, FALSE, FALSE, FALSE, FALSE]  # Conn0/DIO_8_15 In
        w1304 = u16 0  # Conn0/DIO_8_15 - uSec On
        w1305 = FALSE  # Conn0/DIO_8_15 - 75kHz
        w1321 = u16 0  # Conn0/DIO_0_7 - uSec Off
        w1320 = bool[] [FALSE, FALSE, FALSE, FALSE, FALSE, FALSE, FALSE, FALSE]  # Conn0/DIO_0_7 In
        w1319 = u16 0  # Conn0/DIO_0_7 - uSec On
        w1318 = FALSE  # Conn0/DIO_0_7 - 75kHz
        w1317 = u16 6  # Conn1/DIO_0_7 - uSec Off
        w1316 = bool[] [FALSE, TRUE, TRUE, TRUE, TRUE, FALSE, FALSE, TRUE]  # Conn1/DIO_0_7 In
        w1315 = u16 7  # Conn1/DIO_0_7 - uSec On
        w1314 = TRUE  # Conn1/DIO_0_7 - 75kHz
        w1313 = u16 6  # Conn2/DIO_0_7 - uSec Off
        w1312 = u16 7  # Conn2/DIO_0_7 - uSec On
        w1311 = TRUE  # Conn2/DIO_0_7 - 75kHz
        # "Handswitch - Triverse Coag"
        # "Handswitch - Triverse Coag"
        # "Handswitch - Triverse Coag"
        n102 = Build Array(w1256, w1257, w1258, w1254, w1253, w1252, w1259, w1260) -> (w1255:bool[])
        n103 = Bundle By Name(cluster=T4 {"Conn0/DIO_0_7 In"={"Conn0/DIO_0_7 - 75kHz"=FALSE, "Conn0/DIO_0_7 - uSec On"=0, "Conn0/DIO_0_7 In"=[FALSE, FALSE, FALSE, FALSE, FALSE, FALSE, FALSE, FALSE], "Conn0/DIO_0_7 - uSec Off"=0}, "Conn0/DIO_8_15 In"={"Conn0/DIO_8_15 - 75kHz"=FALSE, "Conn0/DIO_8_15 - uSec On"=0, "Conn0/DIO_8_15 In"=[FALSE, FALSE, FALSE, FALSE, FALSE, FALSE, FALSE, FALSE], "Conn0/DIO_8_15 - uSec Off"=0}} ("Conn0 DIOs In"), "Conn0/DIO_0_7 In.Conn0/DIO_0_7 - 75kHz"=w1318, "Conn0/DIO_0_7 In.Conn0/DIO_0_7 - uSec On"=w1319, "Conn0/DIO_0_7 In.Conn0/DIO_0_7 In"=w1320, "Conn0/DIO_0_7 In.Conn0/DIO_0_7 - uSec Off"=w1321, "Conn0/DIO_8_15 In.Conn0/DIO_8_15 - 75kHz"=w1305, "Conn0/DIO_8_15 In.Conn0/DIO_8_15 - uSec On"=w1304, "Conn0/DIO_8_15 In.Conn0/DIO_8_15 In"=w1303, "Conn0/DIO_8_15 In.Conn0/DIO_8_15 - uSec Off"=w1302) -> (w1309:T4)
        n104 = Bundle By Name(cluster=T3 {"Conn1/DIO_0_7 In"={"Conn1/DIO_0_7 - 75kHz"=FALSE, "Conn1/DIO_0_7 - uSec On"=0, "Conn1/DIO_0_7 In"=[FALSE, FALSE, FALSE, FALSE, FALSE, FALSE, FALSE, FALSE], "Conn1/DIO_0_7 - uSec Off"=0}, "Conn1/DIO_8_15 In"={"Conn1/DIO_8_15 - 75kHz"=FALSE, "Conn1/DIO_8_15 - uSec On"=0, "Conn1/DIO_8_15 In"=[FALSE, FALSE, FALSE, FALSE, FALSE, FALSE, FALSE, FALSE], "Conn1/DIO_8_15 - uSec Off"=0}, "Conn1/DIO_16_23 In"={"Conn1/DIO_16_23 - 75kHz"=FALSE, "Conn1/DIO_16_23 - uSec On"=0, "Conn1/DIO_16_23 In"=[FALSE, FALSE, FALSE, FALSE, FALSE, FALSE, FALSE, FALSE], "Conn1/DIO_16_23 - uSec Off"=0}, "Conn1/DIO_24_31 In"={"Conn1/DIO_24_31 - 75kHz"=FALSE, "Conn1/DIO_24_31 - uSec On"=0, "Conn1/DIO_24_31 In"=[FALSE, FALSE, FALSE, FALSE, FALSE, FALSE, FALSE, FALSE], "Conn1/DIO_24_31 - uSec Off"=0}, "Conn1/DIO_32_39 In"={"Conn1/DIO_32_39 - 75kHz"=FALSE, "Conn1/DIO_32_39 - uSec On"=0, "Conn1/DIO_32_39 In"=[FALSE, FALSE, FALSE, FALSE, FALSE, FALSE, FALSE, FALSE], "Conn1/DIO_32_39 - uSec Off"=0}} ("Conn1 DIOs In"), "Conn1/DIO_0_7 In.Conn1/DIO_0_7 - 75kHz"=w1314, "Conn1/DIO_0_7 In.Conn1/DIO_0_7 - uSec On"=w1315, "Conn1/DIO_0_7 In.Conn1/DIO_0_7 In"=w1316, "Conn1/DIO_0_7 In.Conn1/DIO_0_7 - uSec Off"=w1317, "Conn1/DIO_8_15 In.Conn1/DIO_8_15 - 75kHz"=w1301, "Conn1/DIO_8_15 In.Conn1/DIO_8_15 - uSec On"=w1300, "Conn1/DIO_8_15 In.Conn1/DIO_8_15 In"=w1299, "Conn1/DIO_8_15 In.Conn1/DIO_8_15 - uSec Off"=w1298, "Conn1/DIO_16_23 In.Conn1/DIO_16_23 - 75kHz"=w1297, "Conn1/DIO_16_23 In.Conn1/DIO_16_23 - uSec On"=w1296, "Conn1/DIO_16_23 In.Conn1/DIO_16_23 In"=w1295, "Conn1/DIO_16_23 In.Conn1/DIO_16_23 - uSec Off"=w1294, "Conn1/DIO_24_31 In.Conn1/DIO_24_31 - 75kHz"=w1293, "Conn1/DIO_24_31 In.Conn1/DIO_24_31 - uSec On"=w1292, "Conn1/DIO_24_31 In.Conn1/DIO_24_31 In"=w1291, "Conn1/DIO_24_31 In.Conn1/DIO_24_31 - uSec Off"=w1290, "Conn1/DIO_32_39 In.Conn1/DIO_32_39 - 75kHz"=w1289, "Conn1/DIO_32_39 In.Conn1/DIO_32_39 - uSec On"=w1288, "Conn1/DIO_32_39 In.Conn1/DIO_32_39 In"=w1287, "Conn1/DIO_32_39 In.Conn1/DIO_32_39 - uSec Off"=w1286) -> (w1322:T3)
        n105 = Bundle By Name(cluster=T2 {"Conn2/DIO_0_7 In"={"Conn2/DIO_0_7 - 75kHz"=FALSE, "Conn2/DIO_0_7 - uSec On"=0, "Conn2/DIO_0_7 In"=[FALSE, FALSE, FALSE, FALSE, FALSE, FALSE, FALSE, FALSE], "Conn2/DIO_0_7 - uSec Off"=0}, "Conn2/DIO_8_15 In"={"Conn2/DIO_8_15 - 75kHz"=FALSE, "Conn2/DIO_8_15 - uSec On"=0, "Conn2/DIO_8_15 In"=[FALSE, FALSE, FALSE, FALSE, FALSE, FALSE, FALSE, FALSE], "Conn2/DIO_8_15 - uSec Off"=0}, "Conn2/DIO_16_23 In"={"Conn2/DIO_16_23 - 75kHz"=FALSE, "Conn2/DIO_16_23 - uSec On"=0, "Conn2/DIO_16_23 In"=[FALSE, FALSE, FALSE, FALSE, FALSE, FALSE, FALSE, FALSE], "Conn2/DIO_16_23 - uSec Off"=0}, "Conn2/DIO_24_31 In"={"Conn2/DIO_24_31 - 75kHz"=FALSE, "Conn2/DIO_24_31 - uSec On"=0, "Conn2/DIO_24_31 In"=[FALSE, FALSE, FALSE, FALSE, FALSE, FALSE, FALSE, FALSE], "Conn2/DIO_24_31 - uSec Off"=0}, "Conn2/DIO_32_39 In"={"Conn2/DIO_32_39 - 75kHz"=FALSE, "Conn2/DIO_32_39 - uSec On"=0, "Conn2/DIO_32_39 In"=[FALSE, FALSE, FALSE, FALSE, FALSE, FALSE, FALSE, FALSE], "Conn2/DIO_32_39 - uSec Off"=0}} ("Conn2 DIOs In"), "Conn2/DIO_0_7 In.Conn2/DIO_0_7 - 75kHz"=w1311, "Conn2/DIO_0_7 In.Conn2/DIO_0_7 - uSec On"=w1312, "Conn2/DIO_0_7 In.Conn2/DIO_0_7 In"=w1255, "Conn2/DIO_0_7 In.Conn2/DIO_0_7 - uSec Off"=w1313, "Conn2/DIO_8_15 In.Conn2/DIO_8_15 - 75kHz"=w1277, "Conn2/DIO_8_15 In.Conn2/DIO_8_15 - uSec On"=w1276, "Conn2/DIO_8_15 In.Conn2/DIO_8_15 In"=w1275, "Conn2/DIO_8_15 In.Conn2/DIO_8_15 - uSec Off"=w1274, "Conn2/DIO_16_23 In.Conn2/DIO_16_23 - 75kHz"=w1273, "Conn2/DIO_16_23 In.Conn2/DIO_16_23 - uSec On"=w1272, "Conn2/DIO_16_23 In.Conn2/DIO_16_23 In"=w1271, "Conn2/DIO_16_23 In.Conn2/DIO_16_23 - uSec Off"=w1270, "Conn2/DIO_24_31 In.Conn2/DIO_24_31 - 75kHz"=w1269, "Conn2/DIO_24_31 In.Conn2/DIO_24_31 - uSec On"=w1268, "Conn2/DIO_24_31 In.Conn2/DIO_24_31 In"=w1267, "Conn2/DIO_24_31 In.Conn2/DIO_24_31 - uSec Off"=w1266, "Conn2/DIO_32_39 In.Conn2/DIO_32_39 - 75kHz"=w1265, "Conn2/DIO_32_39 In.Conn2/DIO_32_39 - uSec On"=w1264, "Conn2/DIO_32_39 In.Conn2/DIO_32_39 In"=w1263, "Conn2/DIO_32_39 In.Conn2/DIO_32_39 - uSec Off"=w1262) -> (w1323:T2)
        n106 = Build Array(w1285, w1284, w1283, w1282, w1281, w1280, w1279, w1278) -> (w1324:i16[])
        n107 = xnode "Read/Write Control"("FPGA VI Reference In"=w1306, "Conn0 DIOs In"=w1309, "Conn1 DIOs In"=w1322, "Conn2 DIOs In"=w1323, "Connector0/AO0_7"=w1324) -> ("FPGA VI Reference Out"=w1307:refnum<k20>)  [unwired: 1 in, 1 out]
      }
    }
  }
  "Refnum out" <- w3
